vi "Parser.vi"() -> ()   [LabVIEW 2010]
panel:
  out "array of clusters 2":cluster{string[]}[](array[cluster])
  in  "Ring":u16(ring) items=["cp", "ct", "dd", "ep", "io", "ip", "pd", "pp", "ss", "st", "tp", "up", "vp"]
  out "Группы":string[](array[string])
  out "Параметры 2":T1(array[cluster])=[{"Имя"="cp1", "Группа"="cp", "Наименование"="Пропорциональный коэффициент контура тока", "Ед. изм"=0, "Список"="", "Адрес"=0, "Описание"="Параметр настройки ПИ-регулятора контура тока", "Мин"=0, "Макс"=100, "Сервис"=TRUE, "Только чтение"=FALSE, "Разработка"=FALSE, "К-во бит"=32, "Шаг"=12, "Обработка"=FALSE, "Макрос"=""}, {"Имя"="cp10", "Группа"="cp", "Наименование"="Номинальный ток", "Ед. изм"=5, "Список"="", "Адрес"=2069, "Описание"="", "Мин"=0, "Макс"=850, "Сервис"=TRUE, "Только чтение"=FALSE, "Разработка"=FALSE, "К-во бит"=32, "Шаг"=16, "Обработка"=TRUE, "Макрос"="macros cp10\n  ON_READ\n  READ cp3\n  cp3=cp3*5/2047\n  RETURN cp3\n  ON_WRITE\n  cp3=val*66\n  WRITE cp3\nend"}, {"Имя"="cp11", "Группа"="cp", "Наименование"="Коэффициент ФНЧ входного сигнала", "Ед. изм"=0, "Список"="", "Адрес"=2081, "Описание"="Коэффициент ФНЧ входного сигнала контура тока.", "Мин"=0, "Макс"=1, "Сервис"=TRUE, "Только чтение"=FALSE, "Разработка"=FALSE, "К-во бит"=32, "Шаг"=12, "Обработка"=FALSE, "Макрос"=""}, {"Имя"="cp12", "Группа"="cp", "Наименование"="Коэффициент ФНЧ сигнала ОС", "Ед. изм"=0, "Список"="", "Адрес"=2082, "Описание"="Коэффициент ФНЧ сигнала обратной связи контура тока.", "Мин"=0, "Макс"=1, "Сервис"=TRUE, "Только чтение"=FALSE, "Разработка"=FALSE, "К-во бит"=32, "Шаг"=12, "Обработка"=FALSE, "Макрос"=""}, {"Имя"="cp2", "Группа"="cp", "Наименование"="Интегральный коэффициент контура тока", "Ед. изм"=0, "Список"="", "Адрес"=2, "Описание"="Параметр настройки ПИ-регулятора контура тока", "Мин"=0, "Макс"=200, "Сервис"=TRUE, "Только чтение"=FALSE, "Разработка"=FALSE, "К-во бит"=32, "Шаг"=12, "Обработка"=FALSE, "Макрос"=""}, {"Имя"="cp3", "Группа"="cp", "Наименование"="Максимальный ток", "Ед. изм"=1, "Список"="", "Адрес"=4, "Описание"="Определять предельную величину тока допустимую для двигателя.", "Мин"=0, "Макс"=1500, "Сервис"=FALSE, "Только чтение"=FALSE, "Разработка"=FALSE, "К-во бит"=16, "Шаг"=0, "Обработка"=TRUE, "Макрос"="macros cp3\n  ON_READ\n  READ cp3\n  cp3=cp3*5/2047\n  RETURN cp3\n  ON_WRITE\n  cp3=val*2047/5\n  WRITE cp3\nend"}, {"Имя"="cp4", "Группа"="cp", "Наименование"="Максимальная скваженность ШИМ", "Ед. изм"=1, "Список"="", "Адрес"=5, "Описание"="3070 дискрет соответствует 100% заполнения", "Мин"=0, "Макс"=6150, "Сервис"=FALSE, "Только чтение"=FALSE, "Разработка"=FALSE, "К-во бит"=16, "Шаг"=0, "Обработка"=TRUE, "Макрос"="macros cp4\n  ON_READ\n  READ cp4\n  cp4=cp4*5/2500\n  RETURN cp4\n  ON_WRITE\n  cp4=val*2500/5\n  WRITE cp4\nend"}, {"Имя"="cp5", "Группа"="cp", "Наименование"="Состояние контура тока", "Ед. изм"=0, "Список"="0:Разомкнут\n2:Замкнут\n4:Прямое управление токами в обмотках\n5:Адаптивное упрваление\n6:Прямое раздельное управление токами в обмотках\n\r\n", "Адрес"=16, "Описание"="Обеспечивает замкнутое или разомкнутое регулирование контура тока. В стандартном режиме использования контур должен быть замкнут.", "Мин"=0, "Макс"=6, "Сервис"=FALSE, "Только чтение"=FALSE, "Разработка"=FALSE, "К-во бит"=16, "Шаг"=0, "Обработка"=FALSE, "Макрос"=""}, {"Имя"="cp6", "Группа"="cp", "Наименование"="Вырабатываемый момент", "Ед. изм"=0, "Список"="100:100%\n75:75%\n50:50%\n25:25%\n\r\n", "Адрес"=72, "Описание"="Параметр позволяет ограничить развиваемый момент", "Мин"=25, "Макс"=100, "Сервис"=FALSE, "Только чтение"=FALSE, "Разработка"=TRUE, "К-во бит"=16, "Шаг"=0, "Обработка"=FALSE, "Макрос"=""}, {"Имя"="cp7", "Группа"="cp", "Наименование"="Модуляция ШИМ сигнала", "Ед. изм"=0, "Список"="0:Выключена\n1:Включена\n\r\n", "Адрес"=83, "Описание"="Разрешает/запрещает подачу силового напряжения на обмотки двигателя", "Мин"=0, "Макс"=1, "Сервис"=FALSE, "Только чтение"=FALSE, "Разработка"=FALSE, "К-во бит"=16, "Шаг"=0, "Обработка"=FALSE, "Макрос"=""}, {"Имя"="cp8", "Группа"="cp", "Наименование"="Частота ШИМ сигнала", "Ед. изм"=12, "Список"="2500:40кГц\n5000:20кГц\n6250:16кГц\n12500:8кГц\n25000:4кГц\n\r\n", "Адрес"=96, "Описание"="Определяет частоту ШИМ сигнала и частоту работы контура тока. Влияет на КПД силовой части привода, а также качество работы контура тока. Для приводов серии СПШ частота всегда 40кГц. Влияет на параметр cp4.", "Мин"=-65535, "Макс"=65535, "Сервис"=FALSE, "Только чтение"=FALSE, "Разработка"=FALSE, "К-во бит"=16, "Шаг"=0, "Обработка"=FALSE, "Макрос"=""}, {"Имя"="cp9", "Группа"="cp", "Наименование"="Допустимая перегрузка", "Ед. изм"=13, "Список"="", "Адрес"=2068, "Описание"="Ограничение выделяемой мощности обмотками двигателя. Предотвращает повреждения обмоток. Реализует защитную функцию I2t", "Мин"=0, "Макс"=350, "Сервис"=TRUE, "Только чтение"=FALSE, "Разработка"=FALSE, "К-во бит"=32, "Шаг"=16, "Обработка"=FALSE, "Макрос"=""}, {"Имя"="ct1", "Группа"="ct", "Наименование"="Задание тока", "Ед. изм"=5, "Список"="", "Адрес"=512, "Описание"="Сигнал управления при разомкнутом контуре скорости и положения", "Мин"=-3500, "Макс"=3500, "Сервис"=FALSE, "Только чтение"=FALSE, "Разработка"=FALSE, "К-во бит"=16, "Шаг"=0, "Обработка"=TRUE, "Макрос"="macros ct1\n  ON_READ\n  READ ct1\n  ct1=ct1*5/2500\n  RETURN ct1\n  ON_WRITE\n  ct1=val*2500/5\n  WRITE ct1\nend"}, {"Имя"="ct2", "Группа"="ct", "Наименование"="Задание скорости", "Ед. изм"=4, "Список"="", "Адрес"=514, "Описание"="Сигнал управления при разомкнутом контуре положения", "Мин"=-12000, "Макс"=12000, "Сервис"=TRUE, "Только чтение"=FALSE, "Разработка"=FALSE, "К-во бит"=32, "Шаг"=12, "Обработка"=FALSE, "Макрос"=""}, {"Имя"="ct3", "Группа"="ct", "Наименование"="Задание положения", "Ед. изм"=6, "Список"="", "Адрес"=516, "Описание"="Сигнал управления при замкнутом контуре положения", "Мин"=-2147483647, "Макс"=2147483647, "Сервис"=FALSE, "Только чтение"=FALSE, "Разработка"=FALSE, "К-во бит"=32, "Шаг"=0, "Обработка"=FALSE, "Макрос"=""}, {"Имя"="dd1", "Группа"="dd", "Наименование"="Ток в обмотке 1", "Ед. изм"=5, "Список"="", "Адрес"=1024, "Описание"="Показывает ток, протекающий в обмотке двигателя", "Мин"=-5, "Макс"=5, "Сервис"=FALSE, "Только чтение"=TRUE, "Разработка"=FALSE, "К-во бит"=16, "Шаг"=0, "Обработка"=TRUE, "Макрос"="macros dd1\n  ON_READ\n  READ dd1\n  dd1=dd1*5/2047\n  RETURN dd1\n  ON_WRITE\n  dd1=val*2047/5\n  WRITE dd1\nend"}, {"Имя"="dd10", "Группа"="dd", "Наименование"="Температура внутри корпуса", "Ед. изм"=7, "Список"="", "Адрес"=1038, "Описание"="", "Мин"=-40, "Макс"=120, "Сервис"=FALSE, "Только чтение"=TRUE, "Разработка"=FALSE, "К-во бит"=16, "Шаг"=0, "Обработка"=TRUE, "Макрос"="macros dd10\n  ON_READ\n  READ dd10\n  dd10=dd10/128\n  RETURN dd10\n  ON_WRITE\n  dd10=val\n  WRITE dd10\nend"}, {"Имя"="dd11", "Группа"="dd", "Наименование"="Статус контроллера", "Ед. изм"=0, "Список"="0:Исправен\n1:Останов по команде\n2:Останов - высокое противодействующее усилие\n3:Останов - короткое замыкание\n4:Выход из температурного диапазона\n5:Повышенное силовое напряжение\n6:Низкое силовое напряжение\n7:Повышенное цифровое напряжение\n8:Низкое цифровое напряжение\n9:Cиловое напряжение превышает напряжение, установл. пользователем\n10:Останов - превышение допустимой перегрузки\n11:Останов - сработала защита IGBT модуля\n12:Останов - Ошибка поиска фазы по UVW трекам\n13:Останов - ошибка в настройках энкодера\n14: Останов - сбой в работе энкодера\n15: Останов - Ошибка фазировки двигателя\n\r\n", "Адрес"=1039, "Описание"="Привод в состоянии отработать задание только, если его статус \"Исправен\".", "Мин"=0, "Макс"=15, "Сервис"=FALSE, "Только чтение"=FALSE, "Разработка"=FALSE, "К-во бит"=16, "Шаг"=0, "Обработка"=FALSE, "Макрос"=""}, {"Имя"="dd12", "Группа"="dd", "Наименование"="Текущее напряжение питания", "Ед. изм"=8, "Список"="", "Адрес"=1040, "Описание"="", "Мин"=0, "Макс"=120, "Сервис"=FALSE, "Только чтение"=TRUE, "Разработка"=FALSE, "К-во бит"=16, "Шаг"=0, "Обработка"=TRUE, "Макрос"="macros dd12\n  ON_READ\n  READ dd12\n  dd12=dd12/21\n  RETURN dd12\n  ON_WRITE\n  dd12=val\n  WRITE dd12\nend"}, {"Имя"="dd13", "Группа"="dd", "Наименование"="Тестовый параметр 1", "Ед. изм"=0, "Список"="", "Адрес"=1041, "Описание"="Пока используется для индикации перехода на меандр вместо синуса. Параметр для разработчика", "Мин"=-65535, "Макс"=65535, "Сервис"=FALSE, "Только чтение"=TRUE, "Разработка"=TRUE, "К-во бит"=16, "Шаг"=0, "Обработка"=FALSE, "Макрос"=""}, {"Имя"="dd14", "Группа"="dd", "Наименование"="Тестовый параметр 2", "Ед. изм"=0, "Список"="", "Адрес"=1042, "Описание"="Пока используется для индикации сдвига фазы", "Мин"=-65535, "Макс"=65535, "Сервис"=FALSE, "Только чтение"=TRUE, "Разработка"=TRUE, "К-во бит"=16, "Шаг"=0, "Обработка"=FALSE, "Макрос"=""}, {"Имя"="dd15", "Группа"="dd", "Наименование"="Время выполнения команды интерпретатором", "Ед. изм"=11, "Список"="", "Адрес"=1043, "Описание"="Определяет максимальное время, которое интерпретатор затрачивает на выполнение команды в текущей программе.", "Мин"=0, "Макс"=2147483647, "Сервис"=FALSE, "Только чтение"=TRUE, "Разработка"=FALSE, "К-во бит"=32, "Шаг"=1, "Обработка"=TRUE, "Макрос"="macros dd15\n  ON_READ\n  READ dd15\n  dd15=dd15*25/1000\n  RETURN dd15\n  ON_WRITE\n  dd15=val\n  WRITE dd15\nend"}, {"Имя"="dd16", "Группа"="dd", "Наименование"="Время выполнения программы интерпретатором", "Ед. изм"=11, "Список"="", "Адрес"=1044, "Описание"="Определяет максимальное время, которое интерпретатор затрачивает на выполнение всей программы.", "Мин"=0, "Макс"=2147483647, "Сервис"=FALSE, "Только чтение"=TRUE, "Разработка"=FALSE, "К-во бит"=32, "Шаг"=1, "Обработка"=TRUE, "Макрос"="macros dd16\n  ON_READ\n  READ dd16\n  dd16=dd16*25/1000\n  RETURN dd16\n  ON_WRITE\n  dd16=val\n  WRITE dd16\nend"}, {"Имя"="dd17", "Группа"="dd", "Наименование"="Аналоговый вход 0", "Ед. изм"=1, "Список"="", "Адрес"=1045, "Описание"="", "Мин"=-65535, "Макс"=65535, "Сервис"=FALSE, "Только чтение"=TRUE, "Разработка"=FALSE, "К-во бит"=16, "Шаг"=0, "Обработка"=FALSE, "Макрос"=""}, {"Имя"="dd18", "Группа"="dd", "Наименование"="Аналоговый вход 1", "Ед. изм"=1, "Список"="", "Адрес"=1046, "Описание"="", "Мин"=-65535, "Макс"=65535, "Сервис"=FALSE, "Только чтение"=TRUE, "Разработка"=FALSE, "К-во бит"=16, "Шаг"=0, "Обработка"=FALSE, "Макрос"=""}, {"Имя"="dd19", "Группа"="dd", "Наименование"="Текущее цифровое напряжение", "Ед. изм"=8, "Список"="", "Адрес"=1047, "Описание"="", "Мин"=0, "Макс"=23, "Сервис"=FALSE, "Только чтение"=TRUE, "Разработка"=FALSE, "К-во бит"=16, "Шаг"=0, "Обработка"=TRUE, "Макрос"="macros dd19\n  ON_READ\n  READ dd19\n  dd19=dd19/178\n  RETURN dd19\n  ON_WRITE\n  dd19=val\n  WRITE dd19\nend"}, {"Имя"="dd2", "Группа"="dd", "Наименование"="Заданный ток в роторной системе координат", "Ед. изм"=5, "Список"="", "Адрес"=1026, "Описание"="Индицирует ток, который задан контуром скорости", "Мин"=-5, "Макс"=5, "Сервис"=FALSE, "Только чтение"=TRUE, "Разработка"=FALSE, "К-во бит"=16, "Шаг"=0, "Обработка"=TRUE, "Макрос"="macros dd2\n  ON_READ\n  READ dd2\n  dd2=dd2*5/2047\n  RETURN dd2\n  ON_WRITE\n  dd2=val*2047/5\n  WRITE dd2\nend"}, {"Имя"="dd20", "Группа"="dd", "Наименование"="Ошибка контура позиции", "Ед. изм"=6, "Список"="", "Адрес"=1048, "Описание"="", "Мин"=-2147483647, "Макс"=2147483647, "Сервис"=TRUE, "Только чтение"=TRUE, "Разработка"=FALSE, "К-во бит"=32, "Шаг"=10, "Обработка"=FALSE, "Макрос"=""}, {"Имя"="dd21", "Группа"="dd", "Наименование"="Ошибка контура скорости", "Ед. изм"=4, "Список"="", "Адрес"=1049, "Описание"="", "Мин"=-65535, "Макс"=65535, "Сервис"=FALSE, "Только чтение"=TRUE, "Разработка"=FALSE, "К-во бит"=16, "Шаг"=1, "Обработка"=FALSE, "Макрос"=""}, {"Имя"="dd22", "Группа"="dd", "Наименование"="Максимальное отклонение от траектории", "Ед. изм"=1, "Список"="", "Адрес"=1056, "Описание"="Определяет максимальную ошибку контура позиции зафиксированную при прохождении траектории.", "Мин"=0, "Макс"=65535, "Сервис"=FALSE, "Только чтение"=FALSE, "Разработка"=FALSE, "К-во бит"=16, "Шаг"=0, "Обработка"=FALSE, "Макрос"=""}, {"Имя"="dd23", "Группа"="dd", "Наименование"="Статус G декодера", "Ед. изм"=0, "Список"="0:Останов\n1:Начало\n2:Отработка\n3:Ожидание подтверждений\n4:Ошибка\n5:Выход в нуль\r\n", "Адрес"=1057, "Описание"="", "Мин"=0, "Макс"=5, "Сервис"=FALSE, "Только чтение"=TRUE, "Разработка"=TRUE, "К-во бит"=16, "Шаг"=0, "Обработка"=FALSE, "Макрос"=""}, {"Имя"="dd24", "Группа"="dd", "Наименование"="Текущий кадр G декодера", "Ед. изм"=0, "Список"="", "Адрес"=1058, "Описание"="", "Мин"=0, "Макс"=65535, "Сервис"=FALSE, "Только чтение"=TRUE, "Разработка"=TRUE, "К-во бит"=16, "Шаг"=0, "Обработка"=FALSE, "Макрос"=""}, {"Имя"="dd25", "Группа"="dd", "Наименование"="UVW треки", "Ед. изм"=0, "Список"="", "Адрес"=1059, "Описание"="Сигнал, считанный с UVW треков энкодера", "Мин"=0, "Макс"=16, "Сервис"=FALSE, "Только чтение"=TRUE, "Разработка"=FALSE, "К-во бит"=16, "Шаг"=0, "Обработка"=FALSE, "Макрос"=""}, {"Имя"="dd26", "Группа"="dd", "Наименование"="Текущая перегрузка", "Ед. изм"=13, "Список"="", "Адрес"=1060, "Описание"="Накомпленнае мощность, превышающая номинальные характеристики двигателя", "Мин"=0, "Макс"=100, "Сервис"=TRUE, "Только чтение"=TRUE, "Разработка"=FALSE, "К-во бит"=32, "Шаг"=16, "Обработка"=FALSE, "Макрос"=""}, {"Имя"="dd27", "Группа"="dd", "Наименование"="Ток в обмотке 3", "Ед. изм"=5, "Список"="", "Адрес"=1061, "Описание"="Показывает ток, протекающий в обмотке двигателя. Параметр действителен только для СПС.", "Мин"=-5, "Макс"=5, "Сервис"=FALSE, "Только чтение"=TRUE, "Разработка"=FALSE, "К-во бит"=16, "Шаг"=0, "Обработка"=TRUE, "Макрос"="macros dd27\n  ON_READ\n  READ dd1\n  dd1=dd1*5/2047\n  RETURN dd1\n  ON_WRITE\n  dd1=val*2047/5\n  WRITE dd1\nend"}, {"Имя"="dd28", "Группа"="dd", "Наименование"="Заданный ток в обмотке 3", "Ед. изм"=5, "Список"="", "Адрес"=1062, "Описание"="Заданный ток в обмотке 3. Действителен только для приводов серии СПС.", "Мин"=-2047, "Макс"=2047, "Сервис"=FALSE, "Только чтение"=FALSE, "Разработка"=FALSE, "К-во бит"=16, "Шаг"=0, "Обработка"=TRUE, "Макрос"="macros dd28\n  ON_READ\n  READ dd6\n  dd6=dd6/74\n  RETURN dd6\n  ON_WRITE\n  dd6=val*74\n  WRITE dd6\nend"}, {"Имя"="dd29", "Группа"="dd", "Наименование"="Ток потребления двигателя", "Ед. изм"=5, "Список"="", "Адрес"=1063, "Описание"="Параметр действителен только для СПС.", "Мин"=-5, "Макс"=5, "Сервис"=FALSE, "Только чтение"=TRUE, "Разработка"=FALSE, "К-во бит"=16, "Шаг"=0, "Обработка"=TRUE, "Макрос"="macros dd29\n  ON_READ\n  READ dd1\n  dd1=dd1/74\n  RETURN dd1\n  ON_WRITE\n  dd1=val*74\n  WRITE dd1\nend"}, {"Имя"="dd3", "Группа"="dd", "Наименование"="Ток в обмотке 2", "Ед. изм"=5, "Список"="", "Адрес"=1029, "Описание"="Индицирует ток, протекающий в обмотке двигателя", "Мин"=-5, "Макс"=5, "Сервис"=FALSE, "Только чтение"=TRUE, "Разработка"=FALSE, "К-во бит"=16, "Шаг"=0, "Обработка"=TRUE, "Макрос"="macros dd3\n  ON_READ\n  READ dd3\n  dd3=dd3*5/2047\n  RETURN dd3\n  ON_WRITE\n  dd3=val*2047/5\n  WRITE dd3\nend"}, {"Имя"="dd30", "Группа"="dd", "Наименование"="Разница между внешним и внутренним энкодерами", "Ед. изм"=1, "Список"="", "Адрес"=1064, "Описание"="Разница между внешним и внутренним энкодерами с приведением к разрешению внутреннего", "Мин"=-524286, "Макс"=524286, "Сервис"=TRUE, "Только чтение"=TRUE, "Разработка"=FALSE, "К-во бит"=32, "Шаг"=12, "Обработка"=FALSE, "Макрос"=""}, {"Имя"="dd31", "Группа"="dd", "Наименование"="Смещение фазы ослабления поля", "Ед. изм"=0, "Список"="", "Адрес"=1065, "Описание"="", "Мин"=0, "Макс"=0, "Сервис"=FALSE, "Только чтение"=TRUE, "Разработка"=FALSE, "К-во бит"=16, "Шаг"=0, "Обработка"=FALSE, "Макрос"=""}, {"Имя"="dd32", "Группа"="dd", "Наименование"="Задержка синхронизации", "Ед. изм"=14, "Список"="", "Адрес"=1066, "Описание"="Время между приемом команды упарвления и команды синхронизации. Параметр действителен только для приоводов с интерфейсом упарвления EtherCAT и при активизации управления от СЧПУ.", "Мин"=0, "Макс"=0, "Сервис"=FALSE, "Только чтение"=TRUE, "Разработка"=FALSE, "К-во бит"=32, "Шаг"=0, "Обработка"=FALSE, "Макрос"=""}, {"Имя"="dd33", "Группа"="dd", "Наименование"="Кол-во импульсов на сектор UVW сигнала", "Ед. изм"=6, "Список"="", "Адрес"=1067, "Описание"="Кол-во импульсов датчика позиции, приходящееся на текущий сектор UVW сигнала.", "Мин"=-2147483647, "Макс"=2147483647, "Сервис"=FALSE, "Только чтение"=TRUE, "Разработка"=FALSE, "К-во бит"=32, "Шаг"=0, "Обработка"=FALSE, "Макрос"=""}, {"Имя"="dd34", "Группа"="dd", "Наименование"="Ток в роторной системе координат", "Ед. изм"=1, "Список"="", "Адрес"=1068, "Описание"="Ток, пересчитанный в роторную систему координат. Данный сигнал является обратной связью на задание ddd2", "Мин"=-2147483647, "Макс"=2147483647, "Сервис"=TRUE, "Только чтение"=TRUE, "Разработка"=FALSE, "К-во бит"=32, "Шаг"=12, "Обработка"=FALSE, "Макрос"=""}, {"Имя"="dd4", "Группа"="dd", "Наименование"="Текущая скорость вращения", "Ед. изм"=4, "Список"="", "Адрес"=1032, "Описание"="", "Мин"=-5000, "Макс"=5000, "Сервис"=FALSE, "Только чтение"=TRUE, "Разработка"=FALSE, "К-во бит"=8, "Шаг"=12, "Обработка"=FALSE, "Макрос"=""}, {"Имя"="dd5", "Группа"="dd", "Наименование"="Заданная скорость вращения", "Ед. изм"=4, "Список"="", "Адрес"=1033, "Описание"="", "Мин"=-5000, "Макс"=5000, "Сервис"=FALSE, "Только чтение"=TRUE, "Разработка"=FALSE, "К-во бит"=16, "Шаг"=12, "Обработка"=FALSE, "Макрос"=""}, {"Имя"="dd6", "Группа"="dd", "Наименование"="Заданный ток в обмотке 1", "Ед. изм"=5, "Список"="", "Адрес"=1034, "Описание"="", "Мин"=-2047, "Макс"=2047, "Сервис"=FALSE, "Только чтение"=FALSE, "Разработка"=FALSE, "К-во бит"=16, "Шаг"=0, "Обработка"=TRUE, "Макрос"="macros dd6\n  ON_READ\n  READ dd6\n  dd6=dd6*5/2047\n  RETURN dd6\n  ON_WRITE\n  dd6=val*2047/5\n  WRITE dd6\nend"}, {"Имя"="dd7", "Группа"="dd", "Наименование"="Заданная позиция", "Ед. изм"=6, "Список"="", "Адрес"=1035, "Описание"="", "Мин"=-2147483647, "Макс"=2147483647, "Сервис"=FALSE, "Только чтение"=TRUE, "Разработка"=FALSE, "К-во бит"=32, "Шаг"=0, "Обработка"=FALSE, "Макрос"=""}, {"Имя"="dd8", "Группа"="dd", "Наименование"="Текущая позиция", "Ед. изм"=6, "Список"="", "Адрес"=1036, "Описание"="", "Мин"=-2147483647, "Макс"=2147483647, "Сервис"=FALSE, "Только чтение"=TRUE, "Разработка"=FALSE, "К-во бит"=32, "Шаг"=0, "Обработка"=FALSE, "Макрос"=""}, {"Имя"="dd9", "Группа"="dd", "Наименование"="Заданный ток в обмотке 2", "Ед. изм"=5, "Список"="", "Адрес"=1037, "Описание"="", "Мин"=-2047, "Макс"=2047, "Сервис"=FALSE, "Только чтение"=FALSE, "Разработка"=FALSE, "К-во бит"=16, "Шаг"=0, "Обработка"=TRUE, "Макрос"="macros dd9\n  ON_READ\n  READ dd9\n  dd9=dd9*5/2047\n  RETURN dd9\n  ON_WRITE\n  dd9=val*2047/5\n  WRITE dd9\nend"}, {"Имя"="ep1", "Группа"="ep", "Наименование"="Режим торможения", "Ед. изм"=0, "Список"="0:Торможение без контроля напряжения\n2:Торможение с контролем напряжения\n\r\n", "Адрес"=67, "Описание"="При торможении без контроля напряжения привод перейдет в аварийное состояние в момент превышения напряжением допустимого значения, установленным в параметре ep2.", "Мин"=0, "Макс"=2, "Сервис"=FALSE, "Только чтение"=FALSE, "Разработка"=FALSE, "К-во бит"=16, "Шаг"=0, "Обработка"=FALSE, "Макрос"=""}, {"Имя"="ep2", "Группа"="ep", "Наименование"="Максимальное напряжение", "Ед. изм"=8, "Список"="", "Адрес"=68, "Описание"="Максимальное допустимое напряжение, при котором привод должен переходить в состояние отключения.", "Мин"=0, "Макс"=280, "Сервис"=FALSE, "Только чтение"=FALSE, "Разработка"=FALSE, "К-во бит"=16, "Шаг"=0, "Обработка"=TRUE, "Макрос"="macros ep2\n  ON_READ\n  READ ep2\n  ep2=ep2/21\n  RETURN ep2\n  ON_WRITE\n  ep2=val*21\n  WRITE ep2\nend"}, {"Имя"="ep3", "Группа"="ep", "Наименование"="Ток поиска фазы", "Ед. изм"=1, "Список"="", "Адрес"=81, "Описание"="Определяет уровень тока, который устанавливается при поиске фазы. Ток задается в дискретах.", "Мин"=0, "Макс"=32000, "Сервис"=FALSE, "Только чтение"=FALSE, "Разработка"=FALSE, "К-во бит"=16, "Шаг"=1, "Обработка"=FALSE, "Макрос"=""}, {"Имя"="ep4", "Группа"="ep", "Наименование"="Время поиска фазы", "Ед. изм"=1, "Список"="", "Адрес"=82, "Описание"="Определяет время, в течение которого будет удерживаться ток ep3 при поиске фазы.", "Мин"=0, "Макс"=32000, "Сервис"=FALSE, "Только чтение"=FALSE, "Разработка"=FALSE, "К-во бит"=16, "Шаг"=1, "Обработка"=FALSE, "Макрос"=""}, {"Имя"="ep5", "Группа"="ep", "Наименование"="Максимальная температура", "Ед. изм"=7, "Список"="", "Адрес"=84, "Описание"="Указывает максимальную допустимую температуру внутри корпуса", "Мин"=25, "Макс"=85, "Сервис"=FALSE, "Только чтение"=FALSE, "Разработка"=FALSE, "К-во бит"=16, "Шаг"=1, "Обработка"=FALSE, "Макрос"=""}, {"Имя"="ep6", "Группа"="ep", "Наименование"="Период поиска фазы", "Ед. изм"=0, "Список"="0:Однопериодный\n1:1\n2:2\n3:3\n\r\n", "Адрес"=86, "Описание"="Один из трех периодов, во время которого привод может выполнять поиск фазы. В результате удается избежать перегрузки источника питания и выполнить корректный поиск фазы в приводах, между которыми имеется жесткая механическая связь.", "Мин"=0, "Макс"=3, "Сервис"=FALSE, "Только чтение"=FALSE, "Разработка"=FALSE, "К-во бит"=16, "Шаг"=1, "Обработка"=FALSE, "Макрос"=""}, {"Имя"="ep7", "Группа"="ep", "Наименование"="Функция контроля зазора", "Ед. изм"=0, "Список"="0:ВЫКЛ\n90:ВКЛ\n\r\n", "Адрес"=2075, "Описание"="Включение данной автоматически запускает внутреннюю программу контроля расстояния между инструментом и обрабатываемым листом.", "Мин"=0, "Макс"=90, "Сервис"=FALSE, "Только чтение"=FALSE, "Разработка"=FALSE, "К-во бит"=16, "Шаг"=1, "Обработка"=FALSE, "Макрос"=""}, {"Имя"="io0", "Группа"="io", "Наименование"="Порт ввода 0", "Ед. изм"=0, "Список"="", "Адрес"=2053, "Описание"="Значение порта ввода 0", "Мин"=0, "Макс"=1, "Сервис"=FALSE, "Только чтение"=FALSE, "Разработка"=FALSE, "К-во бит"=16, "Шаг"=0, "Обработка"=FALSE, "Макрос"=""}, {"Имя"="io1", "Группа"="io", "Наименование"="Порт ввода 1", "Ед. изм"=0, "Список"="", "Адрес"=2054, "Описание"="Значение порта ввода 1", "Мин"=0, "Макс"=1, "Сервис"=FALSE, "Только чтение"=FALSE, "Разработка"=FALSE, "К-во бит"=16, "Шаг"=0, "Обработка"=FALSE, "Макрос"=""}, {"Имя"="io10", "Группа"="io", "Наименование"="Режим порта ввода 2", "Ед. изм"=0, "Список"="0:Порт ввода общего назначения\n1:Порт ввода в режиме квадратурного счетчика\n2:Порт ввода в режиме счетчика Step/dir\n\r\n", "Адрес"=2063, "Описание"="Определяет режим работы порта ввода.", "Мин"=0, "Макс"=3, "Сервис"=FALSE, "Только чтение"=FALSE, "Разработка"=FALSE, "К-во бит"=16, "Шаг"=1, "Обработка"=FALSE, "Макрос"=""}, {"Имя"="io11", "Группа"="io", "Наименование"="Режим порта ввода 3", "Ед. изм"=0, "Список"="0:Порт ввода общего назначения\n1:Порт ввода в режиме квадратурного счетчика\n2:Порт ввода в режиме счетчика Step/dir\n\r\n", "Адрес"=2064, "Описание"="Определяет режим работы порта ввода.", "Мин"=0, "Макс"=3, "Сервис"=FALSE, "Только чтение"=FALSE, "Разработка"=FALSE, "К-во бит"=16, "Шаг"=1, "Обработка"=FALSE, "Макрос"=""}, {"Имя"="io12", "Группа"="io", "Наименование"="Режим порта вывода 0", "Ед. изм"=0, "Список"="0:Порт вывода общего назначения\n1:Порт вывода в режиме ШИМ\n\r\n", "Адрес"=2065, "Описание"="Определяет режим работы порта вывода.", "Мин"=0, "Макс"=3, "Сервис"=FALSE, "Только чтение"=FALSE, "Разработка"=FALSE, "К-во бит"=16, "Шаг"=1, "Обработка"=FALSE, "Макрос"=""}, {"Имя"="io13", "Группа"="io", "Наименование"="Режим порта вывода 1", "Ед. изм"=0, "Список"="0:Порт вывода общего назначения\n1:Порт вывода в режиме ШИМ\n\r\n", "Адрес"=2066, "Описание"="Определяет режим работы порта вывода.", "Мин"=0, "Макс"=3, "Сервис"=FALSE, "Только чтение"=FALSE, "Разработка"=FALSE, "К-во бит"=16, "Шаг"=1, "Обработка"=FALSE, "Макрос"=""}, {"Имя"="io14", "Группа"="io", "Наименование"="Счетчик импульсов", "Ед. изм"=0, "Список"="", "Адрес"=1807, "Описание"="Аппаратный счетчик импульсов,  которые приходят на входы In0 и In1. При этом порты должны быть настроены на соответствующий интерфейс (см. параметры io8 и io9).", "Мин"=-2147483647, "Макс"=2147483647, "Сервис"=FALSE, "Только чтение"=TRUE, "Разработка"=FALSE, "К-во бит"=32, "Шаг"=1, "Обработка"=FALSE, "Макрос"=""}, {"Имя"="io2", "Группа"="io", "Наименование"="Порт ввода 2", "Ед. изм"=0, "Список"="", "Адрес"=2055, "Описание"="Значение порта ввода 2", "Мин"=0, "Макс"=1, "Сервис"=FALSE, "Только чтение"=FALSE, "Разработка"=FALSE, "К-во бит"=16, "Шаг"=0, "Обработка"=FALSE, "Макрос"=""}, {"Имя"="io3", "Группа"="io", "Наименование"="Порт ввода 3", "Ед. изм"=0, "Список"="", "Адрес"=2056, "Описание"="Значение порта ввода 3", "Мин"=0, "Макс"=1, "Сервис"=FALSE, "Только чтение"=FALSE, "Разработка"=FALSE, "К-во бит"=16, "Шаг"=0, "Обработка"=FALSE, "Макрос"=""}, {"Имя"="io4", "Группа"="io", "Наименование"="Порт вывода 0", "Ед. изм"=0, "Список"="", "Адрес"=2057, "Описание"="Значение порта вывода 0", "Мин"=0, "Макс"=1, "Сервис"=FALSE, "Только чтение"=FALSE, "Разработка"=FALSE, "К-во бит"=16, "Шаг"=0, "Обработка"=FALSE, "Макрос"=""}, {"Имя"="io5", "Группа"="io", "Наименование"="Порт вывода 1", "Ед. изм"=0, "Список"="", "Адрес"=2058, "Описание"="Значение порта вывода 1", "Мин"=0, "Макс"=1, "Сервис"=FALSE, "Только чтение"=FALSE, "Разработка"=FALSE, "К-во бит"=16, "Шаг"=0, "Обработка"=FALSE, "Макрос"=""}, {"Имя"="io6", "Группа"="io", "Наименование"="PWM0", "Ед. изм"=0, "Список"="", "Адрес"=2059, "Описание"="Скваженность ШИМ сигнала, выводимого на порт вывода 0. Порт необходимо соответствующим образом настроить с помощью параметра: Режим работы порта вывода.", "Мин"=0, "Макс"=160, "Сервис"=FALSE, "Только чтение"=FALSE, "Разработка"=FALSE, "К-во бит"=16, "Шаг"=1, "Обработка"=FALSE, "Макрос"=""}, {"Имя"="io7", "Группа"="io", "Наименование"="PWM1", "Ед. изм"=0, "Список"="", "Адрес"=2060, "Описание"="Скваженность ШИМ сигнала, выводимого на порт вывода 1. Порт необходимо соответствующим образом настроить с помощью параметра: Режим работы порта вывода.", "Мин"=0, "Макс"=160, "Сервис"=FALSE, "Только чтение"=FALSE, "Разработка"=FALSE, "К-во бит"=16, "Шаг"=1, "Обработка"=FALSE, "Макрос"=""}, {"Имя"="io8", "Группа"="io", "Наименование"="Режим порта ввода 0", "Ед. изм"=0, "Список"="0:Порт ввода общего назначения\n1:Порт ввода в режиме квадратурного счетчика\n2:Порт ввода в режиме счетчика Step/dir\n\r\n", "Адрес"=2061, "Описание"="Определяет режим работы порта ввода.", "Мин"=0, "Макс"=3, "Сервис"=FALSE, "Только чтение"=FALSE, "Разработка"=FALSE, "К-во бит"=16, "Шаг"=1, "Обработка"=FALSE, "Макрос"=""}, {"Имя"="io9", "Группа"="io", "Наименование"="Режим порта ввода 1", "Ед. изм"=0, "Список"="0:Порт ввода общего назначения\n1:Порт ввода в режиме квадратурного счетчика\n2:Порт ввода в режиме счетчика Step/dir\n\r\n", "Адрес"=2062, "Описание"="Определяет режим работы порта ввода.", "Мин"=0, "Макс"=3, "Сервис"=FALSE, "Только чтение"=FALSE, "Разработка"=FALSE, "К-во бит"=16, "Шаг"=1, "Обработка"=FALSE, "Макрос"=""}, {"Имя"="ip0", "Группа"="ip", "Наименование"="Источник опорного сигнала", "Ед. изм"=0, "Список"="0:Интерфейс USB\n2:Интерфейс StepDir\n4:Аналоговый интерфейс\n5:Интерфейс CAN\n6:Квадратурный интерфейс\r\n", "Адрес"=23, "Описание"="Определяет интерфейс, по которому осуществляется ввод задания для привода.", "Мин"=0, "Макс"=6, "Сервис"=FALSE, "Только чтение"=FALSE, "Разработка"=FALSE, "К-во бит"=16, "Шаг"=0, "Обработка"=FALSE, "Макрос"=""}, {"Имя"="ip1", "Группа"="ip", "Наименование"="Коэффициент веса одной дискреты", "Ед. изм"=0, "Список"="", "Адрес"=24, "Описание"="Определяет количество импульсов датчика, на которые необходимо повернуть вал двигателя, при получении одной дискреты по интерфейсу Step/Dir, т.е. масштаб одного импульса", "Мин"=-4000, "Макс"=4000, "Сервис"=TRUE, "Только чтение"=FALSE, "Разработка"=FALSE, "К-во бит"=32, "Шаг"=10, "Обработка"=FALSE, "Макрос"=""}, {"Имя"="ip10", "Группа"="ip", "Наименование"="Статус шины CAN", "Ед. изм"=0, "Список"="0:Норма\n1:Неисправности на линии\n2:Ошибка передачи синхронизации слейву\n3:Ошибка - подтверждение не получено.\r\n", "Адрес"=56, "Описание"="Статус 2 - устанавливается, если мастер не может передать сообщение слейву в течение ip7", "Мин"=0, "Макс"=3, "Сервис"=FALSE, "Только чтение"=TRUE, "Разработка"=FALSE, "К-во бит"=16, "Шаг"=0, "Обработка"=FALSE, "Макрос"=""}, {"Имя"="ip11", "Группа"="ip", "Наименование"="Статус интерпретатора", "Ед. изм"=0, "Список"="0:Норма\n1:Смена банка программ\n2:Неизвестный параметр\n3:Неизвестная команда\n4:Останов\n5:STATUS_UNKNOWN_AL_OP\n6:STATUS_UNKNOWN_CMP_OP\n7:Загрузка программы\n8:STATUS_DEBUG_BREAK\n9:STATUS_DEBUG_WAIT_END_OF_CMD\n10:Неизвестная динамическая функция\n11:Старая версия программы\n12:Слишком много циклов\n77:Неправильное условие\n13:Не удалось найти Z метку\n78:Переполнение стека\n79:Попытка чтения пустого стека\n\r\n", "Адрес"=66, "Описание"="", "Мин"=0, "Макс"=12, "Сервис"=FALSE, "Только чтение"=TRUE, "Разработка"=FALSE, "К-во бит"=16, "Шаг"=1, "Обработка"=FALSE, "Макрос"=""}, {"Имя"="ip12", "Группа"="ip", "Наименование"="Мертвая зона аналоговых входов", "Ед. изм"=1, "Список"="", "Адрес"=69, "Описание"="Определяет зону нечувствительности аналоговых входов привода. При ручном управлении, например, с помощью джойстика, данный параметр позволяет исключить вращение вала при задании нулевой скорости.", "Мин"=0, "Макс"=250, "Сервис"=FALSE, "Только чтение"=FALSE, "Разработка"=FALSE, "К-во бит"=16, "Шаг"=0, "Обработка"=FALSE, "Макрос"=""}, {"Имя"="ip13", "Группа"="ip", "Наименование"="Ограничитель левый", "Ед. изм"=6, "Список"="", "Адрес"=87, "Описание"="Программный ограничитель позиции,  при достижении которой привод останавливается и воспринимает команду управления только в противоположную сторону.", "Мин"=-2147483647, "Макс"=2147483647, "Сервис"=FALSE, "Только чтение"=FALSE, "Разработка"=FALSE, "К-во бит"=32, "Шаг"=0, "Обработка"=FALSE, "Макрос"=""}, {"Имя"="ip14", "Группа"="ip", "Наименование"="Ограничитель правый", "Ед. изм"=6, "Список"="", "Адрес"=88, "Описание"="Программный ограничитель позиции,  при достижении которой привод останавливается и воспринимает команду управления только в противоположную сторону.", "Мин"=-2147483647, "Макс"=2147483647, "Сервис"=FALSE, "Только чтение"=FALSE, "Разработка"=FALSE, "К-во бит"=32, "Шаг"=0, "Обработка"=FALSE, "Макрос"=""}, {"Имя"="ip15", "Группа"="ip", "Наименование"="Скорость обмена по шине CAN", "Ед. изм"=0, "Список"="500:500 кБит/сек\n1000:1000 кБит/сек\n\r\n", "Адрес"=89, "Описание"="Определяет скорость обмена по шине CAN. При этом допустимая скорость определяется дальностью линии связи. На скорость 1000кБит максимальная дальность 60м, 500кБит - 120м", "Мин"=50, "Макс"=1000, "Сервис"=FALSE, "Только чтение"=FALSE, "Разработка"=FALSE, "К-во бит"=16, "Шаг"=0, "Обработка"=FALSE, "Макрос"=""}, {"Имя"="ip16", "Группа"="ip", "Наименование"="USB2CAN конвертор", "Ед. изм"=0, "Список"="0:Выкл\n2:Вкл\n\r\n", "Адрес"=97, "Описание"="Данная функция предназначена для облегчения подключения к группе приводов СПШ/СПС, которые объединены в рамках системы в одну сеть CAN. Чтобы работать со всеми приводами сети достаточно подключиться только к одному приводу по USB.", "Мин"=0, "Макс"=2, "Сервис"=FALSE, "Только чтение"=FALSE, "Разработка"=FALSE, "К-во бит"=16, "Шаг"=0, "Обработка"=FALSE, "Макрос"=""}, {"Имя"="ip17", "Группа"="ip", "Наименование"="Таймаут передачи синхронизации слейву", "Ед. изм"=9, "Список"="", "Адрес"=2048, "Описание"="Временной интервал, в течение которого мастер обязан передать синхронизацию слейву. По истечении этого времени параметр ip10 будет установлен в значение 1 или 2.", "Мин"=0, "Макс"=10000, "Сервис"=FALSE, "Только чтение"=FALSE, "Разработка"=FALSE, "К-во бит"=16, "Шаг"=25, "Обработка"=FALSE, "Макрос"=""}, {"Имя"="ip18", "Группа"="ip", "Наименование"="Таймаут передачи подтверждения мастеру от слейва", "Ед. изм"=9, "Список"="", "Адрес"=2049, "Описание"="Временной интервал, в течение которого слейв обязан передать подтверждение на команду синхронизации мастеру. По истечении этого времени параметр ip10 будет установлен в значение 3.", "Мин"=0, "Макс"=10000, "Сервис"=FALSE, "Только чтение"=FALSE, "Разработка"=FALSE, "К-во бит"=16, "Шаг"=25, "Обработка"=FALSE, "Макрос"=""}, {"Имя"="ip19", "Группа"="ip", "Наименование"="Данные CAN собщения 0", "Ед. изм"=0, "Список"="", "Адрес"=2077, "Описание"="4 младших байта последнего полученного CAN собщения", "Мин"=-2147483637, "Макс"=2147483646, "Сервис"=FALSE, "Только чтение"=FALSE, "Разработка"=FALSE, "К-во бит"=32, "Шаг"=0, "Обработка"=FALSE, "Макрос"=""}, {"Имя"="ip2", "Группа"="ip", "Наименование"="Текущий банк программы интерпретатора", "Ед. изм"=10, "Список"="0:0\n1:1\n2:2\n3:3\n4:4\n5:5\n6:6\n7:7\n255:Программа не выбрана\n\r\n", "Адрес"=26, "Описание"="Банк, из которой загружена программа на выполнение.", "Мин"=0, "Макс"=255, "Сервис"=FALSE, "Только чтение"=FALSE, "Разработка"=FALSE, "К-во бит"=16, "Шаг"=1, "Обработка"=FALSE, "Макрос"=""}, {"Имя"="ip20", "Группа"="ip", "Наименование"="Данные CAN собщения 1", "Ед. изм"=0, "Список"="", "Адрес"=2078, "Описание"="4 старших байта последнего полученного CAN собщения", "Мин"=-2147483637, "Макс"=2147483646, "Сервис"=FALSE, "Только чтение"=FALSE, "Разработка"=FALSE, "К-во бит"=32, "Шаг"=0, "Обработка"=FALSE, "Макрос"=""}, {"Имя"="ip3", "Группа"="ip", "Наименование"="Текущий банк чт/записи программ интерпретатора", "Ед. изм"=10, "Список"="0:0\n1:1\n2:2\n3:3\n4:4\n5:5\n6:6\n7:7\n255:Программа не выбрана\n\r\n", "Адрес"=27, "Описание"="", "Мин"=0, "Макс"=255, "Сервис"=FALSE, "Только чтение"=TRUE, "Разработка"=TRUE, "К-во бит"=16, "Шаг"=1, "Обработка"=FALSE, "Макрос"=""}, {"Имя"="ip4", "Группа"="ip", "Наименование"="Режим работы интерпретатора", "Ед. изм"=0, "Список"="0:Режим выполнения программы\n1:Режим отладки\n\r\n", "Адрес"=28, "Описание"="Режим работы интерпретатора", "Мин"=0, "Макс"=1, "Сервис"=FALSE, "Только чтение"=FALSE, "Разработка"=FALSE, "К-во бит"=16, "Шаг"=1, "Обработка"=FALSE, "Макрос"=""}, {"Имя"="ip5", "Группа"="ip", "Наименование"="Порт ввода вывода", "Ед. изм"=0, "Список"="", "Адрес"=29, "Описание"="Старший байт содержит содержимое порта вывода, младший - состояние линий ввода.", "Мин"=0, "Макс"=65535, "Сервис"=FALSE, "Только чтение"=FALSE, "Разработка"=FALSE, "К-во бит"=16, "Шаг"=0, "Обработка"=FALSE, "Макрос"=""}, {"Имя"="ip6", "Группа"="ip", "Наименование"="Смещение диапазона сигнала управления", "Ед. изм"=0, "Список"="", "Адрес"=48, "Описание"="Используется для корректировки диапазона регулирования входного сигнала (аналогового или Step\\Dir). Значение 2048 соответствует нулевой скорости при подаче на вход нулевого напряжения.", "Мин"=0, "Макс"=4096, "Сервис"=FALSE, "Только чтение"=FALSE, "Разработка"=FALSE, "К-во бит"=16, "Шаг"=0, "Обработка"=FALSE, "Макрос"=""}, {"Имя"="ip7", "Группа"="ip", "Наименование"="CAN адрес устройства", "Ед. изм"=0, "Список"="", "Адрес"=53, "Описание"="Адрес данного устройства в сети CAN", "Мин"=0, "Макс"=127, "Сервис"=FALSE, "Только чтение"=FALSE, "Разработка"=FALSE, "К-во бит"=16, "Шаг"=0, "Обработка"=FALSE, "Макрос"=""}, {"Имя"="ip8", "Группа"="ip", "Наименование"="CAN адрес удаленного узла", "Ед. изм"=0, "Список"="", "Адрес"=54, "Описание"="Адрес удаленного устройства в сети CAN, которое выступает в качестве мастера для данного устройства", "Мин"=0, "Макс"=127, "Сервис"=FALSE, "Только чтение"=FALSE, "Разработка"=FALSE, "К-во бит"=16, "Шаг"=0, "Обработка"=FALSE, "Макрос"=""}, {"Имя"="ip9", "Группа"="ip", "Наименование"="Режим синхронизации по CAN", "Ед. изм"=0, "Список"="0:Режим не выбран\n1:Режим мастер\n2:Режим слейв\n3:Режим контурного управления\n4:Синхронизация по команде SYNC\n\r\n", "Адрес"=55, "Описание"="В режиме мастер привод передает текущую позицию в CAN на адрес удаленного узла.", "Мин"=0, "Макс"=4, "Сервис"=FALSE, "Только чтение"=FALSE, "Разработка"=FALSE, "К-во бит"=16, "Шаг"=0, "Обработка"=FALSE, "Макрос"=""}, {"Имя"="pd1", "Группа"="pd", "Наименование"="Зона нечувствительности", "Ед. изм"=0, "Список"="", "Адрес"=2561, "Описание"="Параметр настройки ПИД-регулятора", "Мин"=0, "Макс"=10000, "Сервис"=TRUE, "Только чтение"=FALSE, "Разработка"=FALSE, "К-во бит"=32, "Шаг"=12, "Обработка"=FALSE, "Макрос"=""}, {"Имя"="pd10", "Группа"="pd", "Наименование"="Коэффициент форсирующей составляющей 0го порядка", "Ед. изм"=0, "Список"="", "Адрес"=2570, "Описание"="Параметр настройки ПИД-регулятора", "Мин"=0, "Макс"=10000, "Сервис"=TRUE, "Только чтение"=FALSE, "Разработка"=FALSE, "К-во бит"=32, "Шаг"=12, "Обработка"=FALSE, "Макрос"=""}, {"Имя"="pd11", "Группа"="pd", "Наименование"="Коэффициент форсирующей составляющей 1го порядка", "Ед. изм"=0, "Список"="", "Адрес"=2571, "Описание"="Параметр настройки ПИД-регулятора", "Мин"=0, "Макс"=10000, "Сервис"=TRUE, "Только чтение"=FALSE, "Разработка"=FALSE, "К-во бит"=32, "Шаг"=12, "Обработка"=FALSE, "Макрос"=""}, {"Имя"="pd12", "Группа"="pd", "Наименование"="Коэффициент форсирующей составляющей 2го порядка", "Ед. изм"=0, "Список"="", "Адрес"=2572, "Описание"="Параметр настройки ПИД-регулятора", "Мин"=0, "Макс"=10000, "Сервис"=TRUE, "Только чтение"=FALSE, "Разработка"=FALSE, "К-во бит"=32, "Шаг"=12, "Обработка"=FALSE, "Макрос"=""}, {"Имя"="pd13", "Группа"="pd", "Наименование"="Смещение сигнала управления", "Ед. изм"=0, "Список"="", "Адрес"=2573, "Описание"="Параметр настройки ПИД-регулятора", "Мин"=-524286, "Макс"=524287, "Сервис"=TRUE, "Только чтение"=FALSE, "Разработка"=FALSE, "К-во бит"=32, "Шаг"=12, "Обработка"=FALSE, "Макрос"=""}, {"Имя"="pd14", "Группа"="pd", "Наименование"="Ограничение выходного сигнала", "Ед. изм"=0, "Список"="", "Адрес"=2574, "Описание"="Параметр настройки ПИД-регулятора", "Мин"=0, "Макс"=524287, "Сервис"=TRUE, "Только чтение"=FALSE, "Разработка"=FALSE, "К-во бит"=32, "Шаг"=12, "Обработка"=FALSE, "Макрос"=""}, {"Имя"="pd15", "Группа"="pd", "Наименование"="Задание регулятора", "Ед. изм"=0, "Список"="", "Адрес"=2575, "Описание"="Параметр настройки ПИД-регулятора", "Мин"=-524286, "Макс"=524287, "Сервис"=TRUE, "Только чтение"=FALSE, "Разработка"=FALSE, "К-во бит"=32, "Шаг"=12, "Обработка"=FALSE, "Макрос"=""}, {"Имя"="pd16", "Группа"="pd", "Наименование"="Обратная связь", "Ед. изм"=0, "Список"="", "Адрес"=2576, "Описание"="Параметр настройки ПИД-регулятора", "Мин"=-524286, "Макс"=524287, "Сервис"=TRUE, "Только чтение"=TRUE, "Разработка"=FALSE, "К-во бит"=32, "Шаг"=12, "Обработка"=FALSE, "Макрос"=""}, {"Имя"="pd17", "Группа"="pd", "Наименование"="Ошибка", "Ед. изм"=0, "Список"="", "Адрес"=2577, "Описание"="Параметр настройки ПИД-регулятора", "Мин"=-524286, "Макс"=524287, "Сервис"=TRUE, "Только чтение"=TRUE, "Разработка"=FALSE, "К-во бит"=32, "Шаг"=12, "Обработка"=FALSE, "Макрос"=""}, {"Имя"="pd18", "Группа"="pd", "Наименование"="Коэффициент ФНЧ входного сигнала", "Ед. изм"=0, "Список"="", "Адрес"=2589, "Описание"="Параметр настройки ПИД-регулятора", "Мин"=0, "Макс"=1, "Сервис"=TRUE, "Только чтение"=FALSE, "Разработка"=FALSE, "К-во бит"=32, "Шаг"=12, "Обработка"=FALSE, "Макрос"=""}, {"Имя"="pd19", "Группа"="pd", "Наименование"="Коэффициент ФНЧ сигнала обратной связи", "Ед. изм"=0, "Список"="", "Адрес"=2590, "Описание"="Параметр настройки ПИД-регулятора", "Мин"=0, "Макс"=1, "Сервис"=TRUE, "Только чтение"=FALSE, "Разработка"=FALSE, "К-во бит"=32, "Шаг"=12, "Обработка"=FALSE, "Макрос"=""}, {"Имя"="pd2", "Группа"="pd", "Наименование"="Максимальная ошибка", "Ед. изм"=0, "Список"="", "Адрес"=2562, "Описание"="Параметр настройки ПИД-регулятора", "Мин"=0, "Макс"=524287, "Сервис"=TRUE, "Только чтение"=FALSE, "Разработка"=FALSE, "К-во бит"=32, "Шаг"=12, "Обработка"=FALSE, "Макрос"=""}, {"Имя"="pd3", "Группа"="pd", "Наименование"="Пропорциональный коэффициент", "Ед. изм"=0, "Список"="", "Адрес"=2563, "Описание"="Параметр настройки ПИД-регулятора", "Мин"=0, "Макс"=10000, "Сервис"=TRUE, "Только чтение"=FALSE, "Разработка"=FALSE, "К-во бит"=32, "Шаг"=12, "Обработка"=FALSE, "Макрос"=""}, {"Имя"="pd4", "Группа"="pd", "Наименование"="Интегральный коэффициент", "Ед. изм"=0, "Список"="", "Адрес"=2564, "Описание"="Параметр настройки ПИД-регулятора", "Мин"=0, "Макс"=10000, "Сервис"=TRUE, "Только чтение"=FALSE, "Разработка"=FALSE, "К-во бит"=32, "Шаг"=12, "Обработка"=FALSE, "Макрос"=""}, {"Имя"="pd5", "Группа"="pd", "Наименование"="Дифференциальный коэффициент", "Ед. изм"=0, "Список"="", "Адрес"=2565, "Описание"="Параметр настройки ПИД-регулятора", "Мин"=0, "Макс"=10000, "Сервис"=TRUE, "Только чтение"=FALSE, "Разработка"=FALSE, "К-во бит"=32, "Шаг"=12, "Обработка"=FALSE, "Макрос"=""}, {"Имя"="pd6", "Группа"="pd", "Наименование"="Ограничение интегральной составляющей", "Ед. изм"=0, "Список"="", "Адрес"=2566, "Описание"="Параметр настройки ПИД-регулятора", "Мин"=0, "Макс"=100000, "Сервис"=TRUE, "Только чтение"=FALSE, "Разработка"=FALSE, "К-во бит"=32, "Шаг"=12, "Обработка"=FALSE, "Макрос"=""}, {"Имя"="pd7", "Группа"="pd", "Наименование"="Ограничение дифференциальной составляющей", "Ед. изм"=0, "Список"="", "Адрес"=2567, "Описание"="Параметр настройки ПИД-регулятора", "Мин"=0, "Макс"=100000, "Сервис"=TRUE, "Только чтение"=FALSE, "Разработка"=FALSE, "К-во бит"=32, "Шаг"=12, "Обработка"=FALSE, "Макрос"=""}, {"Имя"="pd8", "Группа"="pd", "Наименование"="Ограничение форсирующей составляющей 1го порядка", "Ед. изм"=0, "Список"="", "Адрес"=2568, "Описание"="Параметр настройки ПИД-регулятора", "Мин"=0, "Макс"=524287, "Сервис"=TRUE, "Только чтение"=FALSE, "Разработка"=FALSE, "К-во бит"=32, "Шаг"=12, "Обработка"=FALSE, "Макрос"=""}, {"Имя"="pd9", "Группа"="pd", "Наименование"="Ограничение форсирующей составляющей 2го порядка", "Ед. изм"=0, "Список"="", "Адрес"=2569, "Описание"="Параметр настройки ПИД-регулятора", "Мин"=0, "Макс"=524287, "Сервис"=TRUE, "Только чтение"=FALSE, "Разработка"=FALSE, "К-во бит"=32, "Шаг"=12, "Обработка"=FALSE, "Макрос"=""}, {"Имя"="pp1", "Группа"="pp", "Наименование"="Пропорциональный коэффициент контура положения", "Ед. изм"=0, "Список"="", "Адрес"=11, "Описание"="Параметр настройки ПИ-регулятора контура позиционирования", "Мин"=0, "Макс"=10000, "Сервис"=TRUE, "Только чтение"=FALSE, "Разработка"=FALSE, "К-во бит"=32, "Шаг"=4, "Обработка"=FALSE, "Макрос"=""}, {"Имя"="pp10", "Группа"="pp", "Наименование"="Коэффициент форсирующей составляющей 2го порядка", "Ед. изм"=0, "Список"="", "Адрес"=2581, "Описание"="Параметр настройки ПИД-регулятора", "Мин"=0, "Макс"=100000, "Сервис"=TRUE, "Только чтение"=FALSE, "Разработка"=FALSE, "К-во бит"=32, "Шаг"=10, "Обработка"=FALSE, "Макрос"=""}, {"Имя"="pp11", "Группа"="pp", "Наименование"="Коэффициент микроинтерполяции", "Ед. изм"=0, "Список"="1:1\n2:2\n3:3\n4:4\n5:5\n\r\n", "Адрес"=2076, "Описание"="Коэффициент микроинтерполяции определяет кратность соотношения частот квантования СЧПУ и контура позиции привода. Коэффициент может принимать только значения 1, 2, 3, 4, 5. Если коэффициент равен 1, то частоты СЧПУ и привода равны.", "Мин"=1, "Макс"=5, "Сервис"=TRUE, "Только чтение"=FALSE, "Разработка"=FALSE, "К-во бит"=32, "Шаг"=10, "Обработка"=FALSE, "Макрос"=""}, {"Имя"="pp2", "Группа"="pp", "Наименование"="Интегральный коэффициент контура положения", "Ед. изм"=0, "Список"="", "Адрес"=12, "Описание"="Параметр настройки ПИ-регулятора контура позиционирования", "Мин"=0, "Макс"=30000, "Сервис"=TRUE, "Только чтение"=FALSE, "Разработка"=FALSE, "К-во бит"=32, "Шаг"=4, "Обработка"=FALSE, "Макрос"=""}, {"Имя"="pp3", "Группа"="pp", "Наименование"="Частота дискретизации контура положения", "Ед. изм"=0, "Список"="25:25\n50:50\n100:100\n200:200\n500:500\n1000:1000\n2000:2000\n3000:3000\n4000:4000\n5000:5000\n\r\n", "Адрес"=13, "Описание"="Определяет частоту обсчета контура позиции.", "Мин"=25, "Макс"=5000, "Сервис"=FALSE, "Только чтение"=FALSE, "Разработка"=FALSE, "К-во бит"=16, "Шаг"=0, "Обработка"=FALSE, "Макрос"=""}, {"Имя"="pp5", "Группа"="pp", "Наименование"="Состояние контура положения", "Ед. изм"=0, "Список"="0:Разомкнут\n2:Замкнут\n\r\n", "Адрес"=18, "Описание"="Обеспечивает замкнутое или разомкнутое регулирование контура позиции", "Мин"=0, "Макс"=2, "Сервис"=FALSE, "Только чтение"=FALSE, "Разработка"=FALSE, "К-во бит"=16, "Шаг"=0, "Обработка"=FALSE, "Макрос"=""}, {"Имя"="pp6", "Группа"="pp", "Наименование"="Ограничение интегральной составляющей контура позиции", "Ед. изм"=0, "Список"="", "Адрес"=65, "Описание"="Определяет максимальное значение, до которого может увеличиваться интегральная составляющая. По достижению этой величины интегральная составляющая удерживается константой.", "Мин"=0, "Макс"=15000, "Сервис"=TRUE, "Только чтение"=FALSE, "Разработка"=FALSE, "К-во бит"=32, "Шаг"=10, "Обработка"=FALSE, "Макрос"=""}, {"Имя"="pp7", "Группа"="pp", "Наименование"="Ограничение форсирующей составляющей 1го порядка", "Ед. изм"=0, "Список"="", "Адрес"=2578, "Описание"="Параметр настройки ПИД-регулятора", "Мин"=0, "Макс"=524287, "Сервис"=TRUE, "Только чтение"=FALSE, "Разработка"=FALSE, "К-во бит"=32, "Шаг"=10, "Обработка"=FALSE, "Макрос"=""}, {"Имя"="pp8", "Группа"="pp", "Наименование"="Ограничение форсирующей составляющей 2го порядка", "Ед. изм"=0, "Список"="", "Адрес"=2579, "Описание"="Параметр настройки ПИД-регулятора", "Мин"=0, "Макс"=524287, "Сервис"=TRUE, "Только чтение"=FALSE, "Разработка"=FALSE, "К-во бит"=32, "Шаг"=10, "Обработка"=FALSE, "Макрос"=""}, {"Имя"="pp9", "Группа"="pp", "Наименование"="Коэффициент форсирующей составляющей 1го порядка", "Ед. изм"=0, "Список"="", "Адрес"=2580, "Описание"="Параметр настройки ПИД-регулятора", "Мин"=0, "Макс"=100000, "Сервис"=TRUE, "Только чтение"=FALSE, "Разработка"=FALSE, "К-во бит"=32, "Шаг"=10, "Обработка"=FALSE, "Макрос"=""}, {"Имя"="si1", "Группа"="ss", "Наименование"="Смещение датчика тока 1", "Ед. изм"=0, "Список"="", "Адрес"=1536, "Описание"="Формула расчета I=cur1-511-si1", "Мин"=0, "Макс"=4096, "Сервис"=FALSE, "Только чтение"=FALSE, "Разработка"=TRUE, "К-во бит"=16, "Шаг"=0, "Обработка"=FALSE, "Макрос"=""}, {"Имя"="si2", "Группа"="ss", "Наименование"="Смещение датчика тока 2", "Ед. изм"=0, "Список"="", "Адрес"=1537, "Описание"="Формула расчета I=cur2-511-si2", "Мин"=0, "Макс"=4096, "Сервис"=FALSE, "Только чтение"=FALSE, "Разработка"=TRUE, "К-во бит"=16, "Шаг"=0, "Обработка"=FALSE, "Макрос"=""}, {"Имя"="ss1", "Группа"="ss", "Наименование"="Тестовый параметр", "Ед. изм"=0, "Список"="", "Адрес"=19, "Описание"="", "Мин"=-65535, "Макс"=65535, "Сервис"=FALSE, "Только чтение"=FALSE, "Разработка"=TRUE, "К-во бит"=16, "Шаг"=0, "Обработка"=FALSE, "Макрос"=""}, {"Имя"="ss10", "Группа"="ss", "Наименование"="Сообщение 2", "Ед. изм"=0, "Список"="1:Короткое замыкание\n2:Перегрев\n3:Повышенное напряжение\n4:Пониженное напряжение\n5:Перегрузка по току\n6:Произведена перезапись контроллера\n\r\n", "Адрес"=39, "Описание"="Журнал последних 8 сообщений", "Мин"=0, "Макс"=65535, "Сервис"=FALSE, "Только чтение"=FALSE, "Разработка"=FALSE, "К-во бит"=16, "Шаг"=0, "Обработка"=FALSE, "Макрос"=""}, {"Имя"="ss11", "Группа"="ss", "Наименование"="Сообщение 3", "Ед. изм"=0, "Список"="1:Короткое замыкание\n2:Перегрев\n3:Повышенное напряжение\n4:Пониженное напряжение\n5:Перегрузка по току\n6:Произведена перезапись контроллера\n\r\n", "Адрес"=40, "Описание"="Журнал последних 8 сообщений", "Мин"=0, "Макс"=65535, "Сервис"=FALSE, "Только чтение"=FALSE, "Разработка"=FALSE, "К-во бит"=16, "Шаг"=0, "Обработка"=FALSE, "Макрос"=""}, {"Имя"="ss12", "Группа"="ss", "Наименование"="Сообщение 4", "Ед. изм"=0, "Список"="1:Короткое замыкание\n2:Перегрев\n3:Повышенное напряжение\n4:Пониженное напряжение\n5:Перегрузка по току\n6:Произведена перезапись контроллера\n\r\n", "Адрес"=41, "Описание"="Журнал последних 8 сообщений", "Мин"=0, "Макс"=65535, "Сервис"=FALSE, "Только чтение"=FALSE, "Разработка"=FALSE, "К-во бит"=16, "Шаг"=0, "Обработка"=FALSE, "Макрос"=""}, {"Имя"="ss13", "Группа"="ss", "Наименование"="Сообщение 5", "Ед. изм"=0, "Список"="1:Короткое замыкание\n2:Перегрев\n3:Повышенное напряжение\n4:Пониженное напряжение\n5:Перегрузка по току\n6:Произведена перезапись контроллера\n\r\n", "Адрес"=42, "Описание"="Журнал последних 8 сообщений", "Мин"=0, "Макс"=65535, "Сервис"=FALSE, "Только чтение"=FALSE, "Разработка"=FALSE, "К-во бит"=16, "Шаг"=0, "Обработка"=FALSE, "Макрос"=""}, {"Имя"="ss14", "Группа"="ss", "Наименование"="Сообщение 6", "Ед. изм"=0, "Список"="1:Короткое замыкание\n2:Перегрев\n3:Повышенное напряжение\n4:Пониженное напряжение\n5:Перегрузка по току\n6:Произведена перезапись контроллера\n\r\n", "Адрес"=43, "Описание"="Журнал последних 8 сообщений", "Мин"=0, "Макс"=65535, "Сервис"=FALSE, "Только чтение"=FALSE, "Разработка"=FALSE, "К-во бит"=16, "Шаг"=0, "Обработка"=FALSE, "Макрос"=""}, {"Имя"="ss15", "Группа"="ss", "Наименование"="Сообщение 7", "Ед. изм"=0, "Список"="1:Короткое замыкание\n2:Перегрев\n3:Повышенное напряжение\n4:Пониженное напряжение\n5:Перегрузка по току\n6:Произведена перезапись контроллера\n\r\n", "Адрес"=44, "Описание"="Журнал последних 8 сообщений", "Мин"=0, "Макс"=65535, "Сервис"=FALSE, "Только чтение"=FALSE, "Разработка"=FALSE, "К-во бит"=16, "Шаг"=0, "Обработка"=FALSE, "Макрос"=""}, {"Имя"="ss16", "Группа"="ss", "Наименование"="Счетчик потерь синхронизации", "Ед. изм"=0, "Список"="", "Адрес"=2072, "Описание"="Показывает сколько было потеряно команд SYNC=0x02 по шине CAN. Счетчик работает только, если выбран один из возможных режимов синхронизации.", "Мин"=0, "Макс"=65535, "Сервис"=FALSE, "Только чтение"=FALSE, "Разработка"=FALSE, "К-во бит"=16, "Шаг"=0, "Обработка"=FALSE, "Макрос"=""}, {"Имя"="ss17", "Группа"="ss", "Наименование"="Счетчик потерь команд управления", "Ед. изм"=0, "Список"="", "Адрес"=2073, "Описание"="Показывает сколько было потеряно команд CAN_POS_COM=0x08 по шине CAN. Счетчик работает только, если выбран один из возможных режимов синхронизации.", "Мин"=0, "Макс"=65535, "Сервис"=FALSE, "Только чтение"=FALSE, "Разработка"=FALSE, "К-во бит"=16, "Шаг"=0, "Обработка"=FALSE, "Макрос"=""}, {"Имя"="ss18", "Группа"="ss", "Наименование"="Счетчик получения неизвестных команд", "Ед. изм"=0, "Список"="", "Адрес"=2074, "Описание"="Показывает сколько было получено неизвестных команд по шине CAN, которые помешали прохождению команд управления. Счетчик работает только, если выбран один из возможных режимов синхронизации.", "Мин"=0, "Макс"=65535, "Сервис"=FALSE, "Только чтение"=FALSE, "Разработка"=FALSE, "К-во бит"=16, "Шаг"=0, "Обработка"=FALSE, "Макрос"=""}, {"Имя"="ss2", "Группа"="ss", "Наименование"="Количество КЗ", "Ед. изм"=0, "Список"="", "Адрес"=31, "Описание"="Количество зафиксированных коротких замыканий", "Мин"=0, "Макс"=65535, "Сервис"=FALSE, "Только чтение"=FALSE, "Разработка"=FALSE, "К-во бит"=16, "Шаг"=0, "Обработка"=FALSE, "Макрос"=""}, {"Имя"="ss3", "Группа"="ss", "Наименование"="Количество превышений температуры", "Ед. изм"=0, "Список"="", "Адрес"=32, "Описание"="Количество зафиксированных превышений температуры", "Мин"=0, "Макс"=65535, "Сервис"=FALSE, "Только чтение"=FALSE, "Разработка"=FALSE, "К-во бит"=16, "Шаг"=0, "Обработка"=FALSE, "Макрос"=""}, {"Имя"="ss4", "Группа"="ss", "Наименование"="Количество перенапряжений", "Ед. изм"=0, "Список"="", "Адрес"=33, "Описание"="Количество зафиксированных перенапряжений", "Мин"=0, "Макс"=65535, "Сервис"=FALSE, "Только чтение"=FALSE, "Разработка"=FALSE, "К-во бит"=16, "Шаг"=0, "Обработка"=FALSE, "Макрос"=""}, {"Имя"="ss5", "Группа"="ss", "Наименование"="Количество недонапряжений", "Ед. изм"=0, "Список"="", "Адрес"=34, "Описание"="Количество зафиксированных случаев пониженного напряжений", "Мин"=0, "Макс"=65535, "Сервис"=FALSE, "Только чтение"=FALSE, "Разработка"=FALSE, "К-во бит"=16, "Шаг"=0, "Обработка"=FALSE, "Макрос"=""}, {"Имя"="ss6", "Группа"="ss", "Наименование"="Количество перегрузок", "Ед. изм"=0, "Список"="", "Адрес"=35, "Описание"="", "Мин"=0, "Макс"=65535, "Сервис"=FALSE, "Только чтение"=FALSE, "Разработка"=FALSE, "К-во бит"=16, "Шаг"=0, "Обработка"=FALSE, "Макрос"=""}, {"Имя"="ss7", "Группа"="ss", "Наименование"="Количество перепрогарммирований", "Ед. изм"=0, "Список"="", "Адрес"=36, "Описание"="", "Мин"=0, "Макс"=65535, "Сервис"=FALSE, "Только чтение"=FALSE, "Разработка"=FALSE, "К-во бит"=16, "Шаг"=0, "Обработка"=FALSE, "Макрос"=""}, {"Имя"="ss8", "Группа"="ss", "Наименование"="Сообщение 0", "Ед. изм"=0, "Список"="1:Короткое замыкание\n2:Перегрев\n3:Повышенное напряжение\n4:Пониженное напряжение\n5:Перегрузка по току\n6:Произведена перезапись контроллера\n\r\n", "Адрес"=37, "Описание"="Журнал последних 8 сообщений", "Мин"=0, "Макс"=65535, "Сервис"=FALSE, "Только чтение"=FALSE, "Разработка"=FALSE, "К-во бит"=16, "Шаг"=0, "Обработка"=FALSE, "Макрос"=""}, {"Имя"="ss9", "Группа"="ss", "Наименование"="Сообщение 1", "Ед. изм"=0, "Список"="1:Короткое замыкание\n2:Перегрев\n3:Повышенное напряжение\n4:Пониженное напряжение\n5:Перегрузка по току\n6:Произведена перезапись контроллера\n\r\n", "Адрес"=38, "Описание"="Журнал последних 8 сообщений", "Мин"=0, "Макс"=65535, "Сервис"=FALSE, "Только чтение"=FALSE, "Разработка"=FALSE, "К-во бит"=16, "Шаг"=0, "Обработка"=FALSE, "Макрос"=""}, {"Имя"="st1", "Группа"="st", "Наименование"="Разрешение", "Ед. изм"=6, "Список"="", "Адрес"=21, "Описание"="Разрешение датчика положения/скорости", "Мин"=0, "Макс"=2147483647, "Сервис"=FALSE, "Только чтение"=FALSE, "Разработка"=FALSE, "К-во бит"=32, "Шаг"=0, "Обработка"=FALSE, "Макрос"=""}, {"Имя"="st10", "Группа"="st", "Наименование"="Разрешение линейного энкодера", "Ед. изм"=1, "Список"="", "Адрес"=2071, "Описание"="Разрешение линейного энкодера на оборот вала двигателя", "Мин"=-524286, "Макс"=524286, "Сервис"=TRUE, "Только чтение"=FALSE, "Разработка"=FALSE, "К-во бит"=32, "Шаг"=12, "Обработка"=FALSE, "Макрос"=""}, {"Имя"="st11", "Группа"="st", "Наименование"="Разрешение на полюс двигателя", "Ед. изм"=1, "Список"="", "Адрес"=2083, "Описание"="Формуля для расчета:", "Мин"=1000, "Макс"=2098176, "Сервис"=FALSE, "Только чтение"=FALSE, "Разработка"=FALSE, "К-во бит"=32, "Шаг"=0, "Обработка"=FALSE, "Макрос"=""}, {"Имя"="st12", "Группа"="st", "Наименование"="Коэффициент деления энкодера", "Ед. изм"=0, "Список"="", "Адрес"=2084, "Описание"="Уменьшает разрешение датчика позиции (энкодера) в 2 или 4 раза. Если st12=1, то разрешение энкодера не уменьшается и соответствует физическому разрешению, выдаваемому самим датчиком.", "Мин"=1, "Макс"=4, "Сервис"=FALSE, "Только чтение"=FALSE, "Разработка"=FALSE, "К-во бит"=16, "Шаг"=0, "Обработка"=FALSE, "Макрос"=""}, {"Имя"="st13", "Группа"="st", "Наименование"="Инвертированные сигналы UVW", "Ед. изм"=0, "Список"="0:Нет\n21930:Да\n\r\n", "Адрес"=2085, "Описание"="UVW треки должны следовать в следующем порядке: 2, 3, 1, 5, 4, 6. Для таких датчиков st13=Нет. В некоторых датчиках сигналы идут с инверсией, в этом случае последовательность: 2, 6, 4, 5, 1, 3. Для таких датчиков st13=Да.", "Мин"=-2147483647, "Макс"=2147483647, "Сервис"=FALSE, "Только чтение"=FALSE, "Разработка"=FALSE, "К-во бит"=32, "Шаг"=0, "Обработка"=FALSE, "Макрос"=""}, {"Имя"="st14", "Группа"="st", "Наименование"="Автоматический поиск фазы", "Ед. изм"=0, "Список"="0:Фаза не найдена\n170:Запрос поиска фазы\n171:Ожидание завершения поиска фазы\n172:Ожидаем вращения в +\n173:Ожидаем вращения в -\n174:Ошибка поиска\n175:Поиск выполнен успешно\n\r\n", "Адрес"=2086, "Описание"="Параметр используется для отображения текущего состояния поиска фазы в автоматическом режиме. Поиск фазы позволяет настроить сервоусилитель на конкретный экземпляр двигателя.", "Мин"=0, "Макс"=175, "Сервис"=FALSE, "Только чтение"=TRUE, "Разработка"=FALSE, "К-во бит"=16, "Шаг"=0, "Обработка"=FALSE, "Макрос"=""}, {"Имя"="st2", "Группа"="st", "Наименование"="Версия ПО драйвера", "Ед. изм"=0, "Список"="", "Адрес"=22, "Описание"="Текущая версия программного обеспечения привода.", "Мин"=0, "Макс"=2147483647, "Сервис"=TRUE, "Только чтение"=FALSE, "Разработка"=FALSE, "К-во бит"=32, "Шаг"=12, "Обработка"=FALSE, "Макрос"=""}, {"Имя"="st3", "Группа"="st", "Наименование"="Уникальный идентификатор устройства", "Ед. изм"=0, "Список"="", "Адрес"=30, "Описание"="", "Мин"=0, "Макс"=2147483647, "Сервис"=FALSE, "Только чтение"=FALSE, "Разработка"=FALSE, "К-во бит"=32, "Шаг"=0, "Обработка"=FALSE, "Макрос"=""}, {"Имя"="st4", "Группа"="st", "Наименование"="Тип привода", "Ед. изм"=0, "Список"="1:СПШ10-23xx\n2:СПШ20-23xx\\1000Z\n4:СПШ20-23xx\\2000Z\n64:СПШ10-34xx\n128:СПШ20-34xx\\2000Z\n4096:СПШ20-34xx\\1000Z\n8192:СПС25-80007\n8193:СПС25-80016\n8194:СПС25-80025\n8195:СПС25-1100075\n8196:СПС30-хххх\n\r\n", "Адрес"=70, "Описание"="", "Мин"=1, "Макс"=65535, "Сервис"=FALSE, "Только чтение"=FALSE, "Разработка"=FALSE, "К-во бит"=16, "Шаг"=0, "Обработка"=FALSE, "Макрос"=""}, {"Имя"="st5", "Группа"="st", "Наименование"="Z метка", "Ед. изм"=0, "Список"="0:Нет\n1:Да\n\r\n", "Адрес"=71, "Описание"="Наличие или отсутствие у датчика позиции канала нуливой метки", "Мин"=0, "Макс"=1, "Сервис"=FALSE, "Только чтение"=FALSE, "Разработка"=FALSE, "К-во бит"=16, "Шаг"=0, "Обработка"=FALSE, "Макрос"=""}, {"Имя"="st6", "Группа"="st", "Наименование"="Нулевой сектор сигналов UVW", "Ед. изм"=0, "Список"="1:1\n2:2\n3:3\n4:4\n5:5\n6:6\n170:Выполнить инициализацию\n85:Не использовать UVW треки\n\r\n", "Адрес"=2050, "Описание"="Определяет сектор датчика UVW, в котором находится нуль двигателя. Если установить значение \"Выполнить инициализацию\", то при следующем запуске автоматически будет выполнена операция поиска сектора и смещения внутри сектора", "Мин"=0, "Макс"=170, "Сервис"=FALSE, "Только чтение"=FALSE, "Разработка"=FALSE, "К-во бит"=16, "Шаг"=0, "Обработка"=FALSE, "Макрос"=""}, {"Имя"="st7", "Группа"="st", "Наименование"="Сдвиг нуля внутри сектора сигналов UVW", "Ед. изм"=0, "Список"="", "Адрес"=2052, "Описание"="Определяет смещение внутри сектора датчика UVW, в котором находится нуль двигателя. Если установить значение \"Выполнить инициализацию\", то при следующем запуске автоматически будет выполнена операция поиска сектора и смещения внутри сектора", "Мин"=0, "Макс"=80000, "Сервис"=FALSE, "Только чтение"=FALSE, "Разработка"=FALSE, "К-во бит"=16, "Шаг"=0, "Обработка"=FALSE, "Макрос"=""}, {"Имя"="st8", "Группа"="st", "Наименование"="Тип энкодера", "Ед. изм"=0, "Список"="0:Инкрементальный\n1:Абсолютный\n\r\n", "Адрес"=98, "Описание"="", "Мин"=0, "Макс"=1, "Сервис"=FALSE, "Только чтение"=FALSE, "Разработка"=FALSE, "К-во бит"=32, "Шаг"=1, "Обработка"=FALSE, "Макрос"=""}, {"Имя"="st9", "Группа"="st", "Наименование"="Линейный энкодер", "Ед. изм"=0, "Список"="0:Нет\n1:Да\n\r\n", "Адрес"=2070, "Описание"="Если параметр установлен в Да, то будет использоваться внешний по отношению к приводу линейный энкодер для замыкания контура позиции. При этом контуры тока и скорости будут работать, по прежнему, от внутреннего энкодера.", "Мин"=0, "Макс"=1, "Сервис"=FALSE, "Только чтение"=FALSE, "Разработка"=FALSE, "К-во бит"=16, "Шаг"=0, "Обработка"=FALSE, "Макрос"=""}, {"Имя"="tp1", "Группа"="tp", "Наименование"="Режим осциллографа", "Ед. изм"=0, "Список"="0:Непрерывный режим\n1:Ступенька\n2:Синус\n3:Приращение скорости\n4:Синусоидальное изменение скорости\n5:Треугольное изменение позиции\n6:Измерение без задания\n7:Измерение без задания до принудительного останова\n8:Приращение момента\n\r\n", "Адрес"=1280, "Описание"="Режим сканирования динамических параметров (отображение выбранных параметров в процессе работы привода).", "Мин"=0, "Макс"=8, "Сервис"=FALSE, "Только чтение"=FALSE, "Разработка"=FALSE, "К-во бит"=16, "Шаг"=0, "Обработка"=FALSE, "Макрос"=""}, {"Имя"="tp2", "Группа"="tp", "Наименование"="Период опроса параметров", "Ед. изм"=9, "Список"="", "Адрес"=1282, "Описание"="Определяет интервал времени между запоминанием данных в массив в режимах 1-7.", "Мин"=25, "Макс"=25000, "Сервис"=FALSE, "Только чтение"=FALSE, "Разработка"=FALSE, "К-во бит"=16, "Шаг"=25, "Обработка"=FALSE, "Макрос"=""}, {"Имя"="tp3", "Группа"="tp", "Наименование"="Амплитуда задания положения", "Ед. изм"=0, "Список"="", "Адрес"=1284, "Описание"="Определяет величину приращения позиции в режиме осциллографа 1.", "Мин"=-2147483647, "Макс"=2147483647, "Сервис"=FALSE, "Только чтение"=FALSE, "Разработка"=FALSE, "К-во бит"=32, "Шаг"=0, "Обработка"=FALSE, "Макрос"=""}, {"Имя"="tp5", "Группа"="tp", "Наименование"="Период задающего воздействия", "Ед. изм"=9, "Список"="", "Адрес"=1285, "Описание"="Данный параметр определяет задержку введения задающего воздействия от начала сбора информации в режиме осциллографа 1 и 3.", "Мин"=25, "Макс"=800000, "Сервис"=FALSE, "Только чтение"=FALSE, "Разработка"=FALSE, "К-во бит"=16, "Шаг"=25, "Обработка"=TRUE, "Макрос"="macros tp5\n  ON_READ\n  READ tp5\n  tp5=tp5*25\n  RETURN tp5\n  ON_WRITE\n  tp5=val/25\n  WRITE tp5\n  ON_ERROR\n  err=100000000000\n  RETURN err\nend"}, {"Имя"="tp6", "Группа"="tp", "Наименование"="Амплитуда задания скорости", "Ед. изм"=4, "Список"="", "Адрес"=1286, "Описание"="Определяет величину приращения скорости в режиме осциллографа 3.", "Мин"=-14000, "Макс"=14000, "Сервис"=FALSE, "Только чтение"=FALSE, "Разработка"=FALSE, "К-во бит"=16, "Шаг"=0, "Обработка"=FALSE, "Макрос"=""}, {"Имя"="up0", "Группа"="up", "Наименование"="Переменная общего назначения 0", "Ед. изм"=0, "Список"="", "Адрес"=1792, "Описание"="Может использоваться для общих целей. Например, для запоминания длинны оси, приводимой в движение данным приводом и т.д.", "Мин"=-2147483647, "Макс"=2147483647, "Сервис"=FALSE, "Только чтение"=FALSE, "Разработка"=FALSE, "К-во бит"=32, "Шаг"=0, "Обработка"=FALSE, "Макрос"=""}, {"Имя"="up1", "Группа"="up", "Наименование"="Переменная общего назначения 1", "Ед. изм"=0, "Список"="", "Адрес"=1793, "Описание"="Может использоваться для общих целей. Например, для запоминания длинны оси, приводимой в движение данным приводом и т.д.", "Мин"=-2147483647, "Макс"=2147483647, "Сервис"=FALSE, "Только чтение"=FALSE, "Разработка"=FALSE, "К-во бит"=32, "Шаг"=0, "Обработка"=FALSE, "Макрос"=""}, {"Имя"="up10", "Группа"="up", "Наименование"="Z", "Ед. изм"=0, "Список"="", "Адрес"=1802, "Описание"="Переменная, используемая в ПЛК", "Мин"=-2147483647, "Макс"=2147483647, "Сервис"=FALSE, "Только чтение"=FALSE, "Разработка"=FALSE, "К-во бит"=32, "Шаг"=1, "Обработка"=FALSE, "Макрос"=""}, {"Имя"="up11", "Группа"="up", "Наименование"="EEPROM массив", "Ед. изм"=0, "Список"="", "Адрес"=1803, "Описание"="User EEPROM massive", "Мин"=-2147483647, "Макс"=2147483647, "Сервис"=FALSE, "Только чтение"=FALSE, "Разработка"=TRUE, "К-во бит"=32, "Шаг"=1, "Обработка"=FALSE, "Макрос"=""}, {"Имя"="up12", "Группа"="up", "Наименование"="EEPROM массив метаданных", "Ед. изм"=0, "Список"="", "Адрес"=1804, "Описание"="Metadata massive of params of motor", "Мин"=-2147483647, "Макс"=2147483647, "Сервис"=FALSE, "Только чтение"=FALSE, "Разработка"=TRUE, "К-во бит"=32, "Шаг"=1, "Обработка"=FALSE, "Макрос"=""}, {"Имя"="up13", "Группа"="up", "Наименование"="Значение текущего элемента EEPROM массива", "Ед. изм"=0, "Список"="", "Адрес"=1805, "Описание"="Отображает значение текущего элемента массива энергонезависимой памяти данных общего назначения.", "Мин"=-2147483647, "Макс"=2147483647, "Сервис"=FALSE, "Только чтение"=FALSE, "Разработка"=FALSE, "К-во бит"=32, "Шаг"=1, "Обработка"=FALSE, "Макрос"=""}, {"Имя"="up14", "Группа"="up", "Наименование"="Индекс текущего элемента EEPROM массива", "Ед. изм"=0, "Список"="", "Адрес"=1806, "Описание"="Отображает индекс текущего элемента массива энергонезависимой памяти данных общего назначения.", "Мин"=-2147483647, "Макс"=2147483647, "Сервис"=FALSE, "Только чтение"=FALSE, "Разработка"=FALSE, "К-во бит"=32, "Шаг"=1, "Обработка"=FALSE, "Макрос"=""}, {"Имя"="up15", "Группа"="up", "Наименование"="Значение счетчика импульсов", "Ед. изм"=0, "Список"="", "Адрес"=1807, "Описание"="Отображает значение счетчика импульсов, которые приходят на порты IN0, IN1, по протоколу Step\\Dir или по квадратурному протоколу. Счетчик активизирован только при выборе соответствующего протокола.", "Мин"=-2147483647, "Макс"=2147483647, "Сервис"=FALSE, "Только чтение"=FALSE, "Разработка"=FALSE, "К-во бит"=32, "Шаг"=1, "Обработка"=FALSE, "Макрос"=""}, {"Имя"="up16", "Группа"="up", "Наименование"="Среднее значение заданного тока", "Ед. изм"=0, "Список"="", "Адрес"=1808, "Описание"="Величина пропорциональна вырабатываемому приводом моменту, используется в программах для определения развиваемого момента.", "Мин"=-65535, "Макс"=65535, "Сервис"=FALSE, "Только чтение"=TRUE, "Разработка"=FALSE, "К-во бит"=16, "Шаг"=1, "Обработка"=FALSE, "Макрос"=""}, {"Имя"="up17", "Группа"="up", "Наименование"="Переменная общего назначения 8", "Ед. изм"=0, "Список"="", "Адрес"=1809, "Описание"="Может использоваться для общих целей. ВНИМАНИЕ! Данная переменная не записывается в энергонезависимую память.", "Мин"=-2147483647, "Макс"=2147483647, "Сервис"=FALSE, "Только чтение"=FALSE, "Разработка"=FALSE, "К-во бит"=32, "Шаг"=0, "Обработка"=FALSE, "Макрос"=""}, {"Имя"="up18", "Группа"="up", "Наименование"="Переменная общего назначения 9", "Ед. изм"=0, "Список"="", "Адрес"=1810, "Описание"="Может использоваться для общих целей. ВНИМАНИЕ! Данная переменная не записывается в энергонезависимую память.", "Мин"=-2147483647, "Макс"=2147483647, "Сервис"=FALSE, "Только чтение"=FALSE, "Разработка"=FALSE, "К-во бит"=32, "Шаг"=0, "Обработка"=FALSE, "Макрос"=""}, {"Имя"="up19", "Группа"="up", "Наименование"="Переменная общего назначения 10", "Ед. изм"=0, "Список"="", "Адрес"=1811, "Описание"="", "Мин"=-2147483647, "Макс"=2147483647, "Сервис"=FALSE, "Только чтение"=FALSE, "Разработка"=FALSE, "К-во бит"=32, "Шаг"=0, "Обработка"=FALSE, "Макрос"=""}, {"Имя"="up2", "Группа"="up", "Наименование"="Переменная общего назначения 2", "Ед. изм"=0, "Список"="", "Адрес"=1794, "Описание"="Может использоваться для общих целей. Например, для запоминания длинны оси, приводимой в движение данным приводом и т.д.", "Мин"=-2147483647, "Макс"=2147483647, "Сервис"=FALSE, "Только чтение"=FALSE, "Разработка"=FALSE, "К-во бит"=32, "Шаг"=0, "Обработка"=FALSE, "Макрос"=""}, {"Имя"="up20", "Группа"="up", "Наименование"="Переменная общего назначения 11", "Ед. изм"=0, "Список"="", "Адрес"=1812, "Описание"="", "Мин"=-2147483647, "Макс"=2147483647, "Сервис"=FALSE, "Только чтение"=FALSE, "Разработка"=FALSE, "К-во бит"=32, "Шаг"=0, "Обработка"=FALSE, "Макрос"=""}, {"Имя"="up21", "Группа"="up", "Наименование"="Переменная общего назначения 12", "Ед. изм"=0, "Список"="", "Адрес"=1813, "Описание"="Может использоваться для общих целей. ВНИМАНИЕ! Данная переменная не записывается в энергонезависимую память.", "Мин"=-2147483647, "Макс"=2147483647, "Сервис"=FALSE, "Только чтение"=FALSE, "Разработка"=FALSE, "К-во бит"=32, "Шаг"=0, "Обработка"=FALSE, "Макрос"=""}, {"Имя"="up22", "Группа"="up", "Наименование"="Переменная общего назначения 13", "Ед. изм"=0, "Список"="", "Адрес"=1814, "Описание"="Может использоваться для общих целей. ВНИМАНИЕ! Данная переменная не записывается в энергонезависимую память.", "Мин"=-2147483647, "Макс"=2147483647, "Сервис"=FALSE, "Только чтение"=FALSE, "Разработка"=FALSE, "К-во бит"=32, "Шаг"=0, "Обработка"=FALSE, "Макрос"=""}, {"Имя"="up23", "Группа"="up", "Наименование"="Переменная общего назначения  14", "Ед. изм"=0, "Список"="", "Адрес"=1815, "Описание"="Может использоваться для общих целей. ВНИМАНИЕ! Данная переменная не записывается в энергонезависимую память.", "Мин"=-2147483647, "Макс"=2147483647, "Сервис"=FALSE, "Только чтение"=FALSE, "Разработка"=FALSE, "К-во бит"=32, "Шаг"=0, "Обработка"=FALSE, "Макрос"=""}, {"Имя"="up24", "Группа"="up", "Наименование"="Переменная общего назначения 15", "Ед. изм"=0, "Список"="", "Адрес"=1816, "Описание"="Может использоваться для общих целей. ВНИМАНИЕ! Данная переменная не записывается в энергонезависимую память.", "Мин"=-2147483647, "Макс"=2147483647, "Сервис"=FALSE, "Только чтение"=FALSE, "Разработка"=FALSE, "К-во бит"=32, "Шаг"=0, "Обработка"=FALSE, "Макрос"=""}, {"Имя"="up3", "Группа"="up", "Наименование"="Переменная общего назначения 3", "Ед. изм"=0, "Список"="", "Адрес"=1795, "Описание"="Может использоваться для общих целей. Например, для запоминания длинны оси, приводимой в движение данным приводом и т.д.", "Мин"=-2147483647, "Макс"=2147483647, "Сервис"=FALSE, "Только чтение"=FALSE, "Разработка"=FALSE, "К-во бит"=32, "Шаг"=0, "Обработка"=FALSE, "Макрос"=""}, {"Имя"="up4", "Группа"="up", "Наименование"="Переменная общего назначения 4", "Ед. изм"=0, "Список"="", "Адрес"=1796, "Описание"="Может использоваться для общих целей. Например, для запоминания длинны оси, приводимой в движение данным приводом и т.д.", "Мин"=-2147483647, "Макс"=2147483647, "Сервис"=FALSE, "Только чтение"=FALSE, "Разработка"=FALSE, "К-во бит"=32, "Шаг"=0, "Обработка"=FALSE, "Макрос"=""}, {"Имя"="up5", "Группа"="up", "Наименование"="Переменная общего назначения 5", "Ед. изм"=0, "Список"="", "Адрес"=1797, "Описание"="Может использоваться для общих целей. Например, для запоминания длинны оси, приводимой в движение данным приводом и т.д.", "Мин"=-2147483647, "Макс"=2147483647, "Сервис"=FALSE, "Только чтение"=FALSE, "Разработка"=FALSE, "К-во бит"=32, "Шаг"=0, "Обработка"=FALSE, "Макрос"=""}, {"Имя"="up6", "Группа"="up", "Наименование"="Переменная общего назначения 6", "Ед. изм"=0, "Список"="", "Адрес"=1798, "Описание"="Может использоваться для общих целей. Например, для запоминания длинны оси, приводимой в движение данным приводом и т.д.", "Мин"=-2147483647, "Макс"=2147483647, "Сервис"=FALSE, "Только чтение"=FALSE, "Разработка"=FALSE, "К-во бит"=32, "Шаг"=0, "Обработка"=FALSE, "Макрос"=""}, {"Имя"="up7", "Группа"="up", "Наименование"="Переменная общего назначения 7", "Ед. изм"=0, "Список"="", "Адрес"=1799, "Описание"="Может использоваться для общих целей. Например, для запоминания длинны оси, приводимой в движение данным приводом и т.д.", "Мин"=-2147483647, "Макс"=2147483647, "Сервис"=FALSE, "Только чтение"=FALSE, "Разработка"=FALSE, "К-во бит"=32, "Шаг"=0, "Обработка"=FALSE, "Макрос"=""}, {"Имя"="up8", "Группа"="up", "Наименование"="X", "Ед. изм"=0, "Список"="", "Адрес"=1800, "Описание"="Переменная, используемая в ПЛК", "Мин"=-2147483647, "Макс"=2147483647, "Сервис"=FALSE, "Только чтение"=FALSE, "Разработка"=FALSE, "К-во бит"=32, "Шаг"=1, "Обработка"=FALSE, "Макрос"=""}, {"Имя"="up9", "Группа"="up", "Наименование"="Y", "Ед. изм"=0, "Список"="", "Адрес"=1801, "Описание"="Переменная, используемая в ПЛК", "Мин"=-2147483647, "Макс"=2147483647, "Сервис"=FALSE, "Только чтение"=FALSE, "Разработка"=FALSE, "К-во бит"=32, "Шаг"=1, "Обработка"=FALSE, "Макрос"=""}, {"Имя"="vp1", "Группа"="vp", "Наименование"="Пропорциональный коэффициент контура скорости", "Ед. изм"=0, "Список"="", "Адрес"=6, "Описание"="Параметр настройки ПИ-регулятора контура скорости", "Мин"=0, "Макс"=60000, "Сервис"=TRUE, "Только чтение"=FALSE, "Разработка"=FALSE, "К-во бит"=32, "Шаг"=12, "Обработка"=FALSE, "Макрос"=""}, {"Имя"="vp10", "Группа"="vp", "Наименование"="Начало резонансного диапазона 1", "Ед. изм"=4, "Список"="", "Адрес"=49, "Описание"="Если начало и конец диапазона равны, то диапазон не выбран.", "Мин"=0, "Макс"=8000, "Сервис"=FALSE, "Только чтение"=FALSE, "Разработка"=FALSE, "К-во бит"=16, "Шаг"=0, "Обработка"=TRUE, "Макрос"="macros vp10\n  ON_READ\n  READ vp10\n  if st1=0\n  READ st1\n  fi\n  if vp4=0\n  READ vp4\n  fi\n  if vp3=0\n  READ vp3\n  fi\n  vp10=round(60*vp10*vp4/(st1*vp3))\n  RETURN vp10\n  ON_WRITE\n  if st1=0\n  READ st1\n  fi\n  if vp4=0\n  READ vp4\n  fi\n  if vp3=0\n  READ vp3\n  fi\n  vp10=val*st1*vp3/(60*vp4)\n  WRITE vp10\n  ON_ERROR\n  vp10=100000000000000\n  RETURN vp10\nend"}, {"Имя"="vp11", "Группа"="vp", "Наименование"="Конец резонансного диапазона 1", "Ед. изм"=4, "Список"="", "Адрес"=50, "Описание"="Если начало и конец диапазона равны, то диапазон не выбран.", "Мин"=0, "Макс"=8000, "Сервис"=FALSE, "Только чтение"=FALSE, "Разработка"=FALSE, "К-во бит"=16, "Шаг"=0, "Обработка"=TRUE, "Макрос"="macros vp11\n  ON_READ\n  READ vp11\n  if st1=0\n  READ st1\n  fi\n  if vp4=0\n  READ vp4\n  fi\n  if vp3=0\n  READ vp3\n  fi\n  vp11=round(60*vp11*vp4/(st1*vp3))\n  RETURN vp11\n  ON_WRITE\n  if st1=0\n  READ st1\n  fi\n  if vp4=0\n  READ vp4\n  fi\n  if vp3=0\n  READ vp3\n  fi\n  vp11=val*st1*vp3/(60*vp4)\n  WRITE vp11\n  ON_ERROR\n  vp11=100000000000000\n  RETURN vp11\nend"}, {"Имя"="vp12", "Группа"="vp", "Наименование"="Начало резонансного диапазона 2", "Ед. изм"=4, "Список"="", "Адрес"=51, "Описание"="Если начало и конец диапазона равны, то диапазон не выбран.", "Мин"=0, "Макс"=8000, "Сервис"=FALSE, "Только чтение"=FALSE, "Разработка"=FALSE, "К-во бит"=16, "Шаг"=0, "Обработка"=TRUE, "Макрос"="macros vp12\n  ON_READ\n  READ vp12\n  if st1=0\n  READ st1\n  fi\n  if vp4=0\n  READ vp4\n  fi\n  if vp3=0\n  READ vp3\n  fi\n  vp12=round(60*vp12*vp4/(st1*vp3))\n  RETURN vp12\n  ON_WRITE\n  if st1=0\n  READ st1\n  fi\n  if vp4=0\n  READ vp4\n  fi\n  if vp3=0\n  READ vp3\n  fi\n  vp12=val*st1*vp3/(60*vp4)\n  WRITE vp12\n  ON_ERROR\n  vp12=100000000000000\n  RETURN vp12\nend"}, {"Имя"="vp13", "Группа"="vp", "Наименование"="Конец резонансного диапазона 2", "Ед. изм"=4, "Список"="", "Адрес"=52, "Описание"="Если начало и конец диапазона равны, то диапазон не выбран.", "Мин"=0, "Макс"=8000, "Сервис"=FALSE, "Только чтение"=FALSE, "Разработка"=FALSE, "К-во бит"=16, "Шаг"=0, "Обработка"=TRUE, "Макрос"="macros vp13\n  ON_READ\n  READ vp13\n  if st1=0\n  READ st1\n  fi\n  if vp4=0\n  READ vp4\n  fi\n  if vp3=0\n  READ vp3\n  fi\n  vp13=round(60*vp13*vp4/(st1*vp3))\n  RETURN vp13\n  ON_WRITE\n  if st1=0\n  READ st1\n  fi\n  if vp4=0\n  READ vp4\n  fi\n  if vp3=0\n  READ vp3\n  fi\n  vp13=val*st1*vp3/(60*vp4)\n  WRITE vp13\n  ON_ERROR\n  vp13=100000000000000\n  RETURN vp13\nend"}, {"Имя"="vp14", "Группа"="vp", "Наименование"="Номинальная скорость", "Ед. изм"=4, "Список"="", "Адрес"=57, "Описание"="Скорость, начиная с которой выполняется режим ослабления поля.", "Мин"=0, "Макс"=5000, "Сервис"=FALSE, "Только чтение"=FALSE, "Разработка"=FALSE, "К-во бит"=16, "Шаг"=0, "Обработка"=TRUE, "Макрос"="macros vp14\n  ON_READ\n  READ vp14\n  if st1=0\n  READ st1\n  fi\n  if vp4=0\n  READ vp4\n  fi\n  x=round(60*vp14*1000/4000)\n  RETURN x\n  ON_WRITE\n  if st1=0\n  READ st1\n  fi\n  if vp4=0\n  READ vp4\n  fi\n  vp14=val*4000/(60*1000)\n  WRITE vp14\n  ON_STREAM_REQ\n  READ st1\n  READ vp4\n  ON_ERROR\n  dd4=100000000000000\n  RETURN vp14\nend"}, {"Имя"="vp15", "Группа"="vp", "Наименование"="Авто расчет номинальной скорости", "Ед. изм"=0, "Список"="1:Да\n0:Нет\n\r\n", "Адрес"=64, "Описание"="Автоматический расчет номинальной скорости выполняется на основе текущего напряжения питания при включении привода.", "Мин"=0, "Макс"=1, "Сервис"=FALSE, "Только чтение"=FALSE, "Разработка"=FALSE, "К-во бит"=16, "Шаг"=0, "Обработка"=FALSE, "Макрос"=""}, {"Имя"="vp16", "Группа"="vp", "Наименование"="Дифференциальный коэффициент контура скорости", "Ед. изм"=0, "Список"="", "Адрес"=80, "Описание"="Параметр настройки ПИ-регулятора контура скорости", "Мин"=0, "Макс"=60000, "Сервис"=TRUE, "Только чтение"=FALSE, "Разработка"=FALSE, "К-во бит"=32, "Шаг"=12, "Обработка"=FALSE, "Макрос"=""}, {"Имя"="vp17", "Группа"="vp", "Наименование"="Рывок", "Ед. изм"=0, "Список"="", "Адрес"=99, "Описание"="Ограничивает вторую производную скорости. Параметр вступает в силу только при установки vp9 в значение 4", "Мин"=1, "Макс"=21470, "Сервис"=TRUE, "Только чтение"=FALSE, "Разработка"=FALSE, "К-во бит"=32, "Шаг"=10, "Обработка"=FALSE, "Макрос"=""}, {"Имя"="vp18", "Группа"="vp", "Наименование"="Зона нечувствительности входного сигнала", "Ед. изм"=0, "Список"="", "Адрес"=2582, "Описание"="Параметр настройки ПИ-регулятора контура скорости", "Мин"=0, "Макс"=60000, "Сервис"=TRUE, "Только чтение"=FALSE, "Разработка"=FALSE, "К-во бит"=32, "Шаг"=12, "Обработка"=FALSE, "Макрос"=""}, {"Имя"="vp19", "Группа"="vp", "Наименование"="Максимальная ошибка", "Ед. изм"=0, "Список"="", "Адрес"=2583, "Описание"="Параметр настройки ПИ-регулятора контура скорости", "Мин"=0, "Макс"=60000, "Сервис"=TRUE, "Только чтение"=FALSE, "Разработка"=FALSE, "К-во бит"=32, "Шаг"=12, "Обработка"=FALSE, "Макрос"=""}, {"Имя"="vp2", "Группа"="vp", "Наименование"="Интегральный коэффициент контура скорости", "Ед. изм"=0, "Список"="", "Адрес"=7, "Описание"="Параметр настройки ПИ-регулятора контура скорости", "Мин"=0, "Макс"=60000, "Сервис"=TRUE, "Только чтение"=FALSE, "Разработка"=FALSE, "К-во бит"=32, "Шаг"=12, "Обработка"=FALSE, "Макрос"=""}, {"Имя"="vp20", "Группа"="vp", "Наименование"="Ограничение форсирующей связи 1го порядка", "Ед. изм"=0, "Список"="", "Адрес"=2584, "Описание"="Параметр настройки ПИ-регулятора контура скорости", "Мин"=0, "Макс"=524287, "Сервис"=TRUE, "Только чтение"=FALSE, "Разработка"=FALSE, "К-во бит"=32, "Шаг"=12, "Обработка"=FALSE, "Макрос"=""}, {"Имя"="vp21", "Группа"="vp", "Наименование"="Ограничение форсирующей связи 2го порядка", "Ед. изм"=0, "Список"="", "Адрес"=2585, "Описание"="Параметр настройки ПИ-регулятора контура скорости", "Мин"=0, "Макс"=524287, "Сервис"=TRUE, "Только чтение"=FALSE, "Разработка"=FALSE, "К-во бит"=32, "Шаг"=12, "Обработка"=FALSE, "Макрос"=""}, {"Имя"="vp22", "Группа"="vp", "Наименование"="Коэффициент форсирующей связи 0го порядка", "Ед. изм"=0, "Список"="", "Адрес"=2586, "Описание"="Параметр настройки ПИ-регулятора контура скорости", "Мин"=0, "Макс"=60000, "Сервис"=TRUE, "Только чтение"=FALSE, "Разработка"=FALSE, "К-во бит"=32, "Шаг"=12, "Обработка"=FALSE, "Макрос"=""}, {"Имя"="vp23", "Группа"="vp", "Наименование"="Коэффициент форсирующей связи 1го порядка", "Ед. изм"=0, "Список"="", "Адрес"=2587, "Описание"="Параметр настройки ПИ-регулятора контура скорости", "Мин"=0, "Макс"=60000, "Сервис"=TRUE, "Только чтение"=FALSE, "Разработка"=FALSE, "К-во бит"=32, "Шаг"=12, "Обработка"=FALSE, "Макрос"=""}, {"Имя"="vp24", "Группа"="vp", "Наименование"="Коэффициент форсирующей связи 2го порядка", "Ед. изм"=0, "Список"="", "Адрес"=2588, "Описание"="Параметр настройки ПИ-регулятора контура скорости", "Мин"=0, "Макс"=60000, "Сервис"=TRUE, "Только чтение"=FALSE, "Разработка"=FALSE, "К-во бит"=32, "Шаг"=12, "Обработка"=FALSE, "Макрос"=""}, {"Имя"="vp25", "Группа"="vp", "Наименование"="Коэффициент ФНЧ входного сигнала", "Ед. изм"=0, "Список"="", "Адрес"=2079, "Описание"="Коэффициент ФНЧ входного сигнала контура скорости", "Мин"=0, "Макс"=1, "Сервис"=TRUE, "Только чтение"=FALSE, "Разработка"=FALSE, "К-во бит"=32, "Шаг"=12, "Обработка"=FALSE, "Макрос"=""}, {"Имя"="vp26", "Группа"="vp", "Наименование"="Коэффициент ФНЧ сигнала обратной связи", "Ед. изм"=0, "Список"="", "Адрес"=2080, "Описание"="Коэффициент ФНЧ сигнала обратной связи контура скорости", "Мин"=0, "Макс"=1, "Сервис"=TRUE, "Только чтение"=FALSE, "Разработка"=FALSE, "К-во бит"=32, "Шаг"=12, "Обработка"=FALSE, "Макрос"=""}, {"Имя"="vp3", "Группа"="vp", "Наименование"="Коэффициент обратной связи по скорости", "Ед. изм"=0, "Список"="", "Адрес"=8, "Описание"="Определяет масштаб датчика скорости", "Мин"=-1, "Макс"=1, "Сервис"=TRUE, "Только чтение"=FALSE, "Разработка"=FALSE, "К-во бит"=32, "Шаг"=12, "Обработка"=FALSE, "Макрос"=""}, {"Имя"="vp4", "Группа"="vp", "Наименование"="Частота дискретизации контура скорости", "Ед. изм"=0, "Список"="100:100\n 200:200\n 500:500\n 1000:1000\n 2000:2000\n 3000:3000\n 4000:4000\n 5000:5000\n\r\n", "Адрес"=9, "Описание"="Определяет частоту обсчета контура скорости", "Мин"=100, "Макс"=5000, "Сервис"=FALSE, "Только чтение"=FALSE, "Разработка"=FALSE, "К-во бит"=16, "Шаг"=0, "Обработка"=FALSE, "Макрос"=""}, {"Имя"="vp5", "Группа"="vp", "Наименование"="Ускорение", "Ед. изм"=2, "Список"="", "Адрес"=10, "Описание"="Определяет динамику контура скорости", "Мин"=1, "Макс"=2000000, "Сервис"=TRUE, "Только чтение"=FALSE, "Разработка"=FALSE, "К-во бит"=32, "Шаг"=10, "Обработка"=FALSE, "Макрос"=""}, {"Имя"="vp6", "Группа"="vp", "Наименование"="Максимальное время выхода на номинальный режим", "Ед. изм"=3, "Список"="0:Не ограничено\n1:1\n2:2\n3:3\n4:4\n5:5\n6:6\n7:7\n8:8\n9:9\n10:10\n11:11\n12:12\n13:13\n14:14\n15:15\n16:16\n17:17\n18:18\n19:19\n20:20\n21:21\n22:22\n23:23\n24:24\n25:25\n26:26\n27:27\n28:28\n29:29\n30:30\r\n", "Адрес"=14, "Описание"="Время, по истечению которого привод переходит в состояние останова, если не достигнута заданная скорость", "Мин"=0, "Макс"=30, "Сервис"=FALSE, "Только чтение"=FALSE, "Разработка"=FALSE, "К-во бит"=16, "Шаг"=1, "Обработка"=TRUE, "Макрос"="macros vp6\n  ON_READ\n  READ vp6\n  if vp4=0\n  READ vp4\n  fi\n  vp6=vp6/vp4\n  RETURN vp6\n  ON_WRITE\n  if vp4=0\n  READ vp4\n  fi\n  vp6=val*vp4\n  WRITE vp6\n  ON_ERROR\n  vp6=100000000000000\n  RETURN vp6\nend"}, {"Имя"="vp7", "Группа"="vp", "Наименование"="Состояние контура скорости", "Ед. изм"=0, "Список"="0:Разомкнут\n2:Замкнут\n\r\n", "Адрес"=17, "Описание"="Обеспечивает замкнутое или разомкнутое регулирование контура скорости. Контур должен быть замкнут в режиме управления скоростью привода и в режиме управления позицией.", "Мин"=0, "Макс"=2, "Сервис"=FALSE, "Только чтение"=FALSE, "Разработка"=FALSE, "К-во бит"=16, "Шаг"=0, "Обработка"=FALSE, "Макрос"=""}, {"Имя"="vp8", "Группа"="vp", "Наименование"="Максимальная скорость вращения", "Ед. изм"=4, "Список"="", "Адрес"=20, "Описание"="Ограничение максимальной скорости вращения привода.", "Мин"=0, "Макс"=8000, "Сервис"=TRUE, "Только чтение"=FALSE, "Разработка"=FALSE, "К-во бит"=32, "Шаг"=12, "Обработка"=FALSE, "Макрос"=""}, {"Имя"="vp9", "Группа"="vp", "Наименование"="Динамический режим", "Ед. изм"=0, "Список"="0:Режим плавного разгона/торможения\n2:Режим с максимальной динамикой\n3:Режим G декодирования\n4:S кривая\n\r\n", "Адрес"=15, "Описание"="Включает или отключает внутренний интерполятор. В режиме управления приводов от внешнего контроллера, например, от ЧПУ, привод должен находиться в режиме с максимальной динамикой. Режим G декодирования позволяет реализовать контурное управление непосредственно группой приводов без использования внешнего контроллера.", "Мин"=0, "Макс"=4, "Сервис"=FALSE, "Только чтение"=FALSE, "Разработка"=FALSE, "К-во бит"=16, "Шаг"=0, "Обработка"=FALSE, "Макрос"=""}] {"Ед. изм" items=["", "дискрет", "об/(сек^2)", "сек", "об/мин", "А", "имп.", "град.", "В", "мксек", "Банк", "мсек", "кГц", "А2сек", "nсек"]; "Адрес" format="%04x"}
  out "Параметры":T1(array[cluster])=[{"Имя"="cp1", "Группа"="cp", "Наименование"="Пропорциональный коэффициент контура тока", "Ед. изм"=0, "Список"="", "Адрес"=0, "Описание"="Параметр настройки ПИ-регулятора контура тока", "Мин"=0, "Макс"=100, "Сервис"=TRUE, "Только чтение"=FALSE, "Разработка"=FALSE, "К-во бит"=32, "Шаг"=12, "Обработка"=FALSE, "Макрос"=""}, {"Имя"="cp2", "Группа"="cp", "Наименование"="Интегральный коэффициент контура тока", "Ед. изм"=0, "Список"="", "Адрес"=2, "Описание"="Параметр настройки ПИ-регулятора контура тока", "Мин"=0, "Макс"=200, "Сервис"=TRUE, "Только чтение"=FALSE, "Разработка"=FALSE, "К-во бит"=32, "Шаг"=12, "Обработка"=FALSE, "Макрос"=""}, {"Имя"="cp3", "Группа"="cp", "Наименование"="Максимальный ток", "Ед. изм"=1, "Список"="", "Адрес"=4, "Описание"="Определять предельную величину тока допустимую для двигателя.", "Мин"=0, "Макс"=1500, "Сервис"=FALSE, "Только чтение"=FALSE, "Разработка"=FALSE, "К-во бит"=16, "Шаг"=0, "Обработка"=TRUE, "Макрос"="macros cp3\n  ON_READ\n  READ cp3\n  cp3=cp3*5/2047\n  RETURN cp3\n  ON_WRITE\n  cp3=val*2047/5\n  WRITE cp3\nend"}, {"Имя"="cp4", "Группа"="cp", "Наименование"="Максимальная скваженность ШИМ", "Ед. изм"=1, "Список"="", "Адрес"=5, "Описание"="3070 дискрет соответствует 100% заполнения", "Мин"=0, "Макс"=6150, "Сервис"=FALSE, "Только чтение"=FALSE, "Разработка"=FALSE, "К-во бит"=16, "Шаг"=0, "Обработка"=TRUE, "Макрос"="macros cp4\n  ON_READ\n  READ cp4\n  cp4=cp4*5/2500\n  RETURN cp4\n  ON_WRITE\n  cp4=val*2500/5\n  WRITE cp4\nend"}, {"Имя"="vp1", "Группа"="vp", "Наименование"="Пропорциональный коэффициент контура скорости", "Ед. изм"=0, "Список"="", "Адрес"=6, "Описание"="Параметр настройки ПИ-регулятора контура скорости", "Мин"=0, "Макс"=60000, "Сервис"=TRUE, "Только чтение"=FALSE, "Разработка"=FALSE, "К-во бит"=32, "Шаг"=12, "Обработка"=FALSE, "Макрос"=""}, {"Имя"="vp2", "Группа"="vp", "Наименование"="Интегральный коэффициент контура скорости", "Ед. изм"=0, "Список"="", "Адрес"=7, "Описание"="Параметр настройки ПИ-регулятора контура скорости", "Мин"=0, "Макс"=60000, "Сервис"=TRUE, "Только чтение"=FALSE, "Разработка"=FALSE, "К-во бит"=32, "Шаг"=12, "Обработка"=FALSE, "Макрос"=""}, {"Имя"="vp16", "Группа"="vp", "Наименование"="Дифференциальный коэффициент контура скорости", "Ед. изм"=0, "Список"="", "Адрес"=80, "Описание"="Параметр настройки ПИ-регулятора контура скорости", "Мин"=0, "Макс"=60000, "Сервис"=TRUE, "Только чтение"=FALSE, "Разработка"=FALSE, "К-во бит"=32, "Шаг"=12, "Обработка"=FALSE, "Макрос"=""}, {"Имя"="vp3", "Группа"="vp", "Наименование"="Коэффициент обратной связи по скорости", "Ед. изм"=0, "Список"="", "Адрес"=8, "Описание"="Определяет масштаб датчика скорости", "Мин"=-1, "Макс"=1, "Сервис"=TRUE, "Только чтение"=FALSE, "Разработка"=FALSE, "К-во бит"=32, "Шаг"=12, "Обработка"=FALSE, "Макрос"=""}, {"Имя"="vp4", "Группа"="vp", "Наименование"="Частота дискретизации контура скорости", "Ед. изм"=0, "Список"="100:100\n 200:200\n 500:500\n 1000:1000\n 2000:2000\n 3000:3000\n 4000:4000\n 5000:5000\n\r\n", "Адрес"=9, "Описание"="Определяет частоту обсчета контура скорости", "Мин"=100, "Макс"=5000, "Сервис"=FALSE, "Только чтение"=FALSE, "Разработка"=FALSE, "К-во бит"=16, "Шаг"=0, "Обработка"=FALSE, "Макрос"=""}, {"Имя"="vp5", "Группа"="vp", "Наименование"="Ускорение", "Ед. изм"=2, "Список"="", "Адрес"=10, "Описание"="Определяет динамику контура скорости", "Мин"=1, "Макс"=2000000, "Сервис"=TRUE, "Только чтение"=FALSE, "Разработка"=FALSE, "К-во бит"=32, "Шаг"=10, "Обработка"=FALSE, "Макрос"=""}, {"Имя"="pp1", "Группа"="pp", "Наименование"="Пропорциональный коэффициент контура положения", "Ед. изм"=0, "Список"="", "Адрес"=11, "Описание"="Параметр настройки ПИ-регулятора контура позиционирования", "Мин"=0, "Макс"=10000, "Сервис"=TRUE, "Только чтение"=FALSE, "Разработка"=FALSE, "К-во бит"=32, "Шаг"=4, "Обработка"=FALSE, "Макрос"=""}, {"Имя"="pp2", "Группа"="pp", "Наименование"="Интегральный коэффициент контура положения", "Ед. изм"=0, "Список"="", "Адрес"=12, "Описание"="Параметр настройки ПИ-регулятора контура позиционирования", "Мин"=0, "Макс"=30000, "Сервис"=TRUE, "Только чтение"=FALSE, "Разработка"=FALSE, "К-во бит"=32, "Шаг"=4, "Обработка"=FALSE, "Макрос"=""}, {"Имя"="pp3", "Группа"="pp", "Наименование"="Частота дискретизации контура положения", "Ед. изм"=0, "Список"="25:25\n50:50\n100:100\n200:200\n500:500\n1000:1000\n2000:2000\n3000:3000\n4000:4000\n5000:5000\n\r\n", "Адрес"=13, "Описание"="Определяет частоту обсчета контура позиции.", "Мин"=25, "Макс"=5000, "Сервис"=FALSE, "Только чтение"=FALSE, "Разработка"=FALSE, "К-во бит"=16, "Шаг"=0, "Обработка"=FALSE, "Макрос"=""}, {"Имя"="vp6", "Группа"="vp", "Наименование"="Максимальное время выхода на номинальный режим", "Ед. изм"=3, "Список"="0:Не ограничено\n1:1\n2:2\n3:3\n4:4\n5:5\n6:6\n7:7\n8:8\n9:9\n10:10\n11:11\n12:12\n13:13\n14:14\n15:15\n16:16\n17:17\n18:18\n19:19\n20:20\n21:21\n22:22\n23:23\n24:24\n25:25\n26:26\n27:27\n28:28\n29:29\n30:30\r\n", "Адрес"=14, "Описание"="Время, по истечению которого привод переходит в состояние останова, если не достигнута заданная скорость", "Мин"=0, "Макс"=30, "Сервис"=FALSE, "Только чтение"=FALSE, "Разработка"=FALSE, "К-во бит"=16, "Шаг"=1, "Обработка"=TRUE, "Макрос"="macros vp6\n  ON_READ\n  READ vp6\n  if vp4=0\n  READ vp4\n  fi\n  vp6=vp6/vp4\n  RETURN vp6\n  ON_WRITE\n  if vp4=0\n  READ vp4\n  fi\n  vp6=val*vp4\n  WRITE vp6\n  ON_ERROR\n  vp6=100000000000000\n  RETURN vp6\nend"}, {"Имя"="cp5", "Группа"="cp", "Наименование"="Состояние контура тока", "Ед. изм"=0, "Список"="0:Разомкнут\n2:Замкнут\n4:Прямое управление токами в обмотках\n5:Адаптивное упрваление\n6:Прямое раздельное управление токами в обмотках\n\r\n", "Адрес"=16, "Описание"="Обеспечивает замкнутое или разомкнутое регулирование контура тока. В стандартном режиме использования контур должен быть замкнут.", "Мин"=0, "Макс"=6, "Сервис"=FALSE, "Только чтение"=FALSE, "Разработка"=FALSE, "К-во бит"=16, "Шаг"=0, "Обработка"=FALSE, "Макрос"=""}, {"Имя"="vp7", "Группа"="vp", "Наименование"="Состояние контура скорости", "Ед. изм"=0, "Список"="0:Разомкнут\n2:Замкнут\n\r\n", "Адрес"=17, "Описание"="Обеспечивает замкнутое или разомкнутое регулирование контура скорости. Контур должен быть замкнут в режиме управления скоростью привода и в режиме управления позицией.", "Мин"=0, "Макс"=2, "Сервис"=FALSE, "Только чтение"=FALSE, "Разработка"=FALSE, "К-во бит"=16, "Шаг"=0, "Обработка"=FALSE, "Макрос"=""}, {"Имя"="pp5", "Группа"="pp", "Наименование"="Состояние контура положения", "Ед. изм"=0, "Список"="0:Разомкнут\n2:Замкнут\n\r\n", "Адрес"=18, "Описание"="Обеспечивает замкнутое или разомкнутое регулирование контура позиции", "Мин"=0, "Макс"=2, "Сервис"=FALSE, "Только чтение"=FALSE, "Разработка"=FALSE, "К-во бит"=16, "Шаг"=0, "Обработка"=FALSE, "Макрос"=""}, {"Имя"="vp8", "Группа"="vp", "Наименование"="Максимальная скорость вращения", "Ед. изм"=4, "Список"="", "Адрес"=20, "Описание"="Ограничение максимальной скорости вращения привода.", "Мин"=0, "Макс"=8000, "Сервис"=TRUE, "Только чтение"=FALSE, "Разработка"=FALSE, "К-во бит"=32, "Шаг"=12, "Обработка"=FALSE, "Макрос"=""}, {"Имя"="vp9", "Группа"="vp", "Наименование"="Динамический режим", "Ед. изм"=0, "Список"="0:Режим плавного разгона/торможения\n2:Режим с максимальной динамикой\n3:Режим G декодирования\n4:S кривая\n\r\n", "Адрес"=15, "Описание"="Включает или отключает внутренний интерполятор. В режиме управления приводов от внешнего контроллера, например, от ЧПУ, привод должен находиться в режиме с максимальной динамикой. Режим G декодирования позволяет реализовать контурное управление непосредственно группой приводов без использования внешнего контроллера.", "Мин"=0, "Макс"=4, "Сервис"=FALSE, "Только чтение"=FALSE, "Разработка"=FALSE, "К-во бит"=16, "Шаг"=0, "Обработка"=FALSE, "Макрос"=""}, {"Имя"="ss1", "Группа"="ss", "Наименование"="Тестовый параметр", "Ед. изм"=0, "Список"="", "Адрес"=19, "Описание"="", "Мин"=-65535, "Макс"=65535, "Сервис"=FALSE, "Только чтение"=FALSE, "Разработка"=TRUE, "К-во бит"=16, "Шаг"=0, "Обработка"=FALSE, "Макрос"=""}, {"Имя"="ct1", "Группа"="ct", "Наименование"="Задание тока", "Ед. изм"=5, "Список"="", "Адрес"=512, "Описание"="Сигнал управления при разомкнутом контуре скорости и положения", "Мин"=-3500, "Макс"=3500, "Сервис"=FALSE, "Только чтение"=FALSE, "Разработка"=FALSE, "К-во бит"=16, "Шаг"=0, "Обработка"=TRUE, "Макрос"="macros ct1\n  ON_READ\n  READ ct1\n  ct1=ct1*5/2500\n  RETURN ct1\n  ON_WRITE\n  ct1=val*2500/5\n  WRITE ct1\nend"}, {"Имя"="ct2", "Группа"="ct", "Наименование"="Задание скорости", "Ед. изм"=4, "Список"="", "Адрес"=514, "Описание"="Сигнал управления при разомкнутом контуре положения", "Мин"=-12000, "Макс"=12000, "Сервис"=TRUE, "Только чтение"=FALSE, "Разработка"=FALSE, "К-во бит"=32, "Шаг"=12, "Обработка"=FALSE, "Макрос"=""}, {"Имя"="ct3", "Группа"="ct", "Наименование"="Задание положения", "Ед. изм"=6, "Список"="", "Адрес"=516, "Описание"="Сигнал управления при замкнутом контуре положения", "Мин"=-2147483647, "Макс"=2147483647, "Сервис"=FALSE, "Только чтение"=FALSE, "Разработка"=FALSE, "К-во бит"=32, "Шаг"=0, "Обработка"=FALSE, "Макрос"=""}, {"Имя"="dd1", "Группа"="dd", "Наименование"="Ток в обмотке 1", "Ед. изм"=5, "Список"="", "Адрес"=1024, "Описание"="Показывает ток, протекающий в обмотке двигателя", "Мин"=-5, "Макс"=5, "Сервис"=FALSE, "Только чтение"=TRUE, "Разработка"=FALSE, "К-во бит"=16, "Шаг"=0, "Обработка"=TRUE, "Макрос"="macros dd1\n  ON_READ\n  READ dd1\n  dd1=dd1*5/2047\n  RETURN dd1\n  ON_WRITE\n  dd1=val*2047/5\n  WRITE dd1\nend"}, {"Имя"="dd6", "Группа"="dd", "Наименование"="Заданный ток в обмотке 1", "Ед. изм"=5, "Список"="", "Адрес"=1034, "Описание"="", "Мин"=-2047, "Макс"=2047, "Сервис"=FALSE, "Только чтение"=FALSE, "Разработка"=FALSE, "К-во бит"=16, "Шаг"=0, "Обработка"=TRUE, "Макрос"="macros dd6\n  ON_READ\n  READ dd6\n  dd6=dd6*5/2047\n  RETURN dd6\n  ON_WRITE\n  dd6=val*2047/5\n  WRITE dd6\nend"}, {"Имя"="dd3", "Группа"="dd", "Наименование"="Ток в обмотке 2", "Ед. изм"=5, "Список"="", "Адрес"=1029, "Описание"="Индицирует ток, протекающий в обмотке двигателя", "Мин"=-5, "Макс"=5, "Сервис"=FALSE, "Только чтение"=TRUE, "Разработка"=FALSE, "К-во бит"=16, "Шаг"=0, "Обработка"=TRUE, "Макрос"="macros dd3\n  ON_READ\n  READ dd3\n  dd3=dd3*5/2047\n  RETURN dd3\n  ON_WRITE\n  dd3=val*2047/5\n  WRITE dd3\nend"}, {"Имя"="dd9", "Группа"="dd", "Наименование"="Заданный ток в обмотке 2", "Ед. изм"=5, "Список"="", "Адрес"=1037, "Описание"="", "Мин"=-2047, "Макс"=2047, "Сервис"=FALSE, "Только чтение"=FALSE, "Разработка"=FALSE, "К-во бит"=16, "Шаг"=0, "Обработка"=TRUE, "Макрос"="macros dd9\n  ON_READ\n  READ dd9\n  dd9=dd9*5/2047\n  RETURN dd9\n  ON_WRITE\n  dd9=val*2047/5\n  WRITE dd9\nend"}, {"Имя"="dd2", "Группа"="dd", "Наименование"="Заданный ток в роторной системе координат", "Ед. изм"=5, "Список"="", "Адрес"=1026, "Описание"="Индицирует ток, который задан контуром скорости", "Мин"=-5, "Макс"=5, "Сервис"=FALSE, "Только чтение"=TRUE, "Разработка"=FALSE, "К-во бит"=16, "Шаг"=0, "Обработка"=TRUE, "Макрос"="macros dd2\n  ON_READ\n  READ dd2\n  dd2=dd2*5/2047\n  RETURN dd2\n  ON_WRITE\n  dd2=val*2047/5\n  WRITE dd2\nend"}, {"Имя"="dd4", "Группа"="dd", "Наименование"="Текущая скорость вращения", "Ед. изм"=4, "Список"="", "Адрес"=1032, "Описание"="", "Мин"=-5000, "Макс"=5000, "Сервис"=FALSE, "Только чтение"=TRUE, "Разработка"=FALSE, "К-во бит"=8, "Шаг"=12, "Обработка"=FALSE, "Макрос"=""}, {"Имя"="dd5", "Группа"="dd", "Наименование"="Заданная скорость вращения", "Ед. изм"=4, "Список"="", "Адрес"=1033, "Описание"="", "Мин"=-5000, "Макс"=5000, "Сервис"=FALSE, "Только чтение"=TRUE, "Разработка"=FALSE, "К-во бит"=16, "Шаг"=12, "Обработка"=FALSE, "Макрос"=""}, {"Имя"="dd21", "Группа"="dd", "Наименование"="Ошибка контура скорости", "Ед. изм"=4, "Список"="", "Адрес"=1049, "Описание"="", "Мин"=-65535, "Макс"=65535, "Сервис"=FALSE, "Только чтение"=TRUE, "Разработка"=FALSE, "К-во бит"=16, "Шаг"=1, "Обработка"=FALSE, "Макрос"=""}, {"Имя"="dd7", "Группа"="dd", "Наименование"="Заданная позиция", "Ед. изм"=6, "Список"="", "Адрес"=1035, "Описание"="", "Мин"=-2147483647, "Макс"=2147483647, "Сервис"=FALSE, "Только чтение"=TRUE, "Разработка"=FALSE, "К-во бит"=32, "Шаг"=0, "Обработка"=FALSE, "Макрос"=""}, {"Имя"="dd8", "Группа"="dd", "Наименование"="Текущая позиция", "Ед. изм"=6, "Список"="", "Адрес"=1036, "Описание"="", "Мин"=-2147483647, "Макс"=2147483647, "Сервис"=FALSE, "Только чтение"=TRUE, "Разработка"=FALSE, "К-во бит"=32, "Шаг"=0, "Обработка"=FALSE, "Макрос"=""}, {"Имя"="dd20", "Группа"="dd", "Наименование"="Ошибка контура позиции", "Ед. изм"=6, "Список"="", "Адрес"=1048, "Описание"="", "Мин"=-2147483647, "Макс"=2147483647, "Сервис"=TRUE, "Только чтение"=TRUE, "Разработка"=FALSE, "К-во бит"=32, "Шаг"=10, "Обработка"=FALSE, "Макрос"=""}, {"Имя"="dd10", "Группа"="dd", "Наименование"="Температура внутри корпуса", "Ед. изм"=7, "Список"="", "Адрес"=1038, "Описание"="", "Мин"=-40, "Макс"=120, "Сервис"=FALSE, "Только чтение"=TRUE, "Разработка"=FALSE, "К-во бит"=16, "Шаг"=0, "Обработка"=TRUE, "Макрос"="macros dd10\n  ON_READ\n  READ dd10\n  dd10=dd10/128\n  RETURN dd10\n  ON_WRITE\n  dd10=val\n  WRITE dd10\nend"}, {"Имя"="dd19", "Группа"="dd", "Наименование"="Текущее цифровое напряжение", "Ед. изм"=8, "Список"="", "Адрес"=1047, "Описание"="", "Мин"=0, "Макс"=23, "Сервис"=FALSE, "Только чтение"=TRUE, "Разработка"=FALSE, "К-во бит"=16, "Шаг"=0, "Обработка"=TRUE, "Макрос"="macros dd19\n  ON_READ\n  READ dd19\n  dd19=dd19/178\n  RETURN dd19\n  ON_WRITE\n  dd19=val\n  WRITE dd19\nend"}, {"Имя"="dd12", "Группа"="dd", "Наименование"="Текущее напряжение питания", "Ед. изм"=8, "Список"="", "Адрес"=1040, "Описание"="", "Мин"=0, "Макс"=120, "Сервис"=FALSE, "Только чтение"=TRUE, "Разработка"=FALSE, "К-во бит"=16, "Шаг"=0, "Обработка"=TRUE, "Макрос"="macros dd12\n  ON_READ\n  READ dd12\n  dd12=dd12/21\n  RETURN dd12\n  ON_WRITE\n  dd12=val\n  WRITE dd12\nend"}, {"Имя"="dd11", "Группа"="dd", "Наименование"="Статус контроллера", "Ед. изм"=0, "Список"="0:Исправен\n1:Останов по команде\n2:Останов - высокое противодействующее усилие\n3:Останов - короткое замыкание\n4:Выход из температурного диапазона\n5:Повышенное силовое напряжение\n6:Низкое силовое напряжение\n7:Повышенное цифровое напряжение\n8:Низкое цифровое напряжение\n9:Cиловое напряжение превышает напряжение, установл. пользователем\n10:Останов - превышение допустимой перегрузки\n11:Останов - сработала защита IGBT модуля\n12:Останов - Ошибка поиска фазы по UVW трекам\n13:Останов - ошибка в настройках энкодера\n14: Останов - сбой в работе энкодера\n15: Останов - Ошибка фазировки двигателя\n\r\n", "Адрес"=1039, "Описание"="Привод в состоянии отработать задание только, если его статус \"Исправен\".", "Мин"=0, "Макс"=15, "Сервис"=FALSE, "Только чтение"=FALSE, "Разработка"=FALSE, "К-во бит"=16, "Шаг"=0, "Обработка"=FALSE, "Макрос"=""}, {"Имя"="st1", "Группа"="st", "Наименование"="Разрешение", "Ед. изм"=6, "Список"="", "Адрес"=21, "Описание"="Разрешение датчика положения/скорости", "Мин"=0, "Макс"=2147483647, "Сервис"=FALSE, "Только чтение"=FALSE, "Разработка"=FALSE, "К-во бит"=32, "Шаг"=0, "Обработка"=FALSE, "Макрос"=""}, {"Имя"="tp1", "Группа"="tp", "Наименование"="Режим осциллографа", "Ед. изм"=0, "Список"="0:Непрерывный режим\n1:Ступенька\n2:Синус\n3:Приращение скорости\n4:Синусоидальное изменение скорости\n5:Треугольное изменение позиции\n6:Измерение без задания\n7:Измерение без задания до принудительного останова\n8:Приращение момента\n\r\n", "Адрес"=1280, "Описание"="Режим сканирования динамических параметров (отображение выбранных параметров в процессе работы привода).", "Мин"=0, "Макс"=8, "Сервис"=FALSE, "Только чтение"=FALSE, "Разработка"=FALSE, "К-во бит"=16, "Шаг"=0, "Обработка"=FALSE, "Макрос"=""}, {"Имя"="tp3", "Группа"="tp", "Наименование"="Амплитуда задания положения", "Ед. изм"=0, "Список"="", "Адрес"=1284, "Описание"="Определяет величину приращения позиции в режиме осциллографа 1.", "Мин"=-2147483647, "Макс"=2147483647, "Сервис"=FALSE, "Только чтение"=FALSE, "Разработка"=FALSE, "К-во бит"=32, "Шаг"=0, "Обработка"=FALSE, "Макрос"=""}, {"Имя"="ip0", "Группа"="ip", "Наименование"="Источник опорного сигнала", "Ед. изм"=0, "Список"="0:Интерфейс USB\n2:Интерфейс StepDir\n4:Аналоговый интерфейс\n5:Интерфейс CAN\n6:Квадратурный интерфейс\r\n", "Адрес"=23, "Описание"="Определяет интерфейс, по которому осуществляется ввод задания для привода.", "Мин"=0, "Макс"=6, "Сервис"=FALSE, "Только чтение"=FALSE, "Разработка"=FALSE, "К-во бит"=16, "Шаг"=0, "Обработка"=FALSE, "Макрос"=""}, {"Имя"="st2", "Группа"="st", "Наименование"="Версия ПО драйвера", "Ед. изм"=0, "Список"="", "Адрес"=22, "Описание"="Текущая версия программного обеспечения привода.", "Мин"=0, "Макс"=2147483647, "Сервис"=TRUE, "Только чтение"=FALSE, "Разработка"=FALSE, "К-во бит"=32, "Шаг"=12, "Обработка"=FALSE, "Макрос"=""}, {"Имя"="ip1", "Группа"="ip", "Наименование"="Коэффициент веса одной дискреты", "Ед. изм"=0, "Список"="", "Адрес"=24, "Описание"="Определяет количество импульсов датчика, на которые необходимо повернуть вал двигателя, при получении одной дискреты по интерфейсу Step/Dir, т.е. масштаб одного импульса", "Мин"=-4000, "Макс"=4000, "Сервис"=TRUE, "Только чтение"=FALSE, "Разработка"=FALSE, "К-во бит"=32, "Шаг"=10, "Обработка"=FALSE, "Макрос"=""}, {"Имя"="tp2", "Группа"="tp", "Наименование"="Период опроса параметров", "Ед. изм"=9, "Список"="", "Адрес"=1282, "Описание"="Определяет интервал времени между запоминанием данных в массив в режимах 1-7.", "Мин"=25, "Макс"=25000, "Сервис"=FALSE, "Только чтение"=FALSE, "Разработка"=FALSE, "К-во бит"=16, "Шаг"=25, "Обработка"=FALSE, "Макрос"=""}, {"Имя"="tp5", "Группа"="tp", "Наименование"="Период задающего воздействия", "Ед. изм"=9, "Список"="", "Адрес"=1285, "Описание"="Данный параметр определяет задержку введения задающего воздействия от начала сбора информации в режиме осциллографа 1 и 3.", "Мин"=25, "Макс"=800000, "Сервис"=FALSE, "Только чтение"=FALSE, "Разработка"=FALSE, "К-во бит"=16, "Шаг"=25, "Обработка"=TRUE, "Макрос"="macros tp5\n  ON_READ\n  READ tp5\n  tp5=tp5*25\n  RETURN tp5\n  ON_WRITE\n  tp5=val/25\n  WRITE tp5\n  ON_ERROR\n  err=100000000000\n  RETURN err\nend"}, {"Имя"="tp6", "Группа"="tp", "Наименование"="Амплитуда задания скорости", "Ед. изм"=4, "Список"="", "Адрес"=1286, "Описание"="Определяет величину приращения скорости в режиме осциллографа 3.", "Мин"=-14000, "Макс"=14000, "Сервис"=FALSE, "Только чтение"=FALSE, "Разработка"=FALSE, "К-во бит"=16, "Шаг"=0, "Обработка"=FALSE, "Макрос"=""}, {"Имя"="ip2", "Группа"="ip", "Наименование"="Текущий банк программы интерпретатора", "Ед. изм"=10, "Список"="0:0\n1:1\n2:2\n3:3\n4:4\n5:5\n6:6\n7:7\n255:Программа не выбрана\n\r\n", "Адрес"=26, "Описание"="Банк, из которой загружена программа на выполнение.", "Мин"=0, "Макс"=255, "Сервис"=FALSE, "Только чтение"=FALSE, "Разработка"=FALSE, "К-во бит"=16, "Шаг"=1, "Обработка"=FALSE, "Макрос"=""}, {"Имя"="ip3", "Группа"="ip", "Наименование"="Текущий банк чт/записи программ интерпретатора", "Ед. изм"=10, "Список"="0:0\n1:1\n2:2\n3:3\n4:4\n5:5\n6:6\n7:7\n255:Программа не выбрана\n\r\n", "Адрес"=27, "Описание"="", "Мин"=0, "Макс"=255, "Сервис"=FALSE, "Только чтение"=TRUE, "Разработка"=TRUE, "К-во бит"=16, "Шаг"=1, "Обработка"=FALSE, "Макрос"=""}, {"Имя"="ip4", "Группа"="ip", "Наименование"="Режим работы интерпретатора", "Ед. изм"=0, "Список"="0:Режим выполнения программы\n1:Режим отладки\n\r\n", "Адрес"=28, "Описание"="Режим работы интерпретатора", "Мин"=0, "Макс"=1, "Сервис"=FALSE, "Только чтение"=FALSE, "Разработка"=FALSE, "К-во бит"=16, "Шаг"=1, "Обработка"=FALSE, "Макрос"=""}, {"Имя"="st3", "Группа"="st", "Наименование"="Уникальный идентификатор устройства", "Ед. изм"=0, "Список"="", "Адрес"=30, "Описание"="", "Мин"=0, "Макс"=2147483647, "Сервис"=FALSE, "Только чтение"=FALSE, "Разработка"=FALSE, "К-во бит"=32, "Шаг"=0, "Обработка"=FALSE, "Макрос"=""}, {"Имя"="ip5", "Группа"="ip", "Наименование"="Порт ввода вывода", "Ед. изм"=0, "Список"="", "Адрес"=29, "Описание"="Старший байт содержит содержимое порта вывода, младший - состояние линий ввода.", "Мин"=0, "Макс"=65535, "Сервис"=FALSE, "Только чтение"=FALSE, "Разработка"=FALSE, "К-во бит"=16, "Шаг"=0, "Обработка"=FALSE, "Макрос"=""}, {"Имя"="ss2", "Группа"="ss", "Наименование"="Количество КЗ", "Ед. изм"=0, "Список"="", "Адрес"=31, "Описание"="Количество зафиксированных коротких замыканий", "Мин"=0, "Макс"=65535, "Сервис"=FALSE, "Только чтение"=FALSE, "Разработка"=FALSE, "К-во бит"=16, "Шаг"=0, "Обработка"=FALSE, "Макрос"=""}, {"Имя"="ss3", "Группа"="ss", "Наименование"="Количество превышений температуры", "Ед. изм"=0, "Список"="", "Адрес"=32, "Описание"="Количество зафиксированных превышений температуры", "Мин"=0, "Макс"=65535, "Сервис"=FALSE, "Только чтение"=FALSE, "Разработка"=FALSE, "К-во бит"=16, "Шаг"=0, "Обработка"=FALSE, "Макрос"=""}, {"Имя"="ss4", "Группа"="ss", "Наименование"="Количество перенапряжений", "Ед. изм"=0, "Список"="", "Адрес"=33, "Описание"="Количество зафиксированных перенапряжений", "Мин"=0, "Макс"=65535, "Сервис"=FALSE, "Только чтение"=FALSE, "Разработка"=FALSE, "К-во бит"=16, "Шаг"=0, "Обработка"=FALSE, "Макрос"=""}, {"Имя"="ss5", "Группа"="ss", "Наименование"="Количество недонапряжений", "Ед. изм"=0, "Список"="", "Адрес"=34, "Описание"="Количество зафиксированных случаев пониженного напряжений", "Мин"=0, "Макс"=65535, "Сервис"=FALSE, "Только чтение"=FALSE, "Разработка"=FALSE, "К-во бит"=16, "Шаг"=0, "Обработка"=FALSE, "Макрос"=""}, {"Имя"="ss6", "Группа"="ss", "Наименование"="Количество перегрузок", "Ед. изм"=0, "Список"="", "Адрес"=35, "Описание"="", "Мин"=0, "Макс"=65535, "Сервис"=FALSE, "Только чтение"=FALSE, "Разработка"=FALSE, "К-во бит"=16, "Шаг"=0, "Обработка"=FALSE, "Макрос"=""}, {"Имя"="ss7", "Группа"="ss", "Наименование"="Количество перепрогарммирований", "Ед. изм"=0, "Список"="", "Адрес"=36, "Описание"="", "Мин"=0, "Макс"=65535, "Сервис"=FALSE, "Только чтение"=FALSE, "Разработка"=FALSE, "К-во бит"=16, "Шаг"=0, "Обработка"=FALSE, "Макрос"=""}, {"Имя"="ss8", "Группа"="ss", "Наименование"="Сообщение 0", "Ед. изм"=0, "Список"="1:Короткое замыкание\n2:Перегрев\n3:Повышенное напряжение\n4:Пониженное напряжение\n5:Перегрузка по току\n6:Произведена перезапись контроллера\n\r\n", "Адрес"=37, "Описание"="Журнал последних 8 сообщений", "Мин"=0, "Макс"=65535, "Сервис"=FALSE, "Только чтение"=FALSE, "Разработка"=FALSE, "К-во бит"=16, "Шаг"=0, "Обработка"=FALSE, "Макрос"=""}, {"Имя"="ss9", "Группа"="ss", "Наименование"="Сообщение 1", "Ед. изм"=0, "Список"="1:Короткое замыкание\n2:Перегрев\n3:Повышенное напряжение\n4:Пониженное напряжение\n5:Перегрузка по току\n6:Произведена перезапись контроллера\n\r\n", "Адрес"=38, "Описание"="Журнал последних 8 сообщений", "Мин"=0, "Макс"=65535, "Сервис"=FALSE, "Только чтение"=FALSE, "Разработка"=FALSE, "К-во бит"=16, "Шаг"=0, "Обработка"=FALSE, "Макрос"=""}, {"Имя"="ss10", "Группа"="ss", "Наименование"="Сообщение 2", "Ед. изм"=0, "Список"="1:Короткое замыкание\n2:Перегрев\n3:Повышенное напряжение\n4:Пониженное напряжение\n5:Перегрузка по току\n6:Произведена перезапись контроллера\n\r\n", "Адрес"=39, "Описание"="Журнал последних 8 сообщений", "Мин"=0, "Макс"=65535, "Сервис"=FALSE, "Только чтение"=FALSE, "Разработка"=FALSE, "К-во бит"=16, "Шаг"=0, "Обработка"=FALSE, "Макрос"=""}, {"Имя"="ss11", "Группа"="ss", "Наименование"="Сообщение 3", "Ед. изм"=0, "Список"="1:Короткое замыкание\n2:Перегрев\n3:Повышенное напряжение\n4:Пониженное напряжение\n5:Перегрузка по току\n6:Произведена перезапись контроллера\n\r\n", "Адрес"=40, "Описание"="Журнал последних 8 сообщений", "Мин"=0, "Макс"=65535, "Сервис"=FALSE, "Только чтение"=FALSE, "Разработка"=FALSE, "К-во бит"=16, "Шаг"=0, "Обработка"=FALSE, "Макрос"=""}, {"Имя"="ss12", "Группа"="ss", "Наименование"="Сообщение 4", "Ед. изм"=0, "Список"="1:Короткое замыкание\n2:Перегрев\n3:Повышенное напряжение\n4:Пониженное напряжение\n5:Перегрузка по току\n6:Произведена перезапись контроллера\n\r\n", "Адрес"=41, "Описание"="Журнал последних 8 сообщений", "Мин"=0, "Макс"=65535, "Сервис"=FALSE, "Только чтение"=FALSE, "Разработка"=FALSE, "К-во бит"=16, "Шаг"=0, "Обработка"=FALSE, "Макрос"=""}, {"Имя"="ss13", "Группа"="ss", "Наименование"="Сообщение 5", "Ед. изм"=0, "Список"="1:Короткое замыкание\n2:Перегрев\n3:Повышенное напряжение\n4:Пониженное напряжение\n5:Перегрузка по току\n6:Произведена перезапись контроллера\n\r\n", "Адрес"=42, "Описание"="Журнал последних 8 сообщений", "Мин"=0, "Макс"=65535, "Сервис"=FALSE, "Только чтение"=FALSE, "Разработка"=FALSE, "К-во бит"=16, "Шаг"=0, "Обработка"=FALSE, "Макрос"=""}, {"Имя"="ss14", "Группа"="ss", "Наименование"="Сообщение 6", "Ед. изм"=0, "Список"="1:Короткое замыкание\n2:Перегрев\n3:Повышенное напряжение\n4:Пониженное напряжение\n5:Перегрузка по току\n6:Произведена перезапись контроллера\n\r\n", "Адрес"=43, "Описание"="Журнал последних 8 сообщений", "Мин"=0, "Макс"=65535, "Сервис"=FALSE, "Только чтение"=FALSE, "Разработка"=FALSE, "К-во бит"=16, "Шаг"=0, "Обработка"=FALSE, "Макрос"=""}, {"Имя"="ss15", "Группа"="ss", "Наименование"="Сообщение 7", "Ед. изм"=0, "Список"="1:Короткое замыкание\n2:Перегрев\n3:Повышенное напряжение\n4:Пониженное напряжение\n5:Перегрузка по току\n6:Произведена перезапись контроллера\n\r\n", "Адрес"=44, "Описание"="Журнал последних 8 сообщений", "Мин"=0, "Макс"=65535, "Сервис"=FALSE, "Только чтение"=FALSE, "Разработка"=FALSE, "К-во бит"=16, "Шаг"=0, "Обработка"=FALSE, "Макрос"=""}, {"Имя"="ip6", "Группа"="ip", "Наименование"="Смещение диапазона сигнала управления", "Ед. изм"=0, "Список"="", "Адрес"=48, "Описание"="Используется для корректировки диапазона регулирования входного сигнала (аналогового или Step\\Dir). Значение 2048 соответствует нулевой скорости при подаче на вход нулевого напряжения.", "Мин"=0, "Макс"=4096, "Сервис"=FALSE, "Только чтение"=FALSE, "Разработка"=FALSE, "К-во бит"=16, "Шаг"=0, "Обработка"=FALSE, "Макрос"=""}, {"Имя"="dd13", "Группа"="dd", "Наименование"="Тестовый параметр 1", "Ед. изм"=0, "Список"="", "Адрес"=1041, "Описание"="Пока используется для индикации перехода на меандр вместо синуса. Параметр для разработчика", "Мин"=-65535, "Макс"=65535, "Сервис"=FALSE, "Только чтение"=TRUE, "Разработка"=TRUE, "К-во бит"=16, "Шаг"=0, "Обработка"=FALSE, "Макрос"=""}, {"Имя"="dd14", "Группа"="dd", "Наименование"="Тестовый параметр 2", "Ед. изм"=0, "Список"="", "Адрес"=1042, "Описание"="Пока используется для индикации сдвига фазы", "Мин"=-65535, "Макс"=65535, "Сервис"=FALSE, "Только чтение"=TRUE, "Разработка"=TRUE, "К-во бит"=16, "Шаг"=0, "Обработка"=FALSE, "Макрос"=""}, {"Имя"="vp10", "Группа"="vp", "Наименование"="Начало резонансного диапазона 1", "Ед. изм"=4, "Список"="", "Адрес"=49, "Описание"="Если начало и конец диапазона равны, то диапазон не выбран.", "Мин"=0, "Макс"=8000, "Сервис"=FALSE, "Только чтение"=FALSE, "Разработка"=FALSE, "К-во бит"=16, "Шаг"=0, "Обработка"=TRUE, "Макрос"="macros vp10\n  ON_READ\n  READ vp10\n  if st1=0\n  READ st1\n  fi\n  if vp4=0\n  READ vp4\n  fi\n  if vp3=0\n  READ vp3\n  fi\n  vp10=round(60*vp10*vp4/(st1*vp3))\n  RETURN vp10\n  ON_WRITE\n  if st1=0\n  READ st1\n  fi\n  if vp4=0\n  READ vp4\n  fi\n  if vp3=0\n  READ vp3\n  fi\n  vp10=val*st1*vp3/(60*vp4)\n  WRITE vp10\n  ON_ERROR\n  vp10=100000000000000\n  RETURN vp10\nend"}, {"Имя"="vp11", "Группа"="vp", "Наименование"="Конец резонансного диапазона 1", "Ед. изм"=4, "Список"="", "Адрес"=50, "Описание"="Если начало и конец диапазона равны, то диапазон не выбран.", "Мин"=0, "Макс"=8000, "Сервис"=FALSE, "Только чтение"=FALSE, "Разработка"=FALSE, "К-во бит"=16, "Шаг"=0, "Обработка"=TRUE, "Макрос"="macros vp11\n  ON_READ\n  READ vp11\n  if st1=0\n  READ st1\n  fi\n  if vp4=0\n  READ vp4\n  fi\n  if vp3=0\n  READ vp3\n  fi\n  vp11=round(60*vp11*vp4/(st1*vp3))\n  RETURN vp11\n  ON_WRITE\n  if st1=0\n  READ st1\n  fi\n  if vp4=0\n  READ vp4\n  fi\n  if vp3=0\n  READ vp3\n  fi\n  vp11=val*st1*vp3/(60*vp4)\n  WRITE vp11\n  ON_ERROR\n  vp11=100000000000000\n  RETURN vp11\nend"}, {"Имя"="vp12", "Группа"="vp", "Наименование"="Начало резонансного диапазона 2", "Ед. изм"=4, "Список"="", "Адрес"=51, "Описание"="Если начало и конец диапазона равны, то диапазон не выбран.", "Мин"=0, "Макс"=8000, "Сервис"=FALSE, "Только чтение"=FALSE, "Разработка"=FALSE, "К-во бит"=16, "Шаг"=0, "Обработка"=TRUE, "Макрос"="macros vp12\n  ON_READ\n  READ vp12\n  if st1=0\n  READ st1\n  fi\n  if vp4=0\n  READ vp4\n  fi\n  if vp3=0\n  READ vp3\n  fi\n  vp12=round(60*vp12*vp4/(st1*vp3))\n  RETURN vp12\n  ON_WRITE\n  if st1=0\n  READ st1\n  fi\n  if vp4=0\n  READ vp4\n  fi\n  if vp3=0\n  READ vp3\n  fi\n  vp12=val*st1*vp3/(60*vp4)\n  WRITE vp12\n  ON_ERROR\n  vp12=100000000000000\n  RETURN vp12\nend"}, {"Имя"="vp13", "Группа"="vp", "Наименование"="Конец резонансного диапазона 2", "Ед. изм"=4, "Список"="", "Адрес"=52, "Описание"="Если начало и конец диапазона равны, то диапазон не выбран.", "Мин"=0, "Макс"=8000, "Сервис"=FALSE, "Только чтение"=FALSE, "Разработка"=FALSE, "К-во бит"=16, "Шаг"=0, "Обработка"=TRUE, "Макрос"="macros vp13\n  ON_READ\n  READ vp13\n  if st1=0\n  READ st1\n  fi\n  if vp4=0\n  READ vp4\n  fi\n  if vp3=0\n  READ vp3\n  fi\n  vp13=round(60*vp13*vp4/(st1*vp3))\n  RETURN vp13\n  ON_WRITE\n  if st1=0\n  READ st1\n  fi\n  if vp4=0\n  READ vp4\n  fi\n  if vp3=0\n  READ vp3\n  fi\n  vp13=val*st1*vp3/(60*vp4)\n  WRITE vp13\n  ON_ERROR\n  vp13=100000000000000\n  RETURN vp13\nend"}, {"Имя"="ip7", "Группа"="ip", "Наименование"="CAN адрес устройства", "Ед. изм"=0, "Список"="", "Адрес"=53, "Описание"="Адрес данного устройства в сети CAN", "Мин"=0, "Макс"=127, "Сервис"=FALSE, "Только чтение"=FALSE, "Разработка"=FALSE, "К-во бит"=16, "Шаг"=0, "Обработка"=FALSE, "Макрос"=""}, {"Имя"="ip8", "Группа"="ip", "Наименование"="CAN адрес удаленного узла", "Ед. изм"=0, "Список"="", "Адрес"=54, "Описание"="Адрес удаленного устройства в сети CAN, которое выступает в качестве мастера для данного устройства", "Мин"=0, "Макс"=127, "Сервис"=FALSE, "Только чтение"=FALSE, "Разработка"=FALSE, "К-во бит"=16, "Шаг"=0, "Обработка"=FALSE, "Макрос"=""}, {"Имя"="ip9", "Группа"="ip", "Наименование"="Режим синхронизации по CAN", "Ед. изм"=0, "Список"="0:Режим не выбран\n1:Режим мастер\n2:Режим слейв\n3:Режим контурного управления\n4:Синхронизация по команде SYNC\n\r\n", "Адрес"=55, "Описание"="В режиме мастер привод передает текущую позицию в CAN на адрес удаленного узла.", "Мин"=0, "Макс"=4, "Сервис"=FALSE, "Только чтение"=FALSE, "Разработка"=FALSE, "К-во бит"=16, "Шаг"=0, "Обработка"=FALSE, "Макрос"=""}, {"Имя"="ip10", "Группа"="ip", "Наименование"="Статус шины CAN", "Ед. изм"=0, "Список"="0:Норма\n1:Неисправности на линии\n2:Ошибка передачи синхронизации слейву\n3:Ошибка - подтверждение не получено.\r\n", "Адрес"=56, "Описание"="Статус 2 - устанавливается, если мастер не может передать сообщение слейву в течение ip7", "Мин"=0, "Макс"=3, "Сервис"=FALSE, "Только чтение"=TRUE, "Разработка"=FALSE, "К-во бит"=16, "Шаг"=0, "Обработка"=FALSE, "Макрос"=""}, {"Имя"="vp14", "Группа"="vp", "Наименование"="Номинальная скорость", "Ед. изм"=4, "Список"="", "Адрес"=57, "Описание"="Скорость, начиная с которой выполняется режим ослабления поля.", "Мин"=0, "Макс"=5000, "Сервис"=FALSE, "Только чтение"=FALSE, "Разработка"=FALSE, "К-во бит"=16, "Шаг"=0, "Обработка"=TRUE, "Макрос"="macros vp14\n  ON_READ\n  READ vp14\n  if st1=0\n  READ st1\n  fi\n  if vp4=0\n  READ vp4\n  fi\n  x=round(60*vp14*1000/4000)\n  RETURN x\n  ON_WRITE\n  if st1=0\n  READ st1\n  fi\n  if vp4=0\n  READ vp4\n  fi\n  vp14=val*4000/(60*1000)\n  WRITE vp14\n  ON_STREAM_REQ\n  READ st1\n  READ vp4\n  ON_ERROR\n  dd4=100000000000000\n  RETURN vp14\nend"}, {"Имя"="vp15", "Группа"="vp", "Наименование"="Авто расчет номинальной скорости", "Ед. изм"=0, "Список"="1:Да\n0:Нет\n\r\n", "Адрес"=64, "Описание"="Автоматический расчет номинальной скорости выполняется на основе текущего напряжения питания при включении привода.", "Мин"=0, "Макс"=1, "Сервис"=FALSE, "Только чтение"=FALSE, "Разработка"=FALSE, "К-во бит"=16, "Шаг"=0, "Обработка"=FALSE, "Макрос"=""}, {"Имя"="si1", "Группа"="ss", "Наименование"="Смещение датчика тока 1", "Ед. изм"=0, "Список"="", "Адрес"=1536, "Описание"="Формула расчета I=cur1-511-si1", "Мин"=0, "Макс"=4096, "Сервис"=FALSE, "Только чтение"=FALSE, "Разработка"=TRUE, "К-во бит"=16, "Шаг"=0, "Обработка"=FALSE, "Макрос"=""}, {"Имя"="si2", "Группа"="ss", "Наименование"="Смещение датчика тока 2", "Ед. изм"=0, "Список"="", "Адрес"=1537, "Описание"="Формула расчета I=cur2-511-si2", "Мин"=0, "Макс"=4096, "Сервис"=FALSE, "Только чтение"=FALSE, "Разработка"=TRUE, "К-во бит"=16, "Шаг"=0, "Обработка"=FALSE, "Макрос"=""}, {"Имя"="pp6", "Группа"="pp", "Наименование"="Ограничение интегральной составляющей контура позиции", "Ед. изм"=0, "Список"="", "Адрес"=65, "Описание"="Определяет максимальное значение, до которого может увеличиваться интегральная составляющая. По достижению этой величины интегральная составляющая удерживается константой.", "Мин"=0, "Макс"=15000, "Сервис"=TRUE, "Только чтение"=FALSE, "Разработка"=FALSE, "К-во бит"=32, "Шаг"=10, "Обработка"=FALSE, "Макрос"=""}, {"Имя"="ip11", "Группа"="ip", "Наименование"="Статус интерпретатора", "Ед. изм"=0, "Список"="0:Норма\n1:Смена банка программ\n2:Неизвестный параметр\n3:Неизвестная команда\n4:Останов\n5:STATUS_UNKNOWN_AL_OP\n6:STATUS_UNKNOWN_CMP_OP\n7:Загрузка программы\n8:STATUS_DEBUG_BREAK\n9:STATUS_DEBUG_WAIT_END_OF_CMD\n10:Неизвестная динамическая функция\n11:Старая версия программы\n12:Слишком много циклов\n77:Неправильное условие\n13:Не удалось найти Z метку\n78:Переполнение стека\n79:Попытка чтения пустого стека\n\r\n", "Адрес"=66, "Описание"="", "Мин"=0, "Макс"=12, "Сервис"=FALSE, "Только чтение"=TRUE, "Разработка"=FALSE, "К-во бит"=16, "Шаг"=1, "Обработка"=FALSE, "Макрос"=""}, {"Имя"="ep1", "Группа"="ep", "Наименование"="Режим торможения", "Ед. изм"=0, "Список"="0:Торможение без контроля напряжения\n2:Торможение с контролем напряжения\n\r\n", "Адрес"=67, "Описание"="При торможении без контроля напряжения привод перейдет в аварийное состояние в момент превышения напряжением допустимого значения, установленным в параметре ep2.", "Мин"=0, "Макс"=2, "Сервис"=FALSE, "Только чтение"=FALSE, "Разработка"=FALSE, "К-во бит"=16, "Шаг"=0, "Обработка"=FALSE, "Макрос"=""}, {"Имя"="ep2", "Группа"="ep", "Наименование"="Максимальное напряжение", "Ед. изм"=8, "Список"="", "Адрес"=68, "Описание"="Максимальное допустимое напряжение, при котором привод должен переходить в состояние отключения.", "Мин"=0, "Макс"=280, "Сервис"=FALSE, "Только чтение"=FALSE, "Разработка"=FALSE, "К-во бит"=16, "Шаг"=0, "Обработка"=TRUE, "Макрос"="macros ep2\n  ON_READ\n  READ ep2\n  ep2=ep2/21\n  RETURN ep2\n  ON_WRITE\n  ep2=val*21\n  WRITE ep2\nend"}, {"Имя"="dd15", "Группа"="dd", "Наименование"="Время выполнения команды интерпретатором", "Ед. изм"=11, "Список"="", "Адрес"=1043, "Описание"="Определяет максимальное время, которое интерпретатор затрачивает на выполнение команды в текущей программе.", "Мин"=0, "Макс"=2147483647, "Сервис"=FALSE, "Только чтение"=TRUE, "Разработка"=FALSE, "К-во бит"=32, "Шаг"=1, "Обработка"=TRUE, "Макрос"="macros dd15\n  ON_READ\n  READ dd15\n  dd15=dd15*25/1000\n  RETURN dd15\n  ON_WRITE\n  dd15=val\n  WRITE dd15\nend"}, {"Имя"="dd16", "Группа"="dd", "Наименование"="Время выполнения программы интерпретатором", "Ед. изм"=11, "Список"="", "Адрес"=1044, "Описание"="Определяет максимальное время, которое интерпретатор затрачивает на выполнение всей программы.", "Мин"=0, "Макс"=2147483647, "Сервис"=FALSE, "Только чтение"=TRUE, "Разработка"=FALSE, "К-во бит"=32, "Шаг"=1, "Обработка"=TRUE, "Макрос"="macros dd16\n  ON_READ\n  READ dd16\n  dd16=dd16*25/1000\n  RETURN dd16\n  ON_WRITE\n  dd16=val\n  WRITE dd16\nend"}, {"Имя"="ip12", "Группа"="ip", "Наименование"="Мертвая зона аналоговых входов", "Ед. изм"=1, "Список"="", "Адрес"=69, "Описание"="Определяет зону нечувствительности аналоговых входов привода. При ручном управлении, например, с помощью джойстика, данный параметр позволяет исключить вращение вала при задании нулевой скорости.", "Мин"=0, "Макс"=250, "Сервис"=FALSE, "Только чтение"=FALSE, "Разработка"=FALSE, "К-во бит"=16, "Шаг"=0, "Обработка"=FALSE, "Макрос"=""}, {"Имя"="dd17", "Группа"="dd", "Наименование"="Аналоговый вход 0", "Ед. изм"=1, "Список"="", "Адрес"=1045, "Описание"="", "Мин"=-65535, "Макс"=65535, "Сервис"=FALSE, "Только чтение"=TRUE, "Разработка"=FALSE, "К-во бит"=16, "Шаг"=0, "Обработка"=FALSE, "Макрос"=""}, {"Имя"="dd18", "Группа"="dd", "Наименование"="Аналоговый вход 1", "Ед. изм"=1, "Список"="", "Адрес"=1046, "Описание"="", "Мин"=-65535, "Макс"=65535, "Сервис"=FALSE, "Только чтение"=TRUE, "Разработка"=FALSE, "К-во бит"=16, "Шаг"=0, "Обработка"=FALSE, "Макрос"=""}, {"Имя"="up0", "Группа"="up", "Наименование"="Переменная общего назначения 0", "Ед. изм"=0, "Список"="", "Адрес"=1792, "Описание"="Может использоваться для общих целей. Например, для запоминания длинны оси, приводимой в движение данным приводом и т.д.", "Мин"=-2147483647, "Макс"=2147483647, "Сервис"=FALSE, "Только чтение"=FALSE, "Разработка"=FALSE, "К-во бит"=32, "Шаг"=0, "Обработка"=FALSE, "Макрос"=""}, {"Имя"="up1", "Группа"="up", "Наименование"="Переменная общего назначения 1", "Ед. изм"=0, "Список"="", "Адрес"=1793, "Описание"="Может использоваться для общих целей. Например, для запоминания длинны оси, приводимой в движение данным приводом и т.д.", "Мин"=-2147483647, "Макс"=2147483647, "Сервис"=FALSE, "Только чтение"=FALSE, "Разработка"=FALSE, "К-во бит"=32, "Шаг"=0, "Обработка"=FALSE, "Макрос"=""}, {"Имя"="up2", "Группа"="up", "Наименование"="Переменная общего назначения 2", "Ед. изм"=0, "Список"="", "Адрес"=1794, "Описание"="Может использоваться для общих целей. Например, для запоминания длинны оси, приводимой в движение данным приводом и т.д.", "Мин"=-2147483647, "Макс"=2147483647, "Сервис"=FALSE, "Только чтение"=FALSE, "Разработка"=FALSE, "К-во бит"=32, "Шаг"=0, "Обработка"=FALSE, "Макрос"=""}, {"Имя"="up3", "Группа"="up", "Наименование"="Переменная общего назначения 3", "Ед. изм"=0, "Список"="", "Адрес"=1795, "Описание"="Может использоваться для общих целей. Например, для запоминания длинны оси, приводимой в движение данным приводом и т.д.", "Мин"=-2147483647, "Макс"=2147483647, "Сервис"=FALSE, "Только чтение"=FALSE, "Разработка"=FALSE, "К-во бит"=32, "Шаг"=0, "Обработка"=FALSE, "Макрос"=""}, {"Имя"="up4", "Группа"="up", "Наименование"="Переменная общего назначения 4", "Ед. изм"=0, "Список"="", "Адрес"=1796, "Описание"="Может использоваться для общих целей. Например, для запоминания длинны оси, приводимой в движение данным приводом и т.д.", "Мин"=-2147483647, "Макс"=2147483647, "Сервис"=FALSE, "Только чтение"=FALSE, "Разработка"=FALSE, "К-во бит"=32, "Шаг"=0, "Обработка"=FALSE, "Макрос"=""}, {"Имя"="up5", "Группа"="up", "Наименование"="Переменная общего назначения 5", "Ед. изм"=0, "Список"="", "Адрес"=1797, "Описание"="Может использоваться для общих целей. Например, для запоминания длинны оси, приводимой в движение данным приводом и т.д.", "Мин"=-2147483647, "Макс"=2147483647, "Сервис"=FALSE, "Только чтение"=FALSE, "Разработка"=FALSE, "К-во бит"=32, "Шаг"=0, "Обработка"=FALSE, "Макрос"=""}, {"Имя"="up6", "Группа"="up", "Наименование"="Переменная общего назначения 6", "Ед. изм"=0, "Список"="", "Адрес"=1798, "Описание"="Может использоваться для общих целей. Например, для запоминания длинны оси, приводимой в движение данным приводом и т.д.", "Мин"=-2147483647, "Макс"=2147483647, "Сервис"=FALSE, "Только чтение"=FALSE, "Разработка"=FALSE, "К-во бит"=32, "Шаг"=0, "Обработка"=FALSE, "Макрос"=""}, {"Имя"="up7", "Группа"="up", "Наименование"="Переменная общего назначения 7", "Ед. изм"=0, "Список"="", "Адрес"=1799, "Описание"="Может использоваться для общих целей. Например, для запоминания длинны оси, приводимой в движение данным приводом и т.д.", "Мин"=-2147483647, "Макс"=2147483647, "Сервис"=FALSE, "Только чтение"=FALSE, "Разработка"=FALSE, "К-во бит"=32, "Шаг"=0, "Обработка"=FALSE, "Макрос"=""}, {"Имя"="st4", "Группа"="st", "Наименование"="Тип привода", "Ед. изм"=0, "Список"="1:СПШ10-23xx\n2:СПШ20-23xx\\1000Z\n4:СПШ20-23xx\\2000Z\n64:СПШ10-34xx\n128:СПШ20-34xx\\2000Z\n4096:СПШ20-34xx\\1000Z\n8192:СПС25-80007\n8193:СПС25-80016\n8194:СПС25-80025\n8195:СПС25-1100075\n8196:СПС30-хххх\n\r\n", "Адрес"=70, "Описание"="", "Мин"=1, "Макс"=65535, "Сервис"=FALSE, "Только чтение"=FALSE, "Разработка"=FALSE, "К-во бит"=16, "Шаг"=0, "Обработка"=FALSE, "Макрос"=""}, {"Имя"="st5", "Группа"="st", "Наименование"="Z метка", "Ед. изм"=0, "Список"="0:Нет\n1:Да\n\r\n", "Адрес"=71, "Описание"="Наличие или отсутствие у датчика позиции канала нуливой метки", "Мин"=0, "Макс"=1, "Сервис"=FALSE, "Только чтение"=FALSE, "Разработка"=FALSE, "К-во бит"=16, "Шаг"=0, "Обработка"=FALSE, "Макрос"=""}, {"Имя"="cp6", "Группа"="cp", "Наименование"="Вырабатываемый момент", "Ед. изм"=0, "Список"="100:100%\n75:75%\n50:50%\n25:25%\n\r\n", "Адрес"=72, "Описание"="Параметр позволяет ограничить развиваемый момент", "Мин"=25, "Макс"=100, "Сервис"=FALSE, "Только чтение"=FALSE, "Разработка"=TRUE, "К-во бит"=16, "Шаг"=0, "Обработка"=FALSE, "Макрос"=""}, {"Имя"="ep3", "Группа"="ep", "Наименование"="Ток поиска фазы", "Ед. изм"=1, "Список"="", "Адрес"=81, "Описание"="Определяет уровень тока, который устанавливается при поиске фазы. Ток задается в дискретах.", "Мин"=0, "Макс"=32000, "Сервис"=FALSE, "Только чтение"=FALSE, "Разработка"=FALSE, "К-во бит"=16, "Шаг"=1, "Обработка"=FALSE, "Макрос"=""}, {"Имя"="ep4", "Группа"="ep", "Наименование"="Время поиска фазы", "Ед. изм"=1, "Список"="", "Адрес"=82, "Описание"="Определяет время, в течение которого будет удерживаться ток ep3 при поиске фазы.", "Мин"=0, "Макс"=32000, "Сервис"=FALSE, "Только чтение"=FALSE, "Разработка"=FALSE, "К-во бит"=16, "Шаг"=1, "Обработка"=FALSE, "Макрос"=""}, {"Имя"="ep5", "Группа"="ep", "Наименование"="Максимальная температура", "Ед. изм"=7, "Список"="", "Адрес"=84, "Описание"="Указывает максимальную допустимую температуру внутри корпуса", "Мин"=25, "Макс"=85, "Сервис"=FALSE, "Только чтение"=FALSE, "Разработка"=FALSE, "К-во бит"=16, "Шаг"=1, "Обработка"=FALSE, "Макрос"=""}, {"Имя"="cp7", "Группа"="cp", "Наименование"="Модуляция ШИМ сигнала", "Ед. изм"=0, "Список"="0:Выключена\n1:Включена\n\r\n", "Адрес"=83, "Описание"="Разрешает/запрещает подачу силового напряжения на обмотки двигателя", "Мин"=0, "Макс"=1, "Сервис"=FALSE, "Только чтение"=FALSE, "Разработка"=FALSE, "К-во бит"=16, "Шаг"=0, "Обработка"=FALSE, "Макрос"=""}, {"Имя"="ep6", "Группа"="ep", "Наименование"="Период поиска фазы", "Ед. изм"=0, "Список"="0:Однопериодный\n1:1\n2:2\n3:3\n\r\n", "Адрес"=86, "Описание"="Один из трех периодов, во время которого привод может выполнять поиск фазы. В результате удается избежать перегрузки источника питания и выполнить корректный поиск фазы в приводах, между которыми имеется жесткая механическая связь.", "Мин"=0, "Макс"=3, "Сервис"=FALSE, "Только чтение"=FALSE, "Разработка"=FALSE, "К-во бит"=16, "Шаг"=1, "Обработка"=FALSE, "Макрос"=""}, {"Имя"="up8", "Группа"="up", "Наименование"="X", "Ед. изм"=0, "Список"="", "Адрес"=1800, "Описание"="Переменная, используемая в ПЛК", "Мин"=-2147483647, "Макс"=2147483647, "Сервис"=FALSE, "Только чтение"=FALSE, "Разработка"=FALSE, "К-во бит"=32, "Шаг"=1, "Обработка"=FALSE, "Макрос"=""}, {"Имя"="up9", "Группа"="up", "Наименование"="Y", "Ед. изм"=0, "Список"="", "Адрес"=1801, "Описание"="Переменная, используемая в ПЛК", "Мин"=-2147483647, "Макс"=2147483647, "Сервис"=FALSE, "Только чтение"=FALSE, "Разработка"=FALSE, "К-во бит"=32, "Шаг"=1, "Обработка"=FALSE, "Макрос"=""}, {"Имя"="up10", "Группа"="up", "Наименование"="Z", "Ед. изм"=0, "Список"="", "Адрес"=1802, "Описание"="Переменная, используемая в ПЛК", "Мин"=-2147483647, "Макс"=2147483647, "Сервис"=FALSE, "Только чтение"=FALSE, "Разработка"=FALSE, "К-во бит"=32, "Шаг"=1, "Обработка"=FALSE, "Макрос"=""}, {"Имя"="up11", "Группа"="up", "Наименование"="EEPROM массив", "Ед. изм"=0, "Список"="", "Адрес"=1803, "Описание"="User EEPROM massive", "Мин"=-2147483647, "Макс"=2147483647, "Сервис"=FALSE, "Только чтение"=FALSE, "Разработка"=TRUE, "К-во бит"=32, "Шаг"=1, "Обработка"=FALSE, "Макрос"=""}, {"Имя"="up12", "Группа"="up", "Наименование"="EEPROM массив метаданных", "Ед. изм"=0, "Список"="", "Адрес"=1804, "Описание"="Metadata massive of params of motor", "Мин"=-2147483647, "Макс"=2147483647, "Сервис"=FALSE, "Только чтение"=FALSE, "Разработка"=TRUE, "К-во бит"=32, "Шаг"=1, "Обработка"=FALSE, "Макрос"=""}, {"Имя"="dd22", "Группа"="dd", "Наименование"="Максимальное отклонение от траектории", "Ед. изм"=1, "Список"="", "Адрес"=1056, "Описание"="Определяет максимальную ошибку контура позиции зафиксированную при прохождении траектории.", "Мин"=0, "Макс"=65535, "Сервис"=FALSE, "Только чтение"=FALSE, "Разработка"=FALSE, "К-во бит"=16, "Шаг"=0, "Обработка"=FALSE, "Макрос"=""}, {"Имя"="ip13", "Группа"="ip", "Наименование"="Ограничитель левый", "Ед. изм"=6, "Список"="", "Адрес"=87, "Описание"="Программный ограничитель позиции,  при достижении которой привод останавливается и воспринимает команду управления только в противоположную сторону.", "Мин"=-2147483647, "Макс"=2147483647, "Сервис"=FALSE, "Только чтение"=FALSE, "Разработка"=FALSE, "К-во бит"=32, "Шаг"=0, "Обработка"=FALSE, "Макрос"=""}, {"Имя"="ip14", "Группа"="ip", "Наименование"="Ограничитель правый", "Ед. изм"=6, "Список"="", "Адрес"=88, "Описание"="Программный ограничитель позиции,  при достижении которой привод останавливается и воспринимает команду управления только в противоположную сторону.", "Мин"=-2147483647, "Макс"=2147483647, "Сервис"=FALSE, "Только чтение"=FALSE, "Разработка"=FALSE, "К-во бит"=32, "Шаг"=0, "Обработка"=FALSE, "Макрос"=""}, {"Имя"="dd23", "Группа"="dd", "Наименование"="Статус G декодера", "Ед. изм"=0, "Список"="0:Останов\n1:Начало\n2:Отработка\n3:Ожидание подтверждений\n4:Ошибка\n5:Выход в нуль\r\n", "Адрес"=1057, "Описание"="", "Мин"=0, "Макс"=5, "Сервис"=FALSE, "Только чтение"=TRUE, "Разработка"=TRUE, "К-во бит"=16, "Шаг"=0, "Обработка"=FALSE, "Макрос"=""}, {"Имя"="dd24", "Группа"="dd", "Наименование"="Текущий кадр G декодера", "Ед. изм"=0, "Список"="", "Адрес"=1058, "Описание"="", "Мин"=0, "Макс"=65535, "Сервис"=FALSE, "Только чтение"=TRUE, "Разработка"=TRUE, "К-во бит"=16, "Шаг"=0, "Обработка"=FALSE, "Макрос"=""}, {"Имя"="ip15", "Группа"="ip", "Наименование"="Скорость обмена по шине CAN", "Ед. изм"=0, "Список"="500:500 кБит/сек\n1000:1000 кБит/сек\n\r\n", "Адрес"=89, "Описание"="Определяет скорость обмена по шине CAN. При этом допустимая скорость определяется дальностью линии связи. На скорость 1000кБит максимальная дальность 60м, 500кБит - 120м", "Мин"=50, "Макс"=1000, "Сервис"=FALSE, "Только чтение"=FALSE, "Разработка"=FALSE, "К-во бит"=16, "Шаг"=0, "Обработка"=FALSE, "Макрос"=""}, {"Имя"="cp8", "Группа"="cp", "Наименование"="Частота ШИМ сигнала", "Ед. изм"=12, "Список"="2500:40кГц\n5000:20кГц\n6250:16кГц\n12500:8кГц\n25000:4кГц\n\r\n", "Адрес"=96, "Описание"="Определяет частоту ШИМ сигнала и частоту работы контура тока. Влияет на КПД силовой части привода, а также качество работы контура тока. Для приводов серии СПШ частота всегда 40кГц. Влияет на параметр cp4.", "Мин"=-65535, "Макс"=65535, "Сервис"=FALSE, "Только чтение"=FALSE, "Разработка"=FALSE, "К-во бит"=16, "Шаг"=0, "Обработка"=FALSE, "Макрос"=""}, {"Имя"="ip16", "Группа"="ip", "Наименование"="USB2CAN конвертор", "Ед. изм"=0, "Список"="0:Выкл\n2:Вкл\n\r\n", "Адрес"=97, "Описание"="Данная функция предназначена для облегчения подключения к группе приводов СПШ/СПС, которые объединены в рамках системы в одну сеть CAN. Чтобы работать со всеми приводами сети достаточно подключиться только к одному приводу по USB.", "Мин"=0, "Макс"=2, "Сервис"=FALSE, "Только чтение"=FALSE, "Разработка"=FALSE, "К-во бит"=16, "Шаг"=0, "Обработка"=FALSE, "Макрос"=""}, {"Имя"="up13", "Группа"="up", "Наименование"="Значение текущего элемента EEPROM массива", "Ед. изм"=0, "Список"="", "Адрес"=1805, "Описание"="Отображает значение текущего элемента массива энергонезависимой памяти данных общего назначения.", "Мин"=-2147483647, "Макс"=2147483647, "Сервис"=FALSE, "Только чтение"=FALSE, "Разработка"=FALSE, "К-во бит"=32, "Шаг"=1, "Обработка"=FALSE, "Макрос"=""}, {"Имя"="up14", "Группа"="up", "Наименование"="Индекс текущего элемента EEPROM массива", "Ед. изм"=0, "Список"="", "Адрес"=1806, "Описание"="Отображает индекс текущего элемента массива энергонезависимой памяти данных общего назначения.", "Мин"=-2147483647, "Макс"=2147483647, "Сервис"=FALSE, "Только чтение"=FALSE, "Разработка"=FALSE, "К-во бит"=32, "Шаг"=1, "Обработка"=FALSE, "Макрос"=""}, {"Имя"="up15", "Группа"="up", "Наименование"="Значение счетчика импульсов", "Ед. изм"=0, "Список"="", "Адрес"=1807, "Описание"="Отображает значение счетчика импульсов, которые приходят на порты IN0, IN1, по протоколу Step\\Dir или по квадратурному протоколу. Счетчик активизирован только при выборе соответствующего протокола.", "Мин"=-2147483647, "Макс"=2147483647, "Сервис"=FALSE, "Только чтение"=FALSE, "Разработка"=FALSE, "К-во бит"=32, "Шаг"=1, "Обработка"=FALSE, "Макрос"=""}, {"Имя"="up16", "Группа"="up", "Наименование"="Среднее значение заданного тока", "Ед. изм"=0, "Список"="", "Адрес"=1808, "Описание"="Величина пропорциональна вырабатываемому приводом моменту, используется в программах для определения развиваемого момента.", "Мин"=-65535, "Макс"=65535, "Сервис"=FALSE, "Только чтение"=TRUE, "Разработка"=FALSE, "К-во бит"=16, "Шаг"=1, "Обработка"=FALSE, "Макрос"=""}, {"Имя"="ip17", "Группа"="ip", "Наименование"="Таймаут передачи синхронизации слейву", "Ед. изм"=9, "Список"="", "Адрес"=2048, "Описание"="Временной интервал, в течение которого мастер обязан передать синхронизацию слейву. По истечении этого времени параметр ip10 будет установлен в значение 1 или 2.", "Мин"=0, "Макс"=10000, "Сервис"=FALSE, "Только чтение"=FALSE, "Разработка"=FALSE, "К-во бит"=16, "Шаг"=25, "Обработка"=FALSE, "Макрос"=""}, {"Имя"="ip18", "Группа"="ip", "Наименование"="Таймаут передачи подтверждения мастеру от слейва", "Ед. изм"=9, "Список"="", "Адрес"=2049, "Описание"="Временной интервал, в течение которого слейв обязан передать подтверждение на команду синхронизации мастеру. По истечении этого времени параметр ip10 будет установлен в значение 3.", "Мин"=0, "Макс"=10000, "Сервис"=FALSE, "Только чтение"=FALSE, "Разработка"=FALSE, "К-во бит"=16, "Шаг"=25, "Обработка"=FALSE, "Макрос"=""}, {"Имя"="st6", "Группа"="st", "Наименование"="Нулевой сектор сигналов UVW", "Ед. изм"=0, "Список"="1:1\n2:2\n3:3\n4:4\n5:5\n6:6\n170:Выполнить инициализацию\n85:Не использовать UVW треки\n\r\n", "Адрес"=2050, "Описание"="Определяет сектор датчика UVW, в котором находится нуль двигателя. Если установить значение \"Выполнить инициализацию\", то при следующем запуске автоматически будет выполнена операция поиска сектора и смещения внутри сектора", "Мин"=0, "Макс"=170, "Сервис"=FALSE, "Только чтение"=FALSE, "Разработка"=FALSE, "К-во бит"=16, "Шаг"=0, "Обработка"=FALSE, "Макрос"=""}, {"Имя"="st7", "Группа"="st", "Наименование"="Сдвиг нуля внутри сектора сигналов UVW", "Ед. изм"=0, "Список"="", "Адрес"=2052, "Описание"="Определяет смещение внутри сектора датчика UVW, в котором находится нуль двигателя. Если установить значение \"Выполнить инициализацию\", то при следующем запуске автоматически будет выполнена операция поиска сектора и смещения внутри сектора", "Мин"=0, "Макс"=80000, "Сервис"=FALSE, "Только чтение"=FALSE, "Разработка"=FALSE, "К-во бит"=16, "Шаг"=0, "Обработка"=FALSE, "Макрос"=""}, {"Имя"="io0", "Группа"="io", "Наименование"="Порт ввода 0", "Ед. изм"=0, "Список"="", "Адрес"=2053, "Описание"="Значение порта ввода 0", "Мин"=0, "Макс"=1, "Сервис"=FALSE, "Только чтение"=FALSE, "Разработка"=FALSE, "К-во бит"=16, "Шаг"=0, "Обработка"=FALSE, "Макрос"=""}, {"Имя"="io1", "Группа"="io", "Наименование"="Порт ввода 1", "Ед. изм"=0, "Список"="", "Адрес"=2054, "Описание"="Значение порта ввода 1", "Мин"=0, "Макс"=1, "Сервис"=FALSE, "Только чтение"=FALSE, "Разработка"=FALSE, "К-во бит"=16, "Шаг"=0, "Обработка"=FALSE, "Макрос"=""}, {"Имя"="io2", "Группа"="io", "Наименование"="Порт ввода 2", "Ед. изм"=0, "Список"="", "Адрес"=2055, "Описание"="Значение порта ввода 2", "Мин"=0, "Макс"=1, "Сервис"=FALSE, "Только чтение"=FALSE, "Разработка"=FALSE, "К-во бит"=16, "Шаг"=0, "Обработка"=FALSE, "Макрос"=""}, {"Имя"="io3", "Группа"="io", "Наименование"="Порт ввода 3", "Ед. изм"=0, "Список"="", "Адрес"=2056, "Описание"="Значение порта ввода 3", "Мин"=0, "Макс"=1, "Сервис"=FALSE, "Только чтение"=FALSE, "Разработка"=FALSE, "К-во бит"=16, "Шаг"=0, "Обработка"=FALSE, "Макрос"=""}, {"Имя"="io4", "Группа"="io", "Наименование"="Порт вывода 0", "Ед. изм"=0, "Список"="", "Адрес"=2057, "Описание"="Значение порта вывода 0", "Мин"=0, "Макс"=1, "Сервис"=FALSE, "Только чтение"=FALSE, "Разработка"=FALSE, "К-во бит"=16, "Шаг"=0, "Обработка"=FALSE, "Макрос"=""}, {"Имя"="io5", "Группа"="io", "Наименование"="Порт вывода 1", "Ед. изм"=0, "Список"="", "Адрес"=2058, "Описание"="Значение порта вывода 1", "Мин"=0, "Макс"=1, "Сервис"=FALSE, "Только чтение"=FALSE, "Разработка"=FALSE, "К-во бит"=16, "Шаг"=0, "Обработка"=FALSE, "Макрос"=""}, {"Имя"="io6", "Группа"="io", "Наименование"="PWM0", "Ед. изм"=0, "Список"="", "Адрес"=2059, "Описание"="Скваженность ШИМ сигнала, выводимого на порт вывода 0. Порт необходимо соответствующим образом настроить с помощью параметра: Режим работы порта вывода.", "Мин"=0, "Макс"=160, "Сервис"=FALSE, "Только чтение"=FALSE, "Разработка"=FALSE, "К-во бит"=16, "Шаг"=1, "Обработка"=FALSE, "Макрос"=""}, {"Имя"="io7", "Группа"="io", "Наименование"="PWM1", "Ед. изм"=0, "Список"="", "Адрес"=2060, "Описание"="Скваженность ШИМ сигнала, выводимого на порт вывода 1. Порт необходимо соответствующим образом настроить с помощью параметра: Режим работы порта вывода.", "Мин"=0, "Макс"=160, "Сервис"=FALSE, "Только чтение"=FALSE, "Разработка"=FALSE, "К-во бит"=16, "Шаг"=1, "Обработка"=FALSE, "Макрос"=""}, {"Имя"="io8", "Группа"="io", "Наименование"="Режим порта ввода 0", "Ед. изм"=0, "Список"="0:Порт ввода общего назначения\n1:Порт ввода в режиме квадратурного счетчика\n2:Порт ввода в режиме счетчика Step/dir\n\r\n", "Адрес"=2061, "Описание"="Определяет режим работы порта ввода.", "Мин"=0, "Макс"=3, "Сервис"=FALSE, "Только чтение"=FALSE, "Разработка"=FALSE, "К-во бит"=16, "Шаг"=1, "Обработка"=FALSE, "Макрос"=""}, {"Имя"="io9", "Группа"="io", "Наименование"="Режим порта ввода 1", "Ед. изм"=0, "Список"="0:Порт ввода общего назначения\n1:Порт ввода в режиме квадратурного счетчика\n2:Порт ввода в режиме счетчика Step/dir\n\r\n", "Адрес"=2062, "Описание"="Определяет режим работы порта ввода.", "Мин"=0, "Макс"=3, "Сервис"=FALSE, "Только чтение"=FALSE, "Разработка"=FALSE, "К-во бит"=16, "Шаг"=1, "Обработка"=FALSE, "Макрос"=""}, {"Имя"="io10", "Группа"="io", "Наименование"="Режим порта ввода 2", "Ед. изм"=0, "Список"="0:Порт ввода общего назначения\n1:Порт ввода в режиме квадратурного счетчика\n2:Порт ввода в режиме счетчика Step/dir\n\r\n", "Адрес"=2063, "Описание"="Определяет режим работы порта ввода.", "Мин"=0, "Макс"=3, "Сервис"=FALSE, "Только чтение"=FALSE, "Разработка"=FALSE, "К-во бит"=16, "Шаг"=1, "Обработка"=FALSE, "Макрос"=""}, {"Имя"="io11", "Группа"="io", "Наименование"="Режим порта ввода 3", "Ед. изм"=0, "Список"="0:Порт ввода общего назначения\n1:Порт ввода в режиме квадратурного счетчика\n2:Порт ввода в режиме счетчика Step/dir\n\r\n", "Адрес"=2064, "Описание"="Определяет режим работы порта ввода.", "Мин"=0, "Макс"=3, "Сервис"=FALSE, "Только чтение"=FALSE, "Разработка"=FALSE, "К-во бит"=16, "Шаг"=1, "Обработка"=FALSE, "Макрос"=""}, {"Имя"="io12", "Группа"="io", "Наименование"="Режим порта вывода 0", "Ед. изм"=0, "Список"="0:Порт вывода общего назначения\n1:Порт вывода в режиме ШИМ\n\r\n", "Адрес"=2065, "Описание"="Определяет режим работы порта вывода.", "Мин"=0, "Макс"=3, "Сервис"=FALSE, "Только чтение"=FALSE, "Разработка"=FALSE, "К-во бит"=16, "Шаг"=1, "Обработка"=FALSE, "Макрос"=""}, {"Имя"="io13", "Группа"="io", "Наименование"="Режим порта вывода 1", "Ед. изм"=0, "Список"="0:Порт вывода общего назначения\n1:Порт вывода в режиме ШИМ\n\r\n", "Адрес"=2066, "Описание"="Определяет режим работы порта вывода.", "Мин"=0, "Макс"=3, "Сервис"=FALSE, "Только чтение"=FALSE, "Разработка"=FALSE, "К-во бит"=16, "Шаг"=1, "Обработка"=FALSE, "Макрос"=""}, {"Имя"="io14", "Группа"="io", "Наименование"="Счетчик импульсов", "Ед. изм"=0, "Список"="", "Адрес"=1807, "Описание"="Аппаратный счетчик импульсов,  которые приходят на входы In0 и In1. При этом порты должны быть настроены на соответствующий интерфейс (см. параметры io8 и io9).", "Мин"=-2147483647, "Макс"=2147483647, "Сервис"=FALSE, "Только чтение"=TRUE, "Разработка"=FALSE, "К-во бит"=32, "Шаг"=1, "Обработка"=FALSE, "Макрос"=""}, {"Имя"="dd25", "Группа"="dd", "Наименование"="UVW треки", "Ед. изм"=0, "Список"="", "Адрес"=1059, "Описание"="Сигнал, считанный с UVW треков энкодера", "Мин"=0, "Макс"=16, "Сервис"=FALSE, "Только чтение"=TRUE, "Разработка"=FALSE, "К-во бит"=16, "Шаг"=0, "Обработка"=FALSE, "Макрос"=""}, {"Имя"="st8", "Группа"="st", "Наименование"="Тип энкодера", "Ед. изм"=0, "Список"="0:Инкрементальный\n1:Абсолютный\n\r\n", "Адрес"=98, "Описание"="", "Мин"=0, "Макс"=1, "Сервис"=FALSE, "Только чтение"=FALSE, "Разработка"=FALSE, "К-во бит"=32, "Шаг"=1, "Обработка"=FALSE, "Макрос"=""}, {"Имя"="vp17", "Группа"="vp", "Наименование"="Рывок", "Ед. изм"=0, "Список"="", "Адрес"=99, "Описание"="Ограничивает вторую производную скорости. Параметр вступает в силу только при установки vp9 в значение 4", "Мин"=1, "Макс"=21470, "Сервис"=TRUE, "Только чтение"=FALSE, "Разработка"=FALSE, "К-во бит"=32, "Шаг"=10, "Обработка"=FALSE, "Макрос"=""}, {"Имя"="cp9", "Группа"="cp", "Наименование"="Допустимая перегрузка", "Ед. изм"=13, "Список"="", "Адрес"=2068, "Описание"="Ограничение выделяемой мощности обмотками двигателя. Предотвращает повреждения обмоток. Реализует защитную функцию I2t", "Мин"=0, "Макс"=350, "Сервис"=TRUE, "Только чтение"=FALSE, "Разработка"=FALSE, "К-во бит"=32, "Шаг"=16, "Обработка"=FALSE, "Макрос"=""}, {"Имя"="cp10", "Группа"="cp", "Наименование"="Номинальный ток", "Ед. изм"=5, "Список"="", "Адрес"=2069, "Описание"="", "Мин"=0, "Макс"=850, "Сервис"=TRUE, "Только чтение"=FALSE, "Разработка"=FALSE, "К-во бит"=32, "Шаг"=16, "Обработка"=TRUE, "Макрос"="macros cp10\n  ON_READ\n  READ cp3\n  cp3=cp3*5/2047\n  RETURN cp3\n  ON_WRITE\n  cp3=val*66\n  WRITE cp3\nend"}, {"Имя"="dd26", "Группа"="dd", "Наименование"="Текущая перегрузка", "Ед. изм"=13, "Список"="", "Адрес"=1060, "Описание"="Накомпленнае мощность, превышающая номинальные характеристики двигателя", "Мин"=0, "Макс"=100, "Сервис"=TRUE, "Только чтение"=TRUE, "Разработка"=FALSE, "К-во бит"=32, "Шаг"=16, "Обработка"=FALSE, "Макрос"=""}, {"Имя"="dd27", "Группа"="dd", "Наименование"="Ток в обмотке 3", "Ед. изм"=5, "Список"="", "Адрес"=1061, "Описание"="Показывает ток, протекающий в обмотке двигателя. Параметр действителен только для СПС.", "Мин"=-5, "Макс"=5, "Сервис"=FALSE, "Только чтение"=TRUE, "Разработка"=FALSE, "К-во бит"=16, "Шаг"=0, "Обработка"=TRUE, "Макрос"="macros dd27\n  ON_READ\n  READ dd1\n  dd1=dd1*5/2047\n  RETURN dd1\n  ON_WRITE\n  dd1=val*2047/5\n  WRITE dd1\nend"}, {"Имя"="dd28", "Группа"="dd", "Наименование"="Заданный ток в обмотке 3", "Ед. изм"=5, "Список"="", "Адрес"=1062, "Описание"="Заданный ток в обмотке 3. Действителен только для приводов серии СПС.", "Мин"=-2047, "Макс"=2047, "Сервис"=FALSE, "Только чтение"=FALSE, "Разработка"=FALSE, "К-во бит"=16, "Шаг"=0, "Обработка"=TRUE, "Макрос"="macros dd28\n  ON_READ\n  READ dd6\n  dd6=dd6/74\n  RETURN dd6\n  ON_WRITE\n  dd6=val*74\n  WRITE dd6\nend"}, {"Имя"="dd29", "Группа"="dd", "Наименование"="Ток потребления двигателя", "Ед. изм"=5, "Список"="", "Адрес"=1063, "Описание"="Параметр действителен только для СПС.", "Мин"=-5, "Макс"=5, "Сервис"=FALSE, "Только чтение"=TRUE, "Разработка"=FALSE, "К-во бит"=16, "Шаг"=0, "Обработка"=TRUE, "Макрос"="macros dd29\n  ON_READ\n  READ dd1\n  dd1=dd1/74\n  RETURN dd1\n  ON_WRITE\n  dd1=val*74\n  WRITE dd1\nend"}, {"Имя"="pd1", "Группа"="pd", "Наименование"="Зона нечувствительности", "Ед. изм"=0, "Список"="", "Адрес"=2561, "Описание"="Параметр настройки ПИД-регулятора", "Мин"=0, "Макс"=10000, "Сервис"=TRUE, "Только чтение"=FALSE, "Разработка"=FALSE, "К-во бит"=32, "Шаг"=12, "Обработка"=FALSE, "Макрос"=""}, {"Имя"="pd2", "Группа"="pd", "Наименование"="Максимальная ошибка", "Ед. изм"=0, "Список"="", "Адрес"=2562, "Описание"="Параметр настройки ПИД-регулятора", "Мин"=0, "Макс"=524287, "Сервис"=TRUE, "Только чтение"=FALSE, "Разработка"=FALSE, "К-во бит"=32, "Шаг"=12, "Обработка"=FALSE, "Макрос"=""}, {"Имя"="pd3", "Группа"="pd", "Наименование"="Пропорциональный коэффициент", "Ед. изм"=0, "Список"="", "Адрес"=2563, "Описание"="Параметр настройки ПИД-регулятора", "Мин"=0, "Макс"=10000, "Сервис"=TRUE, "Только чтение"=FALSE, "Разработка"=FALSE, "К-во бит"=32, "Шаг"=12, "Обработка"=FALSE, "Макрос"=""}, {"Имя"="pd4", "Группа"="pd", "Наименование"="Интегральный коэффициент", "Ед. изм"=0, "Список"="", "Адрес"=2564, "Описание"="Параметр настройки ПИД-регулятора", "Мин"=0, "Макс"=10000, "Сервис"=TRUE, "Только чтение"=FALSE, "Разработка"=FALSE, "К-во бит"=32, "Шаг"=12, "Обработка"=FALSE, "Макрос"=""}, {"Имя"="pd5", "Группа"="pd", "Наименование"="Дифференциальный коэффициент", "Ед. изм"=0, "Список"="", "Адрес"=2565, "Описание"="Параметр настройки ПИД-регулятора", "Мин"=0, "Макс"=10000, "Сервис"=TRUE, "Только чтение"=FALSE, "Разработка"=FALSE, "К-во бит"=32, "Шаг"=12, "Обработка"=FALSE, "Макрос"=""}, {"Имя"="pd6", "Группа"="pd", "Наименование"="Ограничение интегральной составляющей", "Ед. изм"=0, "Список"="", "Адрес"=2566, "Описание"="Параметр настройки ПИД-регулятора", "Мин"=0, "Макс"=100000, "Сервис"=TRUE, "Только чтение"=FALSE, "Разработка"=FALSE, "К-во бит"=32, "Шаг"=12, "Обработка"=FALSE, "Макрос"=""}, {"Имя"="pd7", "Группа"="pd", "Наименование"="Ограничение дифференциальной составляющей", "Ед. изм"=0, "Список"="", "Адрес"=2567, "Описание"="Параметр настройки ПИД-регулятора", "Мин"=0, "Макс"=100000, "Сервис"=TRUE, "Только чтение"=FALSE, "Разработка"=FALSE, "К-во бит"=32, "Шаг"=12, "Обработка"=FALSE, "Макрос"=""}, {"Имя"="pd8", "Группа"="pd", "Наименование"="Ограничение форсирующей составляющей 1го порядка", "Ед. изм"=0, "Список"="", "Адрес"=2568, "Описание"="Параметр настройки ПИД-регулятора", "Мин"=0, "Макс"=524287, "Сервис"=TRUE, "Только чтение"=FALSE, "Разработка"=FALSE, "К-во бит"=32, "Шаг"=12, "Обработка"=FALSE, "Макрос"=""}, {"Имя"="pd9", "Группа"="pd", "Наименование"="Ограничение форсирующей составляющей 2го порядка", "Ед. изм"=0, "Список"="", "Адрес"=2569, "Описание"="Параметр настройки ПИД-регулятора", "Мин"=0, "Макс"=524287, "Сервис"=TRUE, "Только чтение"=FALSE, "Разработка"=FALSE, "К-во бит"=32, "Шаг"=12, "Обработка"=FALSE, "Макрос"=""}, {"Имя"="pd10", "Группа"="pd", "Наименование"="Коэффициент форсирующей составляющей 0го порядка", "Ед. изм"=0, "Список"="", "Адрес"=2570, "Описание"="Параметр настройки ПИД-регулятора", "Мин"=0, "Макс"=10000, "Сервис"=TRUE, "Только чтение"=FALSE, "Разработка"=FALSE, "К-во бит"=32, "Шаг"=12, "Обработка"=FALSE, "Макрос"=""}, {"Имя"="pd11", "Группа"="pd", "Наименование"="Коэффициент форсирующей составляющей 1го порядка", "Ед. изм"=0, "Список"="", "Адрес"=2571, "Описание"="Параметр настройки ПИД-регулятора", "Мин"=0, "Макс"=10000, "Сервис"=TRUE, "Только чтение"=FALSE, "Разработка"=FALSE, "К-во бит"=32, "Шаг"=12, "Обработка"=FALSE, "Макрос"=""}, {"Имя"="pd12", "Группа"="pd", "Наименование"="Коэффициент форсирующей составляющей 2го порядка", "Ед. изм"=0, "Список"="", "Адрес"=2572, "Описание"="Параметр настройки ПИД-регулятора", "Мин"=0, "Макс"=10000, "Сервис"=TRUE, "Только чтение"=FALSE, "Разработка"=FALSE, "К-во бит"=32, "Шаг"=12, "Обработка"=FALSE, "Макрос"=""}, {"Имя"="pd13", "Группа"="pd", "Наименование"="Смещение сигнала управления", "Ед. изм"=0, "Список"="", "Адрес"=2573, "Описание"="Параметр настройки ПИД-регулятора", "Мин"=-524286, "Макс"=524287, "Сервис"=TRUE, "Только чтение"=FALSE, "Разработка"=FALSE, "К-во бит"=32, "Шаг"=12, "Обработка"=FALSE, "Макрос"=""}, {"Имя"="pd14", "Группа"="pd", "Наименование"="Ограничение выходного сигнала", "Ед. изм"=0, "Список"="", "Адрес"=2574, "Описание"="Параметр настройки ПИД-регулятора", "Мин"=0, "Макс"=524287, "Сервис"=TRUE, "Только чтение"=FALSE, "Разработка"=FALSE, "К-во бит"=32, "Шаг"=12, "Обработка"=FALSE, "Макрос"=""}, {"Имя"="pd15", "Группа"="pd", "Наименование"="Задание регулятора", "Ед. изм"=0, "Список"="", "Адрес"=2575, "Описание"="Параметр настройки ПИД-регулятора", "Мин"=-524286, "Макс"=524287, "Сервис"=TRUE, "Только чтение"=FALSE, "Разработка"=FALSE, "К-во бит"=32, "Шаг"=12, "Обработка"=FALSE, "Макрос"=""}, {"Имя"="pd16", "Группа"="pd", "Наименование"="Обратная связь", "Ед. изм"=0, "Список"="", "Адрес"=2576, "Описание"="Параметр настройки ПИД-регулятора", "Мин"=-524286, "Макс"=524287, "Сервис"=TRUE, "Только чтение"=TRUE, "Разработка"=FALSE, "К-во бит"=32, "Шаг"=12, "Обработка"=FALSE, "Макрос"=""}, {"Имя"="pd17", "Группа"="pd", "Наименование"="Ошибка", "Ед. изм"=0, "Список"="", "Адрес"=2577, "Описание"="Параметр настройки ПИД-регулятора", "Мин"=-524286, "Макс"=524287, "Сервис"=TRUE, "Только чтение"=TRUE, "Разработка"=FALSE, "К-во бит"=32, "Шаг"=12, "Обработка"=FALSE, "Макрос"=""}, {"Имя"="pp7", "Группа"="pp", "Наименование"="Ограничение форсирующей составляющей 1го порядка", "Ед. изм"=0, "Список"="", "Адрес"=2578, "Описание"="Параметр настройки ПИД-регулятора", "Мин"=0, "Макс"=524287, "Сервис"=TRUE, "Только чтение"=FALSE, "Разработка"=FALSE, "К-во бит"=32, "Шаг"=10, "Обработка"=FALSE, "Макрос"=""}, {"Имя"="pp8", "Группа"="pp", "Наименование"="Ограничение форсирующей составляющей 2го порядка", "Ед. изм"=0, "Список"="", "Адрес"=2579, "Описание"="Параметр настройки ПИД-регулятора", "Мин"=0, "Макс"=524287, "Сервис"=TRUE, "Только чтение"=FALSE, "Разработка"=FALSE, "К-во бит"=32, "Шаг"=10, "Обработка"=FALSE, "Макрос"=""}, {"Имя"="pp9", "Группа"="pp", "Наименование"="Коэффициент форсирующей составляющей 1го порядка", "Ед. изм"=0, "Список"="", "Адрес"=2580, "Описание"="Параметр настройки ПИД-регулятора", "Мин"=0, "Макс"=100000, "Сервис"=TRUE, "Только чтение"=FALSE, "Разработка"=FALSE, "К-во бит"=32, "Шаг"=10, "Обработка"=FALSE, "Макрос"=""}, {"Имя"="pp10", "Группа"="pp", "Наименование"="Коэффициент форсирующей составляющей 2го порядка", "Ед. изм"=0, "Список"="", "Адрес"=2581, "Описание"="Параметр настройки ПИД-регулятора", "Мин"=0, "Макс"=100000, "Сервис"=TRUE, "Только чтение"=FALSE, "Разработка"=FALSE, "К-во бит"=32, "Шаг"=10, "Обработка"=FALSE, "Макрос"=""}, {"Имя"="vp18", "Группа"="vp", "Наименование"="Зона нечувствительности входного сигнала", "Ед. изм"=0, "Список"="", "Адрес"=2582, "Описание"="Параметр настройки ПИ-регулятора контура скорости", "Мин"=0, "Макс"=60000, "Сервис"=TRUE, "Только чтение"=FALSE, "Разработка"=FALSE, "К-во бит"=32, "Шаг"=12, "Обработка"=FALSE, "Макрос"=""}, {"Имя"="vp19", "Группа"="vp", "Наименование"="Максимальная ошибка", "Ед. изм"=0, "Список"="", "Адрес"=2583, "Описание"="Параметр настройки ПИ-регулятора контура скорости", "Мин"=0, "Макс"=60000, "Сервис"=TRUE, "Только чтение"=FALSE, "Разработка"=FALSE, "К-во бит"=32, "Шаг"=12, "Обработка"=FALSE, "Макрос"=""}, {"Имя"="vp20", "Группа"="vp", "Наименование"="Ограничение форсирующей связи 1го порядка", "Ед. изм"=0, "Список"="", "Адрес"=2584, "Описание"="Параметр настройки ПИ-регулятора контура скорости", "Мин"=0, "Макс"=524287, "Сервис"=TRUE, "Только чтение"=FALSE, "Разработка"=FALSE, "К-во бит"=32, "Шаг"=12, "Обработка"=FALSE, "Макрос"=""}, {"Имя"="vp21", "Группа"="vp", "Наименование"="Ограничение форсирующей связи 2го порядка", "Ед. изм"=0, "Список"="", "Адрес"=2585, "Описание"="Параметр настройки ПИ-регулятора контура скорости", "Мин"=0, "Макс"=524287, "Сервис"=TRUE, "Только чтение"=FALSE, "Разработка"=FALSE, "К-во бит"=32, "Шаг"=12, "Обработка"=FALSE, "Макрос"=""}, {"Имя"="vp22", "Группа"="vp", "Наименование"="Коэффициент форсирующей связи 0го порядка", "Ед. изм"=0, "Список"="", "Адрес"=2586, "Описание"="Параметр настройки ПИ-регулятора контура скорости", "Мин"=0, "Макс"=60000, "Сервис"=TRUE, "Только чтение"=FALSE, "Разработка"=FALSE, "К-во бит"=32, "Шаг"=12, "Обработка"=FALSE, "Макрос"=""}, {"Имя"="vp23", "Группа"="vp", "Наименование"="Коэффициент форсирующей связи 1го порядка", "Ед. изм"=0, "Список"="", "Адрес"=2587, "Описание"="Параметр настройки ПИ-регулятора контура скорости", "Мин"=0, "Макс"=60000, "Сервис"=TRUE, "Только чтение"=FALSE, "Разработка"=FALSE, "К-во бит"=32, "Шаг"=12, "Обработка"=FALSE, "Макрос"=""}, {"Имя"="vp24", "Группа"="vp", "Наименование"="Коэффициент форсирующей связи 2го порядка", "Ед. изм"=0, "Список"="", "Адрес"=2588, "Описание"="Параметр настройки ПИ-регулятора контура скорости", "Мин"=0, "Макс"=60000, "Сервис"=TRUE, "Только чтение"=FALSE, "Разработка"=FALSE, "К-во бит"=32, "Шаг"=12, "Обработка"=FALSE, "Макрос"=""}, {"Имя"="st9", "Группа"="st", "Наименование"="Линейный энкодер", "Ед. изм"=0, "Список"="0:Нет\n1:Да\n\r\n", "Адрес"=2070, "Описание"="Если параметр установлен в Да, то будет использоваться внешний по отношению к приводу линейный энкодер для замыкания контура позиции. При этом контуры тока и скорости будут работать, по прежнему, от внутреннего энкодера.", "Мин"=0, "Макс"=1, "Сервис"=FALSE, "Только чтение"=FALSE, "Разработка"=FALSE, "К-во бит"=16, "Шаг"=0, "Обработка"=FALSE, "Макрос"=""}, {"Имя"="st10", "Группа"="st", "Наименование"="Разрешение линейного энкодера", "Ед. изм"=1, "Список"="", "Адрес"=2071, "Описание"="Разрешение линейного энкодера на оборот вала двигателя", "Мин"=-524286, "Макс"=524286, "Сервис"=TRUE, "Только чтение"=FALSE, "Разработка"=FALSE, "К-во бит"=32, "Шаг"=12, "Обработка"=FALSE, "Макрос"=""}, {"Имя"="dd30", "Группа"="dd", "Наименование"="Разница между внешним и внутренним энкодерами", "Ед. изм"=1, "Список"="", "Адрес"=1064, "Описание"="Разница между внешним и внутренним энкодерами с приведением к разрешению внутреннего", "Мин"=-524286, "Макс"=524286, "Сервис"=TRUE, "Только чтение"=TRUE, "Разработка"=FALSE, "К-во бит"=32, "Шаг"=12, "Обработка"=FALSE, "Макрос"=""}, {"Имя"="ss16", "Группа"="ss", "Наименование"="Счетчик потерь синхронизации", "Ед. изм"=0, "Список"="", "Адрес"=2072, "Описание"="Показывает сколько было потеряно команд SYNC=0x02 по шине CAN. Счетчик работает только, если выбран один из возможных режимов синхронизации.", "Мин"=0, "Макс"=65535, "Сервис"=FALSE, "Только чтение"=FALSE, "Разработка"=FALSE, "К-во бит"=16, "Шаг"=0, "Обработка"=FALSE, "Макрос"=""}, {"Имя"="ss17", "Группа"="ss", "Наименование"="Счетчик потерь команд управления", "Ед. изм"=0, "Список"="", "Адрес"=2073, "Описание"="Показывает сколько было потеряно команд CAN_POS_COM=0x08 по шине CAN. Счетчик работает только, если выбран один из возможных режимов синхронизации.", "Мин"=0, "Макс"=65535, "Сервис"=FALSE, "Только чтение"=FALSE, "Разработка"=FALSE, "К-во бит"=16, "Шаг"=0, "Обработка"=FALSE, "Макрос"=""}, {"Имя"="ss18", "Группа"="ss", "Наименование"="Счетчик получения неизвестных команд", "Ед. изм"=0, "Список"="", "Адрес"=2074, "Описание"="Показывает сколько было получено неизвестных команд по шине CAN, которые помешали прохождению команд управления. Счетчик работает только, если выбран один из возможных режимов синхронизации.", "Мин"=0, "Макс"=65535, "Сервис"=FALSE, "Только чтение"=FALSE, "Разработка"=FALSE, "К-во бит"=16, "Шаг"=0, "Обработка"=FALSE, "Макрос"=""}, {"Имя"="pd18", "Группа"="pd", "Наименование"="Коэффициент ФНЧ входного сигнала", "Ед. изм"=0, "Список"="", "Адрес"=2589, "Описание"="Параметр настройки ПИД-регулятора", "Мин"=0, "Макс"=1, "Сервис"=TRUE, "Только чтение"=FALSE, "Разработка"=FALSE, "К-во бит"=32, "Шаг"=12, "Обработка"=FALSE, "Макрос"=""}, {"Имя"="pd19", "Группа"="pd", "Наименование"="Коэффициент ФНЧ сигнала обратной связи", "Ед. изм"=0, "Список"="", "Адрес"=2590, "Описание"="Параметр настройки ПИД-регулятора", "Мин"=0, "Макс"=1, "Сервис"=TRUE, "Только чтение"=FALSE, "Разработка"=FALSE, "К-во бит"=32, "Шаг"=12, "Обработка"=FALSE, "Макрос"=""}, {"Имя"="ep7", "Группа"="ep", "Наименование"="Функция контроля зазора", "Ед. изм"=0, "Список"="0:ВЫКЛ\n90:ВКЛ\n\r\n", "Адрес"=2075, "Описание"="Включение данной автоматически запускает внутреннюю программу контроля расстояния между инструментом и обрабатываемым листом.", "Мин"=0, "Макс"=90, "Сервис"=FALSE, "Только чтение"=FALSE, "Разработка"=FALSE, "К-во бит"=16, "Шаг"=1, "Обработка"=FALSE, "Макрос"=""}, {"Имя"="pp11", "Группа"="pp", "Наименование"="Коэффициент микроинтерполяции", "Ед. изм"=0, "Список"="1:1\n2:2\n3:3\n4:4\n5:5\n\r\n", "Адрес"=2076, "Описание"="Коэффициент микроинтерполяции определяет кратность соотношения частот квантования СЧПУ и контура позиции привода. Коэффициент может принимать только значения 1, 2, 3, 4, 5. Если коэффициент равен 1, то частоты СЧПУ и привода равны.", "Мин"=1, "Макс"=5, "Сервис"=TRUE, "Только чтение"=FALSE, "Разработка"=FALSE, "К-во бит"=32, "Шаг"=10, "Обработка"=FALSE, "Макрос"=""}, {"Имя"="ip19", "Группа"="ip", "Наименование"="Данные CAN собщения 0", "Ед. изм"=0, "Список"="", "Адрес"=2077, "Описание"="4 младших байта последнего полученного CAN собщения", "Мин"=-2147483637, "Макс"=2147483646, "Сервис"=FALSE, "Только чтение"=FALSE, "Разработка"=FALSE, "К-во бит"=32, "Шаг"=0, "Обработка"=FALSE, "Макрос"=""}, {"Имя"="ip20", "Группа"="ip", "Наименование"="Данные CAN собщения 1", "Ед. изм"=0, "Список"="", "Адрес"=2078, "Описание"="4 старших байта последнего полученного CAN собщения", "Мин"=-2147483637, "Макс"=2147483646, "Сервис"=FALSE, "Только чтение"=FALSE, "Разработка"=FALSE, "К-во бит"=32, "Шаг"=0, "Обработка"=FALSE, "Макрос"=""}, {"Имя"="dd31", "Группа"="dd", "Наименование"="Смещение фазы ослабления поля", "Ед. изм"=0, "Список"="", "Адрес"=1065, "Описание"="", "Мин"=0, "Макс"=0, "Сервис"=FALSE, "Только чтение"=TRUE, "Разработка"=FALSE, "К-во бит"=16, "Шаг"=0, "Обработка"=FALSE, "Макрос"=""}, {"Имя"="vp25", "Группа"="vp", "Наименование"="Коэффициент ФНЧ входного сигнала", "Ед. изм"=0, "Список"="", "Адрес"=2079, "Описание"="Коэффициент ФНЧ входного сигнала контура скорости", "Мин"=0, "Макс"=1, "Сервис"=TRUE, "Только чтение"=FALSE, "Разработка"=FALSE, "К-во бит"=32, "Шаг"=12, "Обработка"=FALSE, "Макрос"=""}, {"Имя"="vp26", "Группа"="vp", "Наименование"="Коэффициент ФНЧ сигнала обратной связи", "Ед. изм"=0, "Список"="", "Адрес"=2080, "Описание"="Коэффициент ФНЧ сигнала обратной связи контура скорости", "Мин"=0, "Макс"=1, "Сервис"=TRUE, "Только чтение"=FALSE, "Разработка"=FALSE, "К-во бит"=32, "Шаг"=12, "Обработка"=FALSE, "Макрос"=""}, {"Имя"="up17", "Группа"="up", "Наименование"="Переменная общего назначения 8", "Ед. изм"=0, "Список"="", "Адрес"=1809, "Описание"="Может использоваться для общих целей. ВНИМАНИЕ! Данная переменная не записывается в энергонезависимую память.", "Мин"=-2147483647, "Макс"=2147483647, "Сервис"=FALSE, "Только чтение"=FALSE, "Разработка"=FALSE, "К-во бит"=32, "Шаг"=0, "Обработка"=FALSE, "Макрос"=""}, {"Имя"="up18", "Группа"="up", "Наименование"="Переменная общего назначения 9", "Ед. изм"=0, "Список"="", "Адрес"=1810, "Описание"="Может использоваться для общих целей. ВНИМАНИЕ! Данная переменная не записывается в энергонезависимую память.", "Мин"=-2147483647, "Макс"=2147483647, "Сервис"=FALSE, "Только чтение"=FALSE, "Разработка"=FALSE, "К-во бит"=32, "Шаг"=0, "Обработка"=FALSE, "Макрос"=""}, {"Имя"="up19", "Группа"="up", "Наименование"="Переменная общего назначения 10", "Ед. изм"=0, "Список"="", "Адрес"=1811, "Описание"="", "Мин"=-2147483647, "Макс"=2147483647, "Сервис"=FALSE, "Только чтение"=FALSE, "Разработка"=FALSE, "К-во бит"=32, "Шаг"=0, "Обработка"=FALSE, "Макрос"=""}, {"Имя"="up20", "Группа"="up", "Наименование"="Переменная общего назначения 11", "Ед. изм"=0, "Список"="", "Адрес"=1812, "Описание"="", "Мин"=-2147483647, "Макс"=2147483647, "Сервис"=FALSE, "Только чтение"=FALSE, "Разработка"=FALSE, "К-во бит"=32, "Шаг"=0, "Обработка"=FALSE, "Макрос"=""}, {"Имя"="up21", "Группа"="up", "Наименование"="Переменная общего назначения 12", "Ед. изм"=0, "Список"="", "Адрес"=1813, "Описание"="Может использоваться для общих целей. ВНИМАНИЕ! Данная переменная не записывается в энергонезависимую память.", "Мин"=-2147483647, "Макс"=2147483647, "Сервис"=FALSE, "Только чтение"=FALSE, "Разработка"=FALSE, "К-во бит"=32, "Шаг"=0, "Обработка"=FALSE, "Макрос"=""}, {"Имя"="up22", "Группа"="up", "Наименование"="Переменная общего назначения 13", "Ед. изм"=0, "Список"="", "Адрес"=1814, "Описание"="Может использоваться для общих целей. ВНИМАНИЕ! Данная переменная не записывается в энергонезависимую память.", "Мин"=-2147483647, "Макс"=2147483647, "Сервис"=FALSE, "Только чтение"=FALSE, "Разработка"=FALSE, "К-во бит"=32, "Шаг"=0, "Обработка"=FALSE, "Макрос"=""}, {"Имя"="up23", "Группа"="up", "Наименование"="Переменная общего назначения  14", "Ед. изм"=0, "Список"="", "Адрес"=1815, "Описание"="Может использоваться для общих целей. ВНИМАНИЕ! Данная переменная не записывается в энергонезависимую память.", "Мин"=-2147483647, "Макс"=2147483647, "Сервис"=FALSE, "Только чтение"=FALSE, "Разработка"=FALSE, "К-во бит"=32, "Шаг"=0, "Обработка"=FALSE, "Макрос"=""}, {"Имя"="up24", "Группа"="up", "Наименование"="Переменная общего назначения 15", "Ед. изм"=0, "Список"="", "Адрес"=1816, "Описание"="Может использоваться для общих целей. ВНИМАНИЕ! Данная переменная не записывается в энергонезависимую память.", "Мин"=-2147483647, "Макс"=2147483647, "Сервис"=FALSE, "Только чтение"=FALSE, "Разработка"=FALSE, "К-во бит"=32, "Шаг"=0, "Обработка"=FALSE, "Макрос"=""}, {"Имя"="dd32", "Группа"="dd", "Наименование"="Задержка синхронизации", "Ед. изм"=14, "Список"="", "Адрес"=1066, "Описание"="Время между приемом команды упарвления и команды синхронизации. Параметр действителен только для приоводов с интерфейсом упарвления EtherCAT и при активизации управления от СЧПУ.", "Мин"=0, "Макс"=0, "Сервис"=FALSE, "Только чтение"=TRUE, "Разработка"=FALSE, "К-во бит"=32, "Шаг"=0, "Обработка"=FALSE, "Макрос"=""}, {"Имя"="cp11", "Группа"="cp", "Наименование"="Коэффициент ФНЧ входного сигнала", "Ед. изм"=0, "Список"="", "Адрес"=2081, "Описание"="Коэффициент ФНЧ входного сигнала контура тока.", "Мин"=0, "Макс"=1, "Сервис"=TRUE, "Только чтение"=FALSE, "Разработка"=FALSE, "К-во бит"=32, "Шаг"=12, "Обработка"=FALSE, "Макрос"=""}, {"Имя"="cp12", "Группа"="cp", "Наименование"="Коэффициент ФНЧ сигнала ОС", "Ед. изм"=0, "Список"="", "Адрес"=2082, "Описание"="Коэффициент ФНЧ сигнала обратной связи контура тока.", "Мин"=0, "Макс"=1, "Сервис"=TRUE, "Только чтение"=FALSE, "Разработка"=FALSE, "К-во бит"=32, "Шаг"=12, "Обработка"=FALSE, "Макрос"=""}, {"Имя"="st11", "Группа"="st", "Наименование"="Разрешение на полюс двигателя", "Ед. изм"=1, "Список"="", "Адрес"=2083, "Описание"="Формуля для расчета:", "Мин"=1000, "Макс"=2098176, "Сервис"=FALSE, "Только чтение"=FALSE, "Разработка"=FALSE, "К-во бит"=32, "Шаг"=0, "Обработка"=FALSE, "Макрос"=""}, {"Имя"="st12", "Группа"="st", "Наименование"="Коэффициент деления энкодера", "Ед. изм"=0, "Список"="", "Адрес"=2084, "Описание"="Уменьшает разрешение датчика позиции (энкодера) в 2 или 4 раза. Если st12=1, то разрешение энкодера не уменьшается и соответствует физическому разрешению, выдаваемому самим датчиком.", "Мин"=1, "Макс"=4, "Сервис"=FALSE, "Только чтение"=FALSE, "Разработка"=FALSE, "К-во бит"=16, "Шаг"=0, "Обработка"=FALSE, "Макрос"=""}, {"Имя"="st13", "Группа"="st", "Наименование"="Инвертированные сигналы UVW", "Ед. изм"=0, "Список"="0:Нет\n21930:Да\n\r\n", "Адрес"=2085, "Описание"="UVW треки должны следовать в следующем порядке: 2, 3, 1, 5, 4, 6. Для таких датчиков st13=Нет. В некоторых датчиках сигналы идут с инверсией, в этом случае последовательность: 2, 6, 4, 5, 1, 3. Для таких датчиков st13=Да.", "Мин"=-2147483647, "Макс"=2147483647, "Сервис"=FALSE, "Только чтение"=FALSE, "Разработка"=FALSE, "К-во бит"=32, "Шаг"=0, "Обработка"=FALSE, "Макрос"=""}, {"Имя"="dd33", "Группа"="dd", "Наименование"="Кол-во импульсов на сектор UVW сигнала", "Ед. изм"=6, "Список"="", "Адрес"=1067, "Описание"="Кол-во импульсов датчика позиции, приходящееся на текущий сектор UVW сигнала.", "Мин"=-2147483647, "Макс"=2147483647, "Сервис"=FALSE, "Только чтение"=TRUE, "Разработка"=FALSE, "К-во бит"=32, "Шаг"=0, "Обработка"=FALSE, "Макрос"=""}, {"Имя"="dd34", "Группа"="dd", "Наименование"="Ток в роторной системе координат", "Ед. изм"=1, "Список"="", "Адрес"=1068, "Описание"="Ток, пересчитанный в роторную систему координат. Данный сигнал является обратной связью на задание ddd2", "Мин"=-2147483647, "Макс"=2147483647, "Сервис"=TRUE, "Только чтение"=TRUE, "Разработка"=FALSE, "К-во бит"=32, "Шаг"=12, "Обработка"=FALSE, "Макрос"=""}, {"Имя"="st14", "Группа"="st", "Наименование"="Автоматический поиск фазы", "Ед. изм"=0, "Список"="0:Фаза не найдена\n170:Запрос поиска фазы\n171:Ожидание завершения поиска фазы\n172:Ожидаем вращения в +\n173:Ожидаем вращения в -\n174:Ошибка поиска\n175:Поиск выполнен успешно\n\r\n", "Адрес"=2086, "Описание"="Параметр используется для отображения текущего состояния поиска фазы в автоматическом режиме. Поиск фазы позволяет настроить сервоусилитель на конкретный экземпляр двигателя.", "Мин"=0, "Макс"=175, "Сервис"=FALSE, "Только чтение"=TRUE, "Разработка"=FALSE, "К-во бит"=16, "Шаг"=0, "Обработка"=FALSE, "Макрос"=""}] {"Ед. изм" items=["", "дискрет", "об/(сек^2)", "сек", "об/мин", "А", "имп.", "град.", "В", "мксек", "Банк", "мсек", "кГц", "А2сек", "nсек"]; "Адрес" format="%04x"}
  out "Ед. изм":u16(ring) items=["", "дискрет", "об/(сек^2)", "сек", "об/мин", "А", "имп.", "град.", "В", "мксек", "Банк", "мсек", "кГц", "А2сек", "nсек"]
  in  "text":string="//-------------------------------------------------------------\n// СВОЙСТВА МОДУЛЯ\n//-------------------------------------------------------------\nUnit\n\nUnitName    =Имя конфигурации не указано\nUnitVersion =не указано\n\n//-------------------------------------------------------------\n// ДЕРЕВО ПАРАМЕТРОВ\n//-------------------------------------------------------------\nInterface\n\n0,node: Фиксированные параметры\n1,node: Статические параметры\n2,cp: Контур тока\n2,vp: Контур скорости\n2,pp: Контур положения\n2,st: Общие\n2,ip: Интерфейс\n2,ep: Сервисные параметры\n2,io: Порты ввода-вывода\n2,pd: Технологический ПИД регулятор\n1,ct: Параметры управления\n1,dd: Динамические параметры\n1,ss: Системные параметры\n1,tp: Параметры тестирования\n0,node: Пользовательские параметры\n1,up: Пользовательские переменные\n\n//-------------------------------------------------------------\n// ОПИСАНИЕ ПАРАМЕТРОВ\n//-------------------------------------------------------------\nDescriptions\n\n---\nNAME     =cp1\nGROUP    =cp\nCAPTION  =Пропорциональный коэффициент контура тока\nUNITS    =\nLIST     =\nADDRESS  =0x0000\nDESCRIP  =Параметр настройки ПИ-регулятора контура тока\nMINMAX   =0;100\nSERVICE  =1\nREADONLY =0\nDEVELOP  =0\nBITS     =32\nSTEP     =12\nMACROS   =0\n---\nNAME     =cp2\nGROUP    =cp\nCAPTION  =Интегральный коэффициент контура тока\nUNITS    =\nLIST     =\nADDRESS  =0x0002\nDESCRIP  =Параметр настройки ПИ-регулятора контура тока\nMINMAX   =0;200\nSERVICE  =1\nREADONLY =0\nDEVELOP  =0\nBITS     =32\nSTEP     =12\nMACROS   =0\n---\nNAME     =cp3\nGROUP    =cp\nCAPTION  =Максимальный ток\nUNITS    =дискрет\nLIST     =\nADDRESS  =0x0004\nDESCRIP  =Определять предельную величину тока допустимую для двигателя.\nMINMAX   =0;1500\nSERVICE  =0\nREADONLY =0\nDEVELOP  =0\nBITS     =16\nSTEP     =0.25\nMACROS   =1\n---\nNAME     =cp4\nGROUP    =cp\nCAPTION  =Максимальная скваженность ШИМ\nUNITS    =дискрет\nLIST     =\nADDRESS  =0x0005\nDESCRIP  =3070 дискрет соответствует 100% заполнения\nMINMAX   =0;6150\nSERVICE  =0\nREADONLY =0\nDEVELOP  =0\nBITS     =16\nSTEP     =0.25\nMACROS   =1\n---\nNAME     =vp1\nGROUP    =vp\nCAPTION  =Пропорциональный коэффициент контура скорости\nUNITS    =\nLIST     =\nADDRESS  =0x0006\nDESCRIP  =Параметр настройки ПИ-регулятора контура скорости\nMINMAX   =0;60000\nSERVICE  =1\nREADONLY =0\nDEVELOP  =0\nBITS     =32\nSTEP     =12\nMACROS   =0\n---\nNAME     =vp2\nGROUP    =vp\nCAPTION  =Интегральный коэффициент контура скорости\nUNITS    =\nLIST     =\nADDRESS  =0x0007\nDESCRIP  =Параметр настройки ПИ-регулятора контура скорости\nMINMAX   =0;60000\nSERVICE  =1\nREADONLY =0\nDEVELOP  =0\nBITS     =32\nSTEP     =12\nMACROS   =0\n---\nNAME     =vp16\nGROUP    =vp\nCAPTION  =Дифференциальный коэффициент контура скорости\nUNITS    =\nLIST     =\nADDRESS  =0x0050\nDESCRIP  =Параметр настройки ПИ-регулятора контура скорости\nMINMAX   =0;60000\nSERVICE  =1\nREADONLY =0\nDEVELOP  =0\nBITS     =32\nSTEP     =12\nMACROS   =0\n---\nNAME     =vp3\nGROUP    =vp\nCAPTION  =Коэффициент обратной связи по скорости\nUNITS    =\nLIST     =\nADDRESS  =0x0008\nDESCRIP  =Определяет масштаб датчика скорости\nMINMAX   =-1;1\nSERVICE  =1\nREADONLY =0\nDEVELOP  =0\nBITS     =32\nSTEP     =12\nMACROS   =0\n---\nNAME     =vp4\nGROUP    =vp\nCAPTION  =Частота дискретизации контура скорости\nUNITS    =\nLIST     =100:100; 200:200; 500:500; 1000:1000; 2000:2000; 3000:3000; 4000:4000; 5000:5000;\nADDRESS  =0x0009\nDESCRIP  =Определяет частоту обсчета контура скорости\nMINMAX   =100;5000\nSERVICE  =0\nREADONLY =0\nDEVELOP  =0\nBITS     =16\nSTEP     =\nMACROS   =0\n---\nNAME     =vp5\nGROUP    =vp\nCAPTION  =Ускорение\nUNITS    =об/(сек^2)\nLIST     =\nADDRESS  =0x000A\nDESCRIP  =Определяет динамику контура скорости\nMINMAX   =1;2000000\nSERVICE  =1\nREADONLY =0\nDEVELOP  =0\nBITS     =32\nSTEP     =10\nMACROS   =0\n---\nNAME     =pp1\nGROUP    =pp\nCAPTION  =Пропорциональный коэффициент контура положения\nUNITS    =\nLIST     =\nADDRESS  =0x000B\nDESCRIP  =Параметр настройки ПИ-регулятора контура позиционирования\nMINMAX   =0;10000\nSERVICE  =1\nREADONLY =0\nDEVELOP  =0\nBITS     =32\nSTEP     =4\nMACROS   =0\n---\nNAME     =pp2\nGROUP    =pp\nCAPTION  =Интегральный коэффициент контура положения\nUNITS    =\nLIST     =\nADDRESS  =0x000C\nDESCRIP  =Параметр настройки ПИ-регулятора контура позиционирования\nMINMAX   =0;30000\nSERVICE  =1\nREADONLY =0\nDEVELOP  =0\nBITS     =32\nSTEP     =4\nMACROS   =0\n---\nNAME     =pp3\nGROUP    =pp\nCAPTION  =Частота дискретизации контура положения\nUNITS    =\nLIST     =25:25;50:50;100:100;200:200;500:500;1000:1000;2000:2000;3000:3000;4000:4000;5000:5000;\nADDRESS  =0x000D\nDESCRIP  =Определяет частоту обсчета контура позиции.\nMINMAX   =25;5000\nSERVICE  =0\nREADONLY =0\nDEVELOP  =0\nBITS     =16\nSTEP     =\nMACROS   =0\n---\nNAME     =vp6\nGROUP    =vp\nCAPTION  =Максимальное время выхода на номинальный режим\nUNITS    =сек\nLIST     =0:Не ограничено;1:1;2:2;3:3;4:4;5:5;6:6;7:7;8:8;9:9;10:10;11:11;12:12;13:13;14:14;15:15;16:16;17:17;18:18;19:19;20:20;21:21;22:22;23:23;24:24;25:25;26:26;27:27;28:28;29:29;30:30\nADDRESS  =0x000E\nDESCRIP  =Время, по истечению которого привод переходит в состояние останова, если не достигнута заданная скорость\nMINMAX   =0;30\nSERVICE  =0\nREADONLY =0\nDEVELOP  =0\nBITS     =16\nSTEP     =1\nMACROS   =1\n---\nNAME     =cp5\nGROUP    =cp\nCAPTION  =Состояние контура тока\nUNITS    =\nLIST     =0:Разомкнут;2:Замкнут;4:Прямое управление токами в обмотках;5:Адаптивное упрваление;6:Прямое раздельное управление токами в обмотках;\nADDRESS  =0x0010\nDESCRIP  =Обеспечивает замкнутое или разомкнутое регулирование контура тока. В стандартном режиме использования контур должен быть замкнут.\nMINMAX   =0;6\nSERVICE  =0\nREADONLY =0\nDEVELOP  =0\nBITS     =16\nSTEP     =\nMACROS   =0\n---\nNAME     =vp7\nGROUP    =vp\nCAPTION  =Состояние контура скорости\nUNITS    =\nLIST     =0:Разомкнут;2:Замкнут;\nADDRESS  =0x0011\nDESCRIP  =Обеспечивает замкнутое или разомкнутое регулирование контура скорости. Контур должен быть замкнут в режиме управления скоростью привода и в режиме управления позицией.\nMINMAX   =0;2\nSERVICE  =0\nREADONLY =0\nDEVELOP  =0\nBITS     =16\nSTEP     =\nMACROS   =0\n---\nNAME     =pp5\nGROUP    =pp\nCAPTION  =Состояние контура положения\nUNITS    =\nLIST     =0:Разомкнут;2:Замкнут;\nADDRESS  =0x0012\nDESCRIP  =Обеспечивает замкнутое или разомкнутое регулирование контура позиции\nMINMAX   =0;2\nSERVICE  =0\nREADONLY =0\nDEVELOP  =0\nBITS     =16\nSTEP     =\nMACROS   =0\n---\nNAME     =vp8\nGROUP    =vp\nCAPTION  =Максимальная скорость вращения\nUNITS    =об/мин\nLIST     =\nADDRESS  =0x0014\nDESCRIP  =Ограничение максимальной скорости вращения привода.\nMINMAX   =0;8000\nSERVICE  =1\nREADONLY =0\nDEVELOP  =0\nBITS     =32\nSTEP     =12\nMACROS   =0\n---\nNAME     =vp9\nGROUP    =vp\nCAPTION  =Динамический режим\nUNITS    =\nLIST     =0:Режим плавного разгона/торможения;2:Режим с максимальной динамикой;3:Режим G декодирования;4:S кривая;\nADDRESS  =0x000F\nDESCRIP  =Включает или отключает внутренний интерполятор. В режиме управления приводов от внешнего контроллера, например, от ЧПУ, привод должен находиться в режиме с максимальной динамикой. Режим G декодирования позволяет реализовать контурное управление непосредственно группой приводов без использования внешнего контроллера.\nMINMAX   =0;4\nSERVICE  =0\nREADONLY =0\nDEVELOP  =0\nBITS     =16\nSTEP     =\nMACROS   =0\n---\nNAME     =ss1\nGROUP    =ss\nCAPTION  =Тестовый параметр\nUNITS    =\nLIST     =\nADDRESS  =0x0013\nDESCRIP  =\nMINMAX   =-65535;65535\nSERVICE  =0\nREADONLY =0\nDEVELOP  =1\nBITS     =16\nSTEP     =\nMACROS   =0\n---\nNAME     =ct1\nGROUP    =ct\nCAPTION  =Задание тока\nUNITS    =А\nLIST     =\nADDRESS  =0x0200\nDESCRIP  =Сигнал управления при разомкнутом контуре скорости и положения\nMINMAX   =-3500;3500\nSERVICE  =0\nREADONLY =0\nDEVELOP  =0\nBITS     =16\nSTEP     =0.05\nMACROS   =1\n---\nNAME     =ct2\nGROUP    =ct\nCAPTION  =Задание скорости\nUNITS    =об/мин\nLIST     =\nADDRESS  =0x0202\nDESCRIP  =Сигнал управления при разомкнутом контуре положения\nMINMAX   =-12000;12000\nSERVICE  =1\nREADONLY =0\nDEVELOP  =0\nBITS     =32\nSTEP     =12\nMACROS   =0\n---\nNAME     =ct3\nGROUP    =ct\nCAPTION  =Задание положения\nUNITS    =имп.\nLIST     =\nADDRESS  =0x0204\nDESCRIP  =Сигнал управления при замкнутом контуре положения\nMINMAX   =-2147483647;2147483647\nSERVICE  =0\nREADONLY =0\nDEVELOP  =0\nBITS     =32\nSTEP     =\nMACROS   =0\n---\nNAME     =dd1\nGROUP    =dd\nCAPTION  =Ток в обмотке 1\nUNITS    =А\nLIST     =\nADDRESS  =0x0400\nDESCRIP  =Показывает ток, протекающий в обмотке двигателя\nMINMAX   =-5;5\nSERVICE  =0\nREADONLY =1\nDEVELOP  =0\nBITS     =16\nSTEP     =0.05\nMACROS   =1\n---\nNAME     =dd6\nGROUP    =dd\nCAPTION  =Заданный ток в обмотке 1\nUNITS    =А\nLIST     =\nADDRESS  =0x040A\nDESCRIP  =\nMINMAX   =-2047;2047\nSERVICE  =0\nREADONLY =0\nDEVELOP  =0\nBITS     =16\nSTEP     =\nMACROS   =1\n---\nNAME     =dd3\nGROUP    =dd\nCAPTION  =Ток в обмотке 2\nUNITS    =А\nLIST     =\nADDRESS  =0x0405\nDESCRIP  =Индицирует ток, протекающий в обмотке двигателя\nMINMAX   =-5;5\nSERVICE  =0\nREADONLY =1\nDEVELOP  =0\nBITS     =16\nSTEP     =0.05\nMACROS   =1\n---\nNAME     =dd9\nGROUP    =dd\nCAPTION  =Заданный ток в обмотке 2\nUNITS    =А\nLIST     =\nADDRESS  =0x040D\nDESCRIP  =\nMINMAX   =-2047;2047\nSERVICE  =0\nREADONLY =0\nDEVELOP  =0\nBITS     =16\nSTEP     =\nMACROS   =1\n---\nNAME     =dd2\nGROUP    =dd\nCAPTION  =Заданный ток в роторной системе координат\nUNITS    =А\nLIST     =\nADDRESS  =0x0402\nDESCRIP  =Индицирует ток, который задан контуром скорости\nMINMAX   =-5;5\nSERVICE  =0\nREADONLY =1\nDEVELOP  =0\nBITS     =16\nSTEP     =0.05\nMACROS   =1\n---\nNAME     =dd4\nGROUP    =dd\nCAPTION  =Текущая скорость вращения\nUNITS    =об/мин\nLIST     =\nADDRESS  =0x0408\nDESCRIP  =\nMINMAX   =-5000;5000\nSERVICE  =0\nREADONLY =1\nDEVELOP  =0\nBITS     =8\nSTEP     =12\nMACROS   =0\n---\nNAME     =dd5\nGROUP    =dd\nCAPTION  =Заданная скорость вращения\nUNITS    =об/мин\nLIST     =\nADDRESS  =0x0409\nDESCRIP  =\nMINMAX   =-5000;5000\nSERVICE  =0\nREADONLY =1\nDEVELOP  =0\nBITS     =16\nSTEP     =12\nMACROS   =0\n---\nNAME     =dd21\nGROUP    =dd\nCAPTION  =Ошибка контура скорости\nUNITS    =об/мин\nLIST     =\nADDRESS  =0x0419\nDESCRIP  =\nMINMAX   =-65535;65535\nSERVICE  =0\nREADONLY =1\nDEVELOP  =0\nBITS     =16\nSTEP     =1\nMACROS   =0\n---\nNAME     =dd7\nGROUP    =dd\nCAPTION  =Заданная позиция\nUNITS    =имп.\nLIST     =\nADDRESS  =0x040B\nDESCRIP  =\nMINMAX   =-2147483647;2147483647\nSERVICE  =0\nREADONLY =1\nDEVELOP  =0\nBITS     =32\nSTEP     =\nMACROS   =0\n---\nNAME     =dd8\nGROUP    =dd\nCAPTION  =Текущая позиция\nUNITS    =имп.\nLIST     =\nADDRESS  =0x040C\nDESCRIP  =\nMINMAX   =-2147483647;2147483647\nSERVICE  =0\nREADONLY =1\nDEVELOP  =0\nBITS     =32\nSTEP     =\nMACROS   =0\n---\nNAME     =dd20\nGROUP    =dd\nCAPTION  =Ошибка контура позиции\nUNITS    =имп.\nLIST     =\nADDRESS  =0x0418\nDESCRIP  =\nMINMAX   =-2147483647;2147483647\nSERVICE  =1\nREADONLY =1\nDEVELOP  =0\nBITS     =32\nSTEP     =10\nMACROS   =0\n---\nNAME     =dd10\nGROUP    =dd\nCAPTION  =Температура внутри корпуса\nUNITS    =град.\nLIST     =\nADDRESS  =0x040E\nDESCRIP  =\nMINMAX   =-40;120\nSERVICE  =0\nREADONLY =1\nDEVELOP  =0\nBITS     =16\nSTEP     =\nMACROS   =1\n---\nNAME     =dd19\nGROUP    =dd\nCAPTION  =Текущее цифровое напряжение\nUNITS    =В\nLIST     =\nADDRESS  =0x0417\nDESCRIP  =\nMINMAX   =0;23\nSERVICE  =0\nREADONLY =1\nDEVELOP  =0\nBITS     =16\nSTEP     =\nMACROS   =1\n---\nNAME     =dd12\nGROUP    =dd\nCAPTION  =Текущее напряжение питания\nUNITS    =В\nLIST     =\nADDRESS  =0x0410\nDESCRIP  =\nMINMAX   =0;120\nSERVICE  =0\nREADONLY =1\nDEVELOP  =0\nBITS     =16\nSTEP     =\nMACROS   =1\n---\nNAME     =dd11\nGROUP    =dd\nCAPTION  =Статус контроллера\nUNITS    =\nLIST     =0:Исправен;1:Останов по команде;2:Останов - высокое противодействующее усилие;3:Останов - короткое замыкание;4:Выход из температурного диапазона;5:Повышенное силовое напряжение;6:Низкое силовое напряжение;7:Повышенное цифровое напряжение;8:Низкое цифровое напряжение;9:Cиловое напряжение превышает напряжение, установл. пользователем;10:Останов - превышение допустимой перегрузки;11:Останов - сработала защита IGBT модуля;12:Останов - Ошибка поиска фазы по UVW трекам;13:Останов - ошибка в настройках энкодера;14: Останов - сбой в работе энкодера;15: Останов - Ошибка фазировки двигателя;\nADDRESS  =0x040F\nDESCRIP  =Привод в состоянии отработать задание только, если его статус \"Исправен\".\nMINMAX   =0;15\nSERVICE  =0\nREADONLY =0\nDEVELOP  =0\nBITS     =16\nSTEP     =\nMACROS   =0\n---\nNAME     =st1\nGROUP    =st\nCAPTION  =Разрешение\nUNITS    =имп.\nLIST     =\nADDRESS  =0x0015\nDESCRIP  =Разрешение датчика положения/скорости\nMINMAX   =0;2147483647\nSERVICE  =0\nREADONLY =0\nDEVELOP  =0\nBITS     =32\nSTEP     =\nMACROS   =0\n---\nNAME     =tp1\nGROUP    =tp\nCAPTION  =Режим осциллографа\nUNITS    =\nLIST     =0:Непрерывный режим;1:Ступенька;2:Синус;3:Приращение скорости;4:Синусоидальное изменение скорости;5:Треугольное изменение позиции;6:Измерение без задания;7:Измерение без задания до принудительного останова;8:Приращение момента;\nADDRESS  =0x0500\nDESCRIP  =Режим сканирования динамических параметров (отображение выбранных параметров в процессе работы привода).\nMINMAX   =0;8\nSERVICE  =0\nREADONLY =0\nDEVELOP  =0\nBITS     =16\nSTEP     =\nMACROS   =0\n---\nNAME     =tp3\nGROUP    =tp\nCAPTION  =Амплитуда задания положения\nUNITS    =\nLIST     =\nADDRESS  =0x0504\nDESCRIP  =Определяет величину приращения позиции в режиме осциллографа 1.\nMINMAX   =-2147483647;2147483647\nSERVICE  =0\nREADONLY =0\nDEVELOP  =0\nBITS     =32\nSTEP     =\nMACROS   =0\n---\nNAME     =ip0\nGROUP    =ip\nCAPTION  =Источник опорного сигнала\nUNITS    =\nLIST     =0:Интерфейс USB;2:Интерфейс StepDir;4:Аналоговый интерфейс;5:Интерфейс CAN;6:Квадратурный интерфейс\nADDRESS  =0x0017\nDESCRIP  =Определяет интерфейс, по которому осуществляется ввод задания для привода.\nMINMAX   =0;6\nSERVICE  =0\nREADONLY =0\nDEVELOP  =0\nBITS     =16\nSTEP     =\nMACROS   =0\n---\nNAME     =st2\nGROUP    =st\nCAPTION  =Версия ПО драйвера\nUNITS    =\nLIST     =\nADDRESS  =0x0016\nDESCRIP  =Текущая версия программного обеспечения привода.\nMINMAX   =0;2147483647\nSERVICE  =1\nREADONLY =0\nDEVELOP  =0\nBITS     =32\nSTEP     =12\nMACROS   =0\n---\nNAME     =ip1\nGROUP    =ip\nCAPTION  =Коэффициент веса одной дискреты\nUNITS    =\nLIST     =\nADDRESS  =0x0018\nDESCRIP  =Определяет количество импульсов датчика, на которые необходимо повернуть вал двигателя, при получении одной дискреты по интерфейсу Step/Dir, т.е. масштаб одного импульса\nMINMAX   =-4000;4000\nSERVICE  =1\nREADONLY =0\nDEVELOP  =0\nBITS     =32\nSTEP     =10\nMACROS   =0\n---\nNAME     =tp2\nGROUP    =tp\nCAPTION  =Период опроса параметров\nUNITS    =мксек\nLIST     =\nADDRESS  =0x0502\nDESCRIP  =Определяет интервал времени между запоминанием данных в массив в режимах 1-7.\nMINMAX   =25;25000\nSERVICE  =0\nREADONLY =0\nDEVELOP  =0\nBITS     =16\nSTEP     =25\nMACROS   =0\n---\nNAME     =tp5\nGROUP    =tp\nCAPTION  =Период задающего воздействия\nUNITS    =мксек\nLIST     =\nADDRESS  =0x0505\nDESCRIP  =Данный параметр определяет задержку введения задающего воздействия от начала сбора информации в режиме осциллографа 1 и 3.\nMINMAX   =25;800000\nSERVICE  =0\nREADONLY =0\nDEVELOP  =0\nBITS     =16\nSTEP     =25\nMACROS   =1\n---\nNAME     =tp6\nGROUP    =tp\nCAPTION  =Амплитуда задания скорости\nUNITS    =об/мин\nLIST     =\nADDRESS  =0x0506\nDESCRIP  =Определяет величину приращения скорости в режиме осциллографа 3.\nMINMAX   =-14000;14000\nSERVICE  =0\nREADONLY =0\nDEVELOP  =0\nBITS     =16\nSTEP     =\nMACROS   =0\n---\nNAME     =ip2\nGROUP    =ip\nCAPTION  =Текущий банк программы интерпретатора\nUNITS    =Банк\nLIST     =0:0;1:1;2:2;3:3;4:4;5:5;6:6;7:7;255:Программа не выбрана;\nADDRESS  =0x001A\nDESCRIP  =Банк, из которой загружена программа на выполнение.\nMINMAX   =0;255\nSERVICE  =0\nREADONLY =0\nDEVELOP  =0\nBITS     =16\nSTEP     =1\nMACROS   =0\n---\nNAME     =ip3\nGROUP    =ip\nCAPTION  =Текущий банк чт/записи программ интерпретатора\nUNITS    =Банк\nLIST     =0:0;1:1;2:2;3:3;4:4;5:5;6:6;7:7;255:Программа не выбрана;\nADDRESS  =0x001B\nDESCRIP  =\nMINMAX   =0;255\nSERVICE  =0\nREADONLY =1\nDEVELOP  =1\nBITS     =16\nSTEP     =1\nMACROS   =0\n---\nNAME     =ip4\nGROUP    =ip\nCAPTION  =Режим работы интерпретатора\nUNITS    =\nLIST     =0:Режим выполнения программы;1:Режим отладки;\nADDRESS  =0x001C\nDESCRIP  =Режим работы интерпретатора\nMINMAX   =0;1\nSERVICE  =0\nREADONLY =0\nDEVELOP  =0\nBITS     =16\nSTEP     =1\nMACROS   =0\n---\nNAME     =st3\nGROUP    =st\nCAPTION  =Уникальный идентификатор устройства\nUNITS    =\nLIST     =\nADDRESS  =0x001E\nDESCRIP  =\nMINMAX   =0;2147483647\nSERVICE  =0\nREADONLY =0\nDEVELOP  =0\nBITS     =32\nSTEP     =\nMACROS   =0\n---\nNAME     =ip5\nGROUP    =ip\nCAPTION  =Порт ввода вывода\nUNITS    =\nLIST     =\nADDRESS  =0x0001D\nDESCRIP  =Старший байт содержит содержимое порта вывода, младший - состояние линий ввода.\nMINMAX   =0;65535\nSERVICE  =0\nREADONLY =0\nDEVELOP  =0\nBITS     =16\nSTEP     =\nMACROS   =0\n---\nNAME     =ss2\nGROUP    =ss\nCAPTION  =Количество КЗ\nUNITS    =\nLIST     =\nADDRESS  =0x001F\nDESCRIP  =Количество зафиксированных коротких замыканий\nMINMAX   =0;65535\nSERVICE  =0\nREADONLY =0\nDEVELOP  =0\nBITS     =16\nSTEP     =\nMACROS   =0\n---\nNAME     =ss3\nGROUP    =ss\nCAPTION  =Количество превышений температуры\nUNITS    =\nLIST     =\nADDRESS  =0x0020\nDESCRIP  =Количество зафиксированных превышений температуры\nMINMAX   =0;65535\nSERVICE  =0\nREADONLY =0\nDEVELOP  =0\nBITS     =16\nSTEP     =\nMACROS   =0\n---\nNAME     =ss4\nGROUP    =ss\nCAPTION  =Количество перенапряжений\nUNITS    =\nLIST     =\nADDRESS  =0x0021\nDESCRIP  =Количество зафиксированных перенапряжений\nMINMAX   =0;65535\nSERVICE  =0\nREADONLY =0\nDEVELOP  =0\nBITS     =16\nSTEP     =\nMACROS   =0\n---\nNAME     =ss5\nGROUP    =ss\nCAPTION  =Количество недонапряжений\nUNITS    =\nLIST     =\nADDRESS  =0x0022\nDESCRIP  =Количество зафиксированных случаев пониженного напряжений\nMINMAX   =0;65535\nSERVICE  =0\nREADONLY =0\nDEVELOP  =0\nBITS     =16\nSTEP     =\nMACROS   =0\n---\nNAME     =ss6\nGROUP    =ss\nCAPTION  =Количество перегрузок\nUNITS    =\nLIST     =\nADDRESS  =0x0023\nDESCRIP  =\nMINMAX   =0;65535\nSERVICE  =0\nREADONLY =0\nDEVELOP  =0\nBITS     =16\nSTEP     =\nMACROS   =0\n---\nNAME     =ss7\nGROUP    =ss\nCAPTION  =Количество перепрогарммирований\nUNITS    =\nLIST     =\nADDRESS  =0x0024\nDESCRIP  =\nMINMAX   =0;65535\nSERVICE  =0\nREADONLY =0\nDEVELOP  =0\nBITS     =16\nSTEP     =\nMACROS   =0\n---\nNAME     =ss8\nGROUP    =ss\nCAPTION  =Сообщение 0\nUNITS    =\nLIST     =1:Короткое замыкание;2:Перегрев;3:Повышенное напряжение;4:Пониженное напряжение;5:Перегрузка по току;6:Произведена перезапись контроллера;\nADDRESS  =0x0025\nDESCRIP  =Журнал последних 8 сообщений\nMINMAX   =0;65535\nSERVICE  =0\nREADONLY =0\nDEVELOP  =0\nBITS     =16\nSTEP     =\nMACROS   =0\n---\nNAME     =ss9\nGROUP    =ss\nCAPTION  =Сообщение 1\nUNITS    =\nLIST     =1:Короткое замыкание;2:Перегрев;3:Повышенное напряжение;4:Пониженное напряжение;5:Перегрузка по току;6:Произведена перезапись контроллера;\nADDRESS  =0x0026\nDESCRIP  =Журнал последних 8 сообщений\nMINMAX   =0;65535\nSERVICE  =0\nREADONLY =0\nDEVELOP  =0\nBITS     =16\nSTEP     =\nMACROS   =0\n---\nNAME     =ss10\nGROUP    =ss\nCAPTION  =Сообщение 2\nUNITS    =\nLIST     =1:Короткое замыкание;2:Перегрев;3:Повышенное напряжение;4:Пониженное напряжение;5:Перегрузка по току;6:Произведена перезапись контроллера;\nADDRESS  =0x0027\nDESCRIP  =Журнал последних 8 сообщений\nMINMAX   =0;65535\nSERVICE  =0\nREADONLY =0\nDEVELOP  =0\nBITS     =16\nSTEP     =\nMACROS   =0\n---\nNAME     =ss11\nGROUP    =ss\nCAPTION  =Сообщение 3\nUNITS    =\nLIST     =1:Короткое замыкание;2:Перегрев;3:Повышенное напряжение;4:Пониженное напряжение;5:Перегрузка по току;6:Произведена перезапись контроллера;\nADDRESS  =0x0028\nDESCRIP  =Журнал последних 8 сообщений\nMINMAX   =0;65535\nSERVICE  =0\nREADONLY =0\nDEVELOP  =0\nBITS     =16\nSTEP     =\nMACROS   =0\n---\nNAME     =ss12\nGROUP    =ss\nCAPTION  =Сообщение 4\nUNITS    =\nLIST     =1:Короткое замыкание;2:Перегрев;3:Повышенное напряжение;4:Пониженное напряжение;5:Перегрузка по току;6:Произведена перезапись контроллера;\nADDRESS  =0x0029\nDESCRIP  =Журнал последних 8 сообщений\nMINMAX   =0;65535\nSERVICE  =0\nREADONLY =0\nDEVELOP  =0\nBITS     =16\nSTEP     =\nMACROS   =0\n---\nNAME     =ss13\nGROUP    =ss\nCAPTION  =Сообщение 5\nUNITS    =\nLIST     =1:Короткое замыкание;2:Перегрев;3:Повышенное напряжение;4:Пониженное напряжение;5:Перегрузка по току;6:Произведена перезапись контроллера;\nADDRESS  =0x002A\nDESCRIP  =Журнал последних 8 сообщений\nMINMAX   =0;65535\nSERVICE  =0\nREADONLY =0\nDEVELOP  =0\nBITS     =16\nSTEP     =\nMACROS   =0\n---\nNAME     =ss14\nGROUP    =ss\nCAPTION  =Сообщение 6\nUNITS    =\nLIST     =1:Короткое замыкание;2:Перегрев;3:Повышенное напряжение;4:Пониженное напряжение;5:Перегрузка по току;6:Произведена перезапись контроллера;\nADDRESS  =0x002B\nDESCRIP  =Журнал последних 8 сообщений\nMINMAX   =0;65535\nSERVICE  =0\nREADONLY =0\nDEVELOP  =0\nBITS     =16\nSTEP     =\nMACROS   =0\n---\nNAME     =ss15\nGROUP    =ss\nCAPTION  =Сообщение 7\nUNITS    =\nLIST     =1:Короткое замыкание;2:Перегрев;3:Повышенное напряжение;4:Пониженное напряжение;5:Перегрузка по току;6:Произведена перезапись контроллера;\nADDRESS  =0x002C\nDESCRIP  =Журнал последних 8 сообщений\nMINMAX   =0;65535\nSERVICE  =0\nREADONLY =0\nDEVELOP  =0\nBITS     =16\nSTEP     =\nMACROS   =0\n---\nNAME     =ip6\nGROUP    =ip\nCAPTION  =Смещение диапазона сигнала управления\nUNITS    =\nLIST     =\nADDRESS  =0x0030\nDESCRIP  =Используется для корректировки диапазона регулирования входного сигнала (аналогового или Step\\Dir). Значение 2048 соответствует нулевой скорости при подаче на вход нулевого напряжения.\nMINMAX   =0;4096\nSERVICE  =0\nREADONLY =0\nDEVELOP  =0\nBITS     =16\nSTEP     =\nMACROS   =0\n---\nNAME     =dd13\nGROUP    =dd\nCAPTION  =Тестовый параметр 1\nUNITS    =\nLIST     =\nADDRESS  =0x0411\nDESCRIP  =Пока используется для индикации перехода на меандр вместо синуса. Параметр для разработчика\nMINMAX   =-65535;65535\nSERVICE  =0\nREADONLY =1\nDEVELOP  =1\nBITS     =16\nSTEP     =\nMACROS   =0\n---\nNAME     =dd14\nGROUP    =dd\nCAPTION  =Тестовый параметр 2\nUNITS    =\nLIST     =\nADDRESS  =0x0412\nDESCRIP  =Пока используется для индикации сдвига фазы\nMINMAX   =-65535;65535\nSERVICE  =0\nREADONLY =1\nDEVELOP  =1\nBITS     =16\nSTEP     =\nMACROS   =0\n---\nNAME     =vp10\nGROUP    =vp\nCAPTION  =Начало резонансного диапазона 1\nUNITS    =об/мин\nLIST     =\nADDRESS  =0x0031\nDESCRIP  =Если начало и конец диапазона равны, то диапазон не выбран.\nMINMAX   =0;8000\nSERVICE  =0\nREADONLY =0\nDEVELOP  =0\nBITS     =16\nSTEP     =\nMACROS   =1\n---\nNAME     =vp11\nGROUP    =vp\nCAPTION  =Конец резонансного диапазона 1\nUNITS    =об/мин\nLIST     =\nADDRESS  =0x0032\nDESCRIP  =Если начало и конец диапазона равны, то диапазон не выбран.\nMINMAX   =0;8000\nSERVICE  =0\nREADONLY =0\nDEVELOP  =0\nBITS     =16\nSTEP     =\nMACROS   =1\n---\nNAME     =vp12\nGROUP    =vp\nCAPTION  =Начало резонансного диапазона 2\nUNITS    =об/мин\nLIST     =\nADDRESS  =0x0033\nDESCRIP  =Если начало и конец диапазона равны, то диапазон не выбран.\nMINMAX   =0;8000\nSERVICE  =0\nREADONLY =0\nDEVELOP  =0\nBITS     =16\nSTEP     =\nMACROS   =1\n---\nNAME     =vp13\nGROUP    =vp\nCAPTION  =Конец резонансного диапазона 2\nUNITS    =об/мин\nLIST     =\nADDRESS  =0x0034\nDESCRIP  =Если начало и конец диапазона равны, то диапазон не выбран.\nMINMAX   =0;8000\nSERVICE  =0\nREADONLY =0\nDEVELOP  =0\nBITS     =16\nSTEP     =\nMACROS   =1\n---\nNAME     =ip7\nGROUP    =ip\nCAPTION  =CAN адрес устройства\nUNITS    =\nLIST     =\nADDRESS  =0x0035\nDESCRIP  =Адрес данного устройства в сети CAN\nMINMAX   =0;127\nSERVICE  =0\nREADONLY =0\nDEVELOP  =0\nBITS     =16\nSTEP     =\nMACROS   =0\n---\nNAME     =ip8\nGROUP    =ip\nCAPTION  =CAN адрес удаленного узла\nUNITS    =\nLIST     =\nADDRESS  =0x0036\nDESCRIP  =Адрес удаленного устройства в сети CAN, которое выступает в качестве мастера для данного устройства\nMINMAX   =0;127\nSERVICE  =0\nREADONLY =0\nDEVELOP  =0\nBITS     =16\nSTEP     =\nMACROS   =0\n---\nNAME     =ip9\nGROUP    =ip\nCAPTION  =Режим синхронизации по CAN\nUNITS    =\nLIST     =0:Режим не выбран;1:Режим мастер;2:Режим слейв;3:Режим контурного управления;4:Синхронизация по команде SYNC;\nADDRESS  =0x0037\nDESCRIP  =В режиме мастер привод передает текущую позицию в CAN на адрес удаленного узла.\nMINMAX   =0;4\nSERVICE  =0\nREADONLY =0\nDEVELOP  =0\nBITS     =16\nSTEP     =\nMACROS   =0\n---\nNAME     =ip10\nGROUP    =ip\nCAPTION  =Статус шины CAN\nUNITS    =\nLIST     =0:Норма;1:Неисправности на линии;2:Ошибка передачи синхронизации слейву;3:Ошибка - подтверждение не получено.\nADDRESS  =0x0038\nDESCRIP  =Статус 2 - устанавливается, если мастер не может передать сообщение слейву в течение ip7\nMINMAX   =0;3\nSERVICE  =0\nREADONLY =1\nDEVELOP  =0\nBITS     =16\nSTEP     =\nMACROS   =0\n---\nNAME     =vp14\nGROUP    =vp\nCAPTION  =Номинальная скорость\nUNITS    =об/мин\nLIST     =\nADDRESS  =0x0039\nDESCRIP  =Скорость, начиная с которой выполняется режим ослабления поля.\nMINMAX   =0;5000\nSERVICE  =0\nREADONLY =0\nDEVELOP  =0\nBITS     =16\nSTEP     =\nMACROS   =1\n---\nNAME     =vp15\nGROUP    =vp\nCAPTION  =Авто расчет номинальной скорости\nUNITS    =\nLIST     =1:Да;0:Нет;\nADDRESS  =0x0040\nDESCRIP  =Автоматический расчет номинальной скорости выполняется на основе текущего напряжения питания при включении привода.\nMINMAX   =0;1\nSERVICE  =0\nREADONLY =0\nDEVELOP  =0\nBITS     =16\nSTEP     =\nMACROS   =0\n---\nNAME     =si1\nGROUP    =ss\nCAPTION  =Смещение датчика тока 1\nUNITS    =\nLIST     =\nADDRESS  =0x0600\nDESCRIP  =Формула расчета I=cur1-511-si1\nMINMAX   =0;4096\nSERVICE  =0\nREADONLY =0\nDEVELOP  =1\nBITS     =16\nSTEP     =\nMACROS   =0\n---\nNAME     =si2\nGROUP    =ss\nCAPTION  =Смещение датчика тока 2\nUNITS    =\nLIST     =\nADDRESS  =0x0601\nDESCRIP  =Формула расчета I=cur2-511-si2\nMINMAX   =0;4096\nSERVICE  =0\nREADONLY =0\nDEVELOP  =1\nBITS     =16\nSTEP     =\nMACROS   =0\n---\nNAME     =pp6\nGROUP    =pp\nCAPTION  =Ограничение интегральной составляющей контура позиции\nUNITS    =\nLIST     =\nADDRESS  =0x0041\nDESCRIP  =Определяет максимальное значение, до которого может увеличиваться интегральная составляющая. По достижению этой величины интегральная составляющая удерживается константой.\nMINMAX   =0;15000\nSERVICE  =1\nREADONLY =0\nDEVELOP  =0\nBITS     =32\nSTEP     =10\nMACROS   =0\n---\nNAME     =ip11\nGROUP    =ip\nCAPTION  =Статус интерпретатора\nUNITS    =\nLIST     =0:Норма;1:Смена банка программ;2:Неизвестный параметр;3:Неизвестная команда;4:Останов;5:STATUS_UNKNOWN_AL_OP;6:STATUS_UNKNOWN_CMP_OP;7:Загрузка программы;8:STATUS_DEBUG_BREAK;9:STATUS_DEBUG_WAIT_END_OF_CMD;10:Неизвестная динамическая функция;11:Старая версия программы;12:Слишком много циклов;77:Неправильное условие;13:Не удалось найти Z метку;78:Переполнение стека;79:Попытка чтения пустого стека;\nADDRESS  =0x0042\nDESCRIP  =0:Норма;1:Смена банка программ;2:Неизвестный параметр;3:Неизвестная команда;4:Останов;5:STATUS_UNKNOWN_AL_OP;6:STATUS_UNKNOWN_CMP_OP;7:Загрузка программы;8:STATUS_DEBUG_BREAK;9:STATUS_DEBUG_WAIT_END_OF_CMD;10:Неизвестная динамическая функция;\nMINMAX   =0;12\nSERVICE  =0\nREADONLY =1\nDEVELOP  =0\nBITS     =16\nSTEP     =1\nMACROS   =0\n---\nNAME     =ep1\nGROUP    =ep\nCAPTION  =Режим торможения\nUNITS    =\nLIST     =0:Торможение без контроля напряжения;2:Торможение с контролем напряжения;\nADDRESS  =0x0043\nDESCRIP  =При торможении без контроля напряжения привод перейдет в аварийное состояние в момент превышения напряжением допустимого значения, установленным в параметре ep2.\nMINMAX   =0;2\nSERVICE  =0\nREADONLY =0\nDEVELOP  =0\nBITS     =16\nSTEP     =\nMACROS   =0\n---\nNAME     =ep2\nGROUP    =ep\nCAPTION  =Максимальное напряжение\nUNITS    =В\nLIST     =\nADDRESS  =0x0044\nDESCRIP  =Максимальное допустимое напряжение, при котором привод должен переходить в состояние отключения.\nMINMAX   =0;280\nSERVICE  =0\nREADONLY =0\nDEVELOP  =0\nBITS     =16\nSTEP     =0.5\nMACROS   =1\n---\nNAME     =dd15\nGROUP    =dd\nCAPTION  =Время выполнения команды интерпретатором\nUNITS    =мсек\nLIST     =\nADDRESS  =0x0413\nDESCRIP  =Определяет максимальное время, которое интерпретатор затрачивает на выполнение команды в текущей программе.\nMINMAX   =0;2147483647\nSERVICE  =0\nREADONLY =1\nDEVELOP  =0\nBITS     =32\nSTEP     =1\nMACROS   =1\n---\nNAME     =dd16\nGROUP    =dd\nCAPTION  =Время выполнения программы интерпретатором\nUNITS    =мсек\nLIST     =\nADDRESS  =0x0414\nDESCRIP  =Определяет максимальное время, которое интерпретатор затрачивает на выполнение всей программы.\nMINMAX   =0;2147483647\nSERVICE  =0\nREADONLY =1\nDEVELOP  =0\nBITS     =32\nSTEP     =1\nMACROS   =1\n---\nNAME     =ip12\nGROUP    =ip\nCAPTION  =Мертвая зона аналоговых входов\nUNITS    =дискрет\nLIST     =\nADDRESS  =0x0045\nDESCRIP  =Определяет зону нечувствительности аналоговых входов привода. При ручном управлении, например, с помощью джойстика, данный параметр позволяет исключить вращение вала при задании нулевой скорости.\nMINMAX   =0;250\nSERVICE  =0\nREADONLY =0\nDEVELOP  =0\nBITS     =16\nSTEP     =\nMACROS   =0\n---\nNAME     =dd17\nGROUP    =dd\nCAPTION  =Аналоговый вход 0\nUNITS    =дискрет\nLIST     =\nADDRESS  =0x0415\nDESCRIP  =\nMINMAX   =-65535;65535\nSERVICE  =0\nREADONLY =1\nDEVELOP  =0\nBITS     =16\nSTEP     =\nMACROS   =0\n---\nNAME     =dd18\nGROUP    =dd\nCAPTION  =Аналоговый вход 1\nUNITS    =дискрет\nLIST     =\nADDRESS  =0x0416\nDESCRIP  =\nMINMAX   =-65535;65535\nSERVICE  =0\nREADONLY =1\nDEVELOP  =0\nBITS     =16\nSTEP     =\nMACROS   =0\n---\nNAME     =up0\nGROUP    =up\nCAPTION  =Переменная общего назначения 0\nUNITS    =\nLIST     =\nADDRESS  =0x0700\nDESCRIP  =Может использоваться для общих целей. Например, для запоминания длинны оси, приводимой в движение данным приводом и т.д.\nMINMAX   =-2147483647;2147483647\nSERVICE  =0\nREADONLY =0\nDEVELOP  =0\nBITS     =32\nSTEP     =\nMACROS   =0\n---\nNAME     =up1\nGROUP    =up\nCAPTION  =Переменная общего назначения 1\nUNITS    =\nLIST     =\nADDRESS  =0x0701\nDESCRIP  =Может использоваться для общих целей. Например, для запоминания длинны оси, приводимой в движение данным приводом и т.д.\nMINMAX   =-2147483647;2147483647\nSERVICE  =0\nREADONLY =0\nDEVELOP  =0\nBITS     =32\nSTEP     =\nMACROS   =0\n---\nNAME     =up2\nGROUP    =up\nCAPTION  =Переменная общего назначения 2\nUNITS    =\nLIST     =\nADDRESS  =0x0702\nDESCRIP  =Может использоваться для общих целей. Например, для запоминания длинны оси, приводимой в движение данным приводом и т.д.\nMINMAX   =-2147483647;2147483647\nSERVICE  =0\nREADONLY =0\nDEVELOP  =0\nBITS     =32\nSTEP     =\nMACROS   =0\n---\nNAME     =up3\nGROUP    =up\nCAPTION  =Переменная общего назначения 3\nUNITS    =\nLIST     =\nADDRESS  =0x0703\nDESCRIP  =Может использоваться для общих целей. Например, для запоминания длинны оси, приводимой в движение данным приводом и т.д.\nMINMAX   =-2147483647;2147483647\nSERVICE  =0\nREADONLY =0\nDEVELOP  =0\nBITS     =32\nSTEP     =\nMACROS   =0\n---\nNAME     =up4\nGROUP    =up\nCAPTION  =Переменная общего назначения 4\nUNITS    =\nLIST     =\nADDRESS  =0x0704\nDESCRIP  =Может использоваться для общих целей. Например, для запоминания длинны оси, приводимой в движение данным приводом и т.д.\nMINMAX   =-2147483647;2147483647\nSERVICE  =0\nREADONLY =0\nDEVELOP  =0\nBITS     =32\nSTEP     =\nMACROS   =0\n---\nNAME     =up5\nGROUP    =up\nCAPTION  =Переменная общего назначения 5\nUNITS    =\nLIST     =\nADDRESS  =0x0705\nDESCRIP  =Может использоваться для общих целей. Например, для запоминания длинны оси, приводимой в движение данным приводом и т.д.\nMINMAX   =-2147483647;2147483647\nSERVICE  =0\nREADONLY =0\nDEVELOP  =0\nBITS     =32\nSTEP     =\nMACROS   =0\n---\nNAME     =up6\nGROUP    =up\nCAPTION  =Переменная общего назначения 6\nUNITS    =\nLIST     =\nADDRESS  =0x0706\nDESCRIP  =Может использоваться для общих целей. Например, для запоминания длинны оси, приводимой в движение данным приводом и т.д.\nMINMAX   =-2147483647;2147483647\nSERVICE  =0\nREADONLY =0\nDEVELOP  =0\nBITS     =32\nSTEP     =\nMACROS   =0\n---\nNAME     =up7\nGROUP    =up\nCAPTION  =Переменная общего назначения 7\nUNITS    =\nLIST     =\nADDRESS  =0x0707\nDESCRIP  =Может использоваться для общих целей. Например, для запоминания длинны оси, приводимой в движение данным приводом и т.д.\nMINMAX   =-2147483647;2147483647\nSERVICE  =0\nREADONLY =0\nDEVELOP  =0\nBITS     =32\nSTEP     =\nMACROS   =0\n---\nNAME     =st4\nGROUP    =st\nCAPTION  =Тип привода\nUNITS    =\nLIST     =1:СПШ10-23xx;2:СПШ20-23xx\\1000Z;4:СПШ20-23xx\\2000Z;64:СПШ10-34xx;128:СПШ20-34xx\\2000Z;4096:СПШ20-34xx\\1000Z;8192:СПС25-80007;8193:СПС25-80016;8194:СПС25-80025;8195:СПС25-1100075;8196:СПС30-хххх;\nADDRESS  =0x0046\nDESCRIP  =\nMINMAX   =1;65535\nSERVICE  =0\nREADONLY =0\nDEVELOP  =0\nBITS     =16\nSTEP     =\nMACROS   =0\n---\nNAME     =st5\nGROUP    =st\nCAPTION  =Z метка\nUNITS    =\nLIST     =0:Нет;1:Да;\nADDRESS  =0x0047\nDESCRIP  =Наличие или отсутствие у датчика позиции канала нуливой метки\nMINMAX   =0;1\nSERVICE  =0\nREADONLY =0\nDEVELOP  =0\nBITS     =16\nSTEP     =\nMACROS   =0\n---\nNAME     =cp6\nGROUP    =cp\nCAPTION  =Вырабатываемый момент\nUNITS    =\nLIST     =100:100%;75:75%;50:50%;25:25%;\nADDRESS  =0x0048\nDESCRIP  =Параметр позволяет ограничить развиваемый момент\nMINMAX   =25;100\nSERVICE  =0\nREADONLY =0\nDEVELOP  =1\nBITS     =16\nSTEP     =\nMACROS   =0\n---\nNAME     =ep3\nGROUP    =ep\nCAPTION  =Ток поиска фазы\nUNITS    =дискрет\nLIST     =\nADDRESS  =0x0051\nDESCRIP  =Определяет уровень тока, который устанавливается при поиске фазы. Ток задается в дискретах.\nMINMAX   =0;32000\nSERVICE  =0\nREADONLY =0\nDEVELOP  =0\nBITS     =16\nSTEP     =1\nMACROS   =0\n---\nNAME     =ep4\nGROUP    =ep\nCAPTION  =Время поиска фазы\nUNITS    =дискрет\nLIST     =\nADDRESS  =0x0052\nDESCRIP  =Определяет время, в течение которого будет удерживаться ток ep3 при поиске фазы.\nMINMAX   =0;32000\nSERVICE  =0\nREADONLY =0\nDEVELOP  =0\nBITS     =16\nSTEP     =1\nMACROS   =0\n---\nNAME     =ep5\nGROUP    =ep\nCAPTION  =Максимальная температура\nUNITS    =град.\nLIST     =\nADDRESS  =0x0054\nDESCRIP  =Указывает максимальную допустимую температуру внутри корпуса\nMINMAX   =25;85\nSERVICE  =0\nREADONLY =0\nDEVELOP  =0\nBITS     =16\nSTEP     =1\nMACROS   =0\n---\nNAME     =cp7\nGROUP    =cp\nCAPTION  =Модуляция ШИМ сигнала\nUNITS    =\nLIST     =0:Выключена;1:Включена;\nADDRESS  =0x0053\nDESCRIP  =Разрешает/запрещает подачу силового напряжения на обмотки двигателя\nMINMAX   =0;1\nSERVICE  =0\nREADONLY =0\nDEVELOP  =0\nBITS     =16\nSTEP     =\nMACROS   =0\n---\nNAME     =ep6\nGROUP    =ep\nCAPTION  =Период поиска фазы\nUNITS    =\nLIST     =0:Однопериодный;1:1;2:2;3:3;\nADDRESS  =0x0056\nDESCRIP  =Один из трех периодов, во время которого привод может выполнять поиск фазы. В результате удается избежать перегрузки источника питания и выполнить корректный поиск фазы в приводах, между которыми имеется жесткая механическая связь.\nMINMAX   =0;3\nSERVICE  =0\nREADONLY =0\nDEVELOP  =0\nBITS     =16\nSTEP     =1\nMACROS   =0\n---\nNAME     =up8\nGROUP    =up\nCAPTION  =X\nUNITS    =\nLIST     =\nADDRESS  =0x0708\nDESCRIP  =Переменная, используемая в ПЛК\nMINMAX   =-2147483647;2147483647\nSERVICE  =0\nREADONLY =0\nDEVELOP  =0\nBITS     =32\nSTEP     =1\nMACROS   =0\n---\nNAME     =up9\nGROUP    =up\nCAPTION  =Y\nUNITS    =\nLIST     =\nADDRESS  =0x0709\nDESCRIP  =Переменная, используемая в ПЛК\nMINMAX   =-2147483647;2147483647\nSERVICE  =0\nREADONLY =0\nDEVELOP  =0\nBITS     =32\nSTEP     =1\nMACROS   =0\n---\nNAME     =up10\nGROUP    =up\nCAPTION  =Z\nUNITS    =\nLIST     =\nADDRESS  =0x070A\nDESCRIP  =Переменная, используемая в ПЛК\nMINMAX   =-2147483647;2147483647\nSERVICE  =0\nREADONLY =0\nDEVELOP  =0\nBITS     =32\nSTEP     =1\nMACROS   =0\n---\nNAME     =up11\nGROUP    =up\nCAPTION  =EEPROM массив\nUNITS    =\nLIST     =\nADDRESS  =0x070B\nDESCRIP  =User EEPROM massive\nMINMAX   =-2147483647;2147483647\nSERVICE  =0\nREADONLY =0\nDEVELOP  =1\nBITS     =32\nSTEP     =1\nMACROS   =0\n---\nNAME     =up12\nGROUP    =up\nCAPTION  =EEPROM массив метаданных\nUNITS    =\nLIST     =\nADDRESS  =0x070C\nDESCRIP  =Metadata massive of params of motor\nMINMAX   =-2147483647;2147483647\nSERVICE  =0\nREADONLY =0\nDEVELOP  =1\nBITS     =32\nSTEP     =1\nMACROS   =0\n---\nNAME     =dd22\nGROUP    =dd\nCAPTION  =Максимальное отклонение от траектории\nUNITS    =дискрет\nLIST     =\nADDRESS  =0x0420\nDESCRIP  =Определяет максимальную ошибку контура позиции зафиксированную при прохождении траектории.\nMINMAX   =0;65535\nSERVICE  =0\nREADONLY =0\nDEVELOP  =0\nBITS     =16\nSTEP     =\nMACROS   =0\n---\nNAME     =ip13\nGROUP    =ip\nCAPTION  =Ограничитель левый\nUNITS    =имп.\nLIST     =\nADDRESS  =0x0057\nDESCRIP  =Программный ограничитель позиции,  при достижении которой привод останавливается и воспринимает команду управления только в противоположную сторону.\nMINMAX   =-2147483647;2147483647\nSERVICE  =0\nREADONLY =0\nDEVELOP  =0\nBITS     =32\nSTEP     =\nMACROS   =0\n---\nNAME     =ip14\nGROUP    =ip\nCAPTION  =Ограничитель правый\nUNITS    =имп.\nLIST     =\nADDRESS  =0x0058\nDESCRIP  =Программный ограничитель позиции,  при достижении которой привод останавливается и воспринимает команду управления только в противоположную сторону.\nMINMAX   =-2147483647;2147483647\nSERVICE  =0\nREADONLY =0\nDEVELOP  =0\nBITS     =32\nSTEP     =\nMACROS   =0\n---\nNAME     =dd23\nGROUP    =dd\nCAPTION  =Статус G декодера\nUNITS    =\nLIST     =0:Останов;1:Начало;2:Отработка;3:Ожидание подтверждений;4:Ошибка;5:Выход в нуль\nADDRESS  =0x0421\nDESCRIP  =\nMINMAX   =0;5\nSERVICE  =0\nREADONLY =1\nDEVELOP  =1\nBITS     =16\nSTEP     =\nMACROS   =0\n---\nNAME     =dd24\nGROUP    =dd\nCAPTION  =Текущий кадр G декодера\nUNITS    =\nLIST     =\nADDRESS  =0x0422\nDESCRIP  =\nMINMAX   =0;65535\nSERVICE  =0\nREADONLY =1\nDEVELOP  =1\nBITS     =16\nSTEP     =\nMACROS   =0\n---\nNAME     =ip15\nGROUP    =ip\nCAPTION  =Скорость обмена по шине CAN\nUNITS    =\nLIST     =500:500 кБит/сек;1000:1000 кБит/сек;\nADDRESS  =0x0059\nDESCRIP  =Определяет скорость обмена по шине CAN. При этом допустимая скорость определяется дальностью линии связи. На скорость 1000кБит максимальная дальность 60м, 500кБит - 120м\nMINMAX   =50;1000\nSERVICE  =0\nREADONLY =0\nDEVELOP  =0\nBITS     =16\nSTEP     =\nMACROS   =0\n---\nNAME     =cp8\nGROUP    =cp\nCAPTION  =Частота ШИМ сигнала\nUNITS    =кГц\nLIST     =2500:40кГц;5000:20кГц;6250:16кГц;12500:8кГц;25000:4кГц;\nADDRESS  =0x0060\nDESCRIP  =Определяет частоту ШИМ сигнала и частоту работы контура тока. Влияет на КПД силовой части привода, а также качество работы контура тока. Для приводов серии СПШ частота всегда 40кГц. Влияет на параметр cp4.\nMINMAX   =-65535;65535\nSERVICE  =0\nREADONLY =0\nDEVELOP  =0\nBITS     =16\nSTEP     =\nMACROS   =0\n---\nNAME     =ip16\nGROUP    =ip\nCAPTION  =USB2CAN конвертор\nUNITS    =\nLIST     =0:Выкл;2:Вкл;\nADDRESS  =0x0061\nDESCRIP  =Данная функция предназначена для облегчения подключения к группе приводов СПШ/СПС, которые объединены в рамках системы в одну сеть CAN. Чтобы работать со всеми приводами сети достаточно подключиться только к одному приводу по USB.\nMINMAX   =0;2\nSERVICE  =0\nREADONLY =0\nDEVELOP  =0\nBITS     =16\nSTEP     =\nMACROS   =0\n---\nNAME     =up13\nGROUP    =up\nCAPTION  =Значение текущего элемента EEPROM массива\nUNITS    =\nLIST     =\nADDRESS  =0x070D\nDESCRIP  =Отображает значение текущего элемента массива энергонезависимой памяти данных общего назначения.\nMINMAX   =-2147483647;2147483647\nSERVICE  =0\nREADONLY =0\nDEVELOP  =0\nBITS     =32\nSTEP     =1\nMACROS   =0\n---\nNAME     =up14\nGROUP    =up\nCAPTION  =Индекс текущего элемента EEPROM массива\nUNITS    =\nLIST     =\nADDRESS  =0x070E\nDESCRIP  =Отображает индекс текущего элемента массива энергонезависимой памяти данных общего назначения.\nMINMAX   =-2147483647;2147483647\nSERVICE  =0\nREADONLY =0\nDEVELOP  =0\nBITS     =32\nSTEP     =1\nMACROS   =0\n---\nNAME     =up15\nGROUP    =up\nCAPTION  =Значение счетчика импульсов\nUNITS    =\nLIST     =\nADDRESS  =0x070F\nDESCRIP  =Отображает значение счетчика импульсов, которые приходят на порты IN0, IN1, по протоколу Step\\Dir или по квадратурному протоколу. Счетчик активизирован только при выборе соответствующего протокола.\nMINMAX   =-2147483647;2147483647\nSERVICE  =0\nREADONLY =0\nDEVELOP  =0\nBITS     =32\nSTEP     =1\nMACROS   =0\n---\nNAME     =up16\nGROUP    =up\nCAPTION  =Среднее значение заданного тока\nUNITS    =\nLIST     =\nADDRESS  =0x0710\nDESCRIP  =Величина пропорциональна вырабатываемому приводом моменту, используется в программах для определения развиваемого момента.\nMINMAX   =-65535;65535\nSERVICE  =0\nREADONLY =1\nDEVELOP  =0\nBITS     =16\nSTEP     =1\nMACROS   =0\n---\nNAME     =ip17\nGROUP    =ip\nCAPTION  =Таймаут передачи синхронизации слейву\nUNITS    =мксек\nLIST     =\nADDRESS  =0x0800\nDESCRIP  =Временной интервал, в течение которого мастер обязан передать синхронизацию слейву. По истечении этого времени параметр ip10 будет установлен в значение 1 или 2.\nMINMAX   =0;10000\nSERVICE  =0\nREADONLY =0\nDEVELOP  =0\nBITS     =16\nSTEP     =25\nMACROS   =0\n---\nNAME     =ip18\nGROUP    =ip\nCAPTION  =Таймаут передачи подтверждения мастеру от слейва\nUNITS    =мксек\nLIST     =\nADDRESS  =0x0801\nDESCRIP  =Временной интервал, в течение которого слейв обязан передать подтверждение на команду синхронизации мастеру. По истечении этого времени параметр ip10 будет установлен в значение 3.\nMINMAX   =0;10000\nSERVICE  =0\nREADONLY =0\nDEVELOP  =0\nBITS     =16\nSTEP     =25\nMACROS   =0\n---\nNAME     =st6\nGROUP    =st\nCAPTION  =Нулевой сектор сигналов UVW\nUNITS    =\nLIST     =1:1;2:2;3:3;4:4;5:5;6:6;170:Выполнить инициализацию;85:Не использовать UVW треки;\nADDRESS  =0x0802\nDESCRIP  =Определяет сектор датчика UVW, в котором находится нуль двигателя. Если установить значение \"Выполнить инициализацию\", то при следующем запуске автоматически будет выполнена операция поиска сектора и смещения внутри сектора\nMINMAX   =0;170\nSERVICE  =0\nREADONLY =0\nDEVELOP  =0\nBITS     =16\nSTEP     =\nMACROS   =0\n---\nNAME     =st7\nGROUP    =st\nCAPTION  =Сдвиг нуля внутри сектора сигналов UVW\nUNITS    =\nLIST     =\nADDRESS  =0x0804\nDESCRIP  =Определяет смещение внутри сектора датчика UVW, в котором находится нуль двигателя. Если установить значение \"Выполнить инициализацию\", то при следующем запуске автоматически будет выполнена операция поиска сектора и смещения внутри сектора\nMINMAX   =0;80000\nSERVICE  =0\nREADONLY =0\nDEVELOP  =0\nBITS     =16\nSTEP     =\nMACROS   =0\n---\nNAME     =io0\nGROUP    =io\nCAPTION  =Порт ввода 0\nUNITS    =\nLIST     =\nADDRESS  =0x0805\nDESCRIP  =Значение порта ввода 0\nMINMAX   =0;1\nSERVICE  =0\nREADONLY =0\nDEVELOP  =0\nBITS     =16\nSTEP     =\nMACROS   =0\n---\nNAME     =io1\nGROUP    =io\nCAPTION  =Порт ввода 1\nUNITS    =\nLIST     =\nADDRESS  =0x0806\nDESCRIP  =Значение порта ввода 1\nMINMAX   =0;1\nSERVICE  =0\nREADONLY =0\nDEVELOP  =0\nBITS     =16\nSTEP     =\nMACROS   =0\n---\nNAME     =io2\nGROUP    =io\nCAPTION  =Порт ввода 2\nUNITS    =\nLIST     =\nADDRESS  =0x0807\nDESCRIP  =Значение порта ввода 2\nMINMAX   =0;1\nSERVICE  =0\nREADONLY =0\nDEVELOP  =0\nBITS     =16\nSTEP     =\nMACROS   =0\n---\nNAME     =io3\nGROUP    =io\nCAPTION  =Порт ввода 3\nUNITS    =\nLIST     =\nADDRESS  =0x0808\nDESCRIP  =Значение порта ввода 3\nMINMAX   =0;1\nSERVICE  =0\nREADONLY =0\nDEVELOP  =0\nBITS     =16\nSTEP     =\nMACROS   =0\n---\nNAME     =io4\nGROUP    =io\nCAPTION  =Порт вывода 0\nUNITS    =\nLIST     =\nADDRESS  =0x0809\nDESCRIP  =Значение порта вывода 0\nMINMAX   =0;1\nSERVICE  =0\nREADONLY =0\nDEVELOP  =0\nBITS     =16\nSTEP     =\nMACROS   =0\n---\nNAME     =io5\nGROUP    =io\nCAPTION  =Порт вывода 1\nUNITS    =\nLIST     =\nADDRESS  =0x080A\nDESCRIP  =Значение порта вывода 1\nMINMAX   =0;1\nSERVICE  =0\nREADONLY =0\nDEVELOP  =0\nBITS     =16\nSTEP     =\nMACROS   =0\n---\nNAME     =io6\nGROUP    =io\nCAPTION  =PWM0\nUNITS    =\nLIST     =\nADDRESS  =0x080B\nDESCRIP  =Скваженность ШИМ сигнала, выводимого на порт вывода 0. Порт необходимо соответствующим образом настроить с помощью параметра: Режим работы порта вывода.\nMINMAX   =0;160\nSERVICE  =0\nREADONLY =0\nDEVELOP  =0\nBITS     =16\nSTEP     =1\nMACROS   =0\n---\nNAME     =io7\nGROUP    =io\nCAPTION  =PWM1\nUNITS    =\nLIST     =\nADDRESS  =0x080C\nDESCRIP  =Скваженность ШИМ сигнала, выводимого на порт вывода 1. Порт необходимо соответствующим образом настроить с помощью параметра: Режим работы порта вывода.\nMINMAX   =0;160\nSERVICE  =0\nREADONLY =0\nDEVELOP  =0\nBITS     =16\nSTEP     =1\nMACROS   =0\n---\nNAME     =io8\nGROUP    =io\nCAPTION  =Режим порта ввода 0\nUNITS    =\nLIST     =0:Порт ввода общего назначения;1:Порт ввода в режиме квадратурного счетчика;2:Порт ввода в режиме счетчика Step/dir;\nADDRESS  =0x080D\nDESCRIP  =Определяет режим работы порта ввода.\nMINMAX   =0;3\nSERVICE  =0\nREADONLY =0\nDEVELOP  =0\nBITS     =16\nSTEP     =1\nMACROS   =0\n---\nNAME     =io9\nGROUP    =io\nCAPTION  =Режим порта ввода 1\nUNITS    =\nLIST     =0:Порт ввода общего назначения;1:Порт ввода в режиме квадратурного счетчика;2:Порт ввода в режиме счетчика Step/dir;\nADDRESS  =0x080E\nDESCRIP  =Определяет режим работы порта ввода.\nMINMAX   =0;3\nSERVICE  =0\nREADONLY =0\nDEVELOP  =0\nBITS     =16\nSTEP     =1\nMACROS   =0\n---\nNAME     =io10\nGROUP    =io\nCAPTION  =Режим порта ввода 2\nUNITS    =\nLIST     =0:Порт ввода общего назначения;1:Порт ввода в режиме квадратурного счетчика;2:Порт ввода в режиме счетчика Step/dir;\nADDRESS  =0x080F\nDESCRIP  =Определяет режим работы порта ввода.\nMINMAX   =0;3\nSERVICE  =0\nREADONLY =0\nDEVELOP  =0\nBITS     =16\nSTEP     =1\nMACROS   =0\n---\nNAME     =io11\nGROUP    =io\nCAPTION  =Режим порта ввода 3\nUNITS    =\nLIST     =0:Порт ввода общего назначения;1:Порт ввода в режиме квадратурного счетчика;2:Порт ввода в режиме счетчика Step/dir;\nADDRESS  =0x0810\nDESCRIP  =Определяет режим работы порта ввода.\nMINMAX   =0;3\nSERVICE  =0\nREADONLY =0\nDEVELOP  =0\nBITS     =16\nSTEP     =1\nMACROS   =0\n---\nNAME     =io12\nGROUP    =io\nCAPTION  =Режим порта вывода 0\nUNITS    =\nLIST     =0:Порт вывода общего назначения;1:Порт вывода в режиме ШИМ;\nADDRESS  =0x0811\nDESCRIP  =Определяет режим работы порта вывода.\nMINMAX   =0;3\nSERVICE  =0\nREADONLY =0\nDEVELOP  =0\nBITS     =16\nSTEP     =1\nMACROS   =0\n---\nNAME     =io13\nGROUP    =io\nCAPTION  =Режим порта вывода 1\nUNITS    =\nLIST     =0:Порт вывода общего назначения;1:Порт вывода в режиме ШИМ;\nADDRESS  =0x0812\nDESCRIP  =Определяет режим работы порта вывода.\nMINMAX   =0;3\nSERVICE  =0\nREADONLY =0\nDEVELOP  =0\nBITS     =16\nSTEP     =1\nMACROS   =0\n---\nNAME     =io14\nGROUP    =io\nCAPTION  =Счетчик импульсов\nUNITS    =\nLIST     =\nADDRESS  =0x070F\nDESCRIP  =Аппаратный счетчик импульсов,  которые приходят на входы In0 и In1. При этом порты должны быть настроены на соответствующий интерфейс (см. параметры io8 и io9).\nMINMAX   =-2147483647;2147483647\nSERVICE  =0\nREADONLY =1\nDEVELOP  =0\nBITS     =32\nSTEP     =1\nMACROS   =0\n---\nNAME     =dd25\nGROUP    =dd\nCAPTION  =UVW треки\nUNITS    =\nLIST     =\nADDRESS  =0x0423\nDESCRIP  =Сигнал, считанный с UVW треков энкодера\nMINMAX   =0;16\nSERVICE  =0\nREADONLY =1\nDEVELOP  =0\nBITS     =16\nSTEP     =\nMACROS   =0\n---\nNAME     =st8\nGROUP    =st\nCAPTION  =Тип энкодера\nUNITS    =\nLIST     =0:Инкрементальный;1:Абсолютный;\nADDRESS  =0x0062\nDESCRIP  =\nMINMAX   =0;1\nSERVICE  =0\nREADONLY =0\nDEVELOP  =0\nBITS     =32\nSTEP     =1\nMACROS   =0\n---\nNAME     =vp17\nGROUP    =vp\nCAPTION  =Рывок\nUNITS    =\nLIST     =\nADDRESS  =0x0063\nDESCRIP  =Ограничивает вторую производную скорости. Параметр вступает в силу только при установки vp9 в значение 4\nMINMAX   =1;21470\nSERVICE  =1\nREADONLY =0\nDEVELOP  =0\nBITS     =32\nSTEP     =10\nMACROS   =0\n---\nNAME     =cp9\nGROUP    =cp\nCAPTION  =Допустимая перегрузка\nUNITS    =А2сек\nLIST     =\nADDRESS  =0x0814\nDESCRIP  =Ограничение выделяемой мощности обмотками двигателя. Предотвращает повреждения обмоток. Реализует защитную функцию I2t\nMINMAX   =0;350\nSERVICE  =1\nREADONLY =0\nDEVELOP  =0\nBITS     =32\nSTEP     =16\nMACROS   =0\n---\nNAME     =cp10\nGROUP    =cp\nCAPTION  =Номинальный ток\nUNITS    =А\nLIST     =\nADDRESS  =0x0815\nDESCRIP  =\nMINMAX   =0;850\nSERVICE  =1\nREADONLY =0\nDEVELOP  =0\nBITS     =32\nSTEP     =16\nMACROS   =1\n---\nNAME     =dd26\nGROUP    =dd\nCAPTION  =Текущая перегрузка\nUNITS    =А2сек\nLIST     =\nADDRESS  =0x0424\nDESCRIP  =Накомпленнае мощность, превышающая номинальные характеристики двигателя\nMINMAX   =0;100\nSERVICE  =1\nREADONLY =1\nDEVELOP  =0\nBITS     =32\nSTEP     =16\nMACROS   =0\n---\nNAME     =dd27\nGROUP    =dd\nCAPTION  =Ток в обмотке 3\nUNITS    =А\nLIST     =\nADDRESS  =0x0425\nDESCRIP  =Показывает ток, протекающий в обмотке двигателя. Параметр действителен только для СПС.\nMINMAX   =-5;5\nSERVICE  =0\nREADONLY =1\nDEVELOP  =0\nBITS     =16\nSTEP     =0.05\nMACROS   =1\n---\nNAME     =dd28\nGROUP    =dd\nCAPTION  =Заданный ток в обмотке 3\nUNITS    =А\nLIST     =\nADDRESS  =0x0426\nDESCRIP  =Заданный ток в обмотке 3. Действителен только для приводов серии СПС.\nMINMAX   =-2047;2047\nSERVICE  =0\nREADONLY =0\nDEVELOP  =0\nBITS     =16\nSTEP     =\nMACROS   =1\n---\nNAME     =dd29\nGROUP    =dd\nCAPTION  =Ток потребления двигателя\nUNITS    =А\nLIST     =\nADDRESS  =0x0427\nDESCRIP  =Параметр действителен только для СПС.\nMINMAX   =-5;5\nSERVICE  =0\nREADONLY =1\nDEVELOP  =0\nBITS     =16\nSTEP     =0.05\nMACROS   =1\n---\nNAME     =pd1\nGROUP    =pd\nCAPTION  =Зона нечувствительности\nUNITS    =\nLIST     =\nADDRESS  =0x0A01\nDESCRIP  =Параметр настройки ПИД-регулятора\nMINMAX   =0;10000\nSERVICE  =1\nREADONLY =0\nDEVELOP  =0\nBITS     =32\nSTEP     =12\nMACROS   =0\n---\nNAME     =pd2\nGROUP    =pd\nCAPTION  =Максимальная ошибка\nUNITS    =\nLIST     =\nADDRESS  =0x0A02\nDESCRIP  =Параметр настройки ПИД-регулятора\nMINMAX   =0;524287\nSERVICE  =1\nREADONLY =0\nDEVELOP  =0\nBITS     =32\nSTEP     =12\nMACROS   =0\n---\nNAME     =pd3\nGROUP    =pd\nCAPTION  =Пропорциональный коэффициент\nUNITS    =\nLIST     =\nADDRESS  =0x0A03\nDESCRIP  =Параметр настройки ПИД-регулятора\nMINMAX   =0;10000\nSERVICE  =1\nREADONLY =0\nDEVELOP  =0\nBITS     =32\nSTEP     =12\nMACROS   =0\n---\nNAME     =pd4\nGROUP    =pd\nCAPTION  =Интегральный коэффициент\nUNITS    =\nLIST     =\nADDRESS  =0x0A04\nDESCRIP  =Параметр настройки ПИД-регулятора\nMINMAX   =0;10000\nSERVICE  =1\nREADONLY =0\nDEVELOP  =0\nBITS     =32\nSTEP     =12\nMACROS   =0\n---\nNAME     =pd5\nGROUP    =pd\nCAPTION  =Дифференциальный коэффициент\nUNITS    =\nLIST     =\nADDRESS  =0x0A05\nDESCRIP  =Параметр настройки ПИД-регулятора\nMINMAX   =0;10000\nSERVICE  =1\nREADONLY =0\nDEVELOP  =0\nBITS     =32\nSTEP     =12\nMACROS   =0\n---\nNAME     =pd6\nGROUP    =pd\nCAPTION  =Ограничение интегральной составляющей\nUNITS    =\nLIST     =\nADDRESS  =0x0A06\nDESCRIP  =Параметр настройки ПИД-регулятора\nMINMAX   =0;100000\nSERVICE  =1\nREADONLY =0\nDEVELOP  =0\nBITS     =32\nSTEP     =12\nMACROS   =0\n---\nNAME     =pd7\nGROUP    =pd\nCAPTION  =Ограничение дифференциальной составляющей\nUNITS    =\nLIST     =\nADDRESS  =0x0A07\nDESCRIP  =Параметр настройки ПИД-регулятора\nMINMAX   =0;100000\nSERVICE  =1\nREADONLY =0\nDEVELOP  =0\nBITS     =32\nSTEP     =12\nMACROS   =0\n---\nNAME     =pd8\nGROUP    =pd\nCAPTION  =Ограничение форсирующей составляющей 1го порядка\nUNITS    =\nLIST     =\nADDRESS  =0x0A08\nDESCRIP  =Параметр настройки ПИД-регулятора\nMINMAX   =0;524287\nSERVICE  =1\nREADONLY =0\nDEVELOP  =0\nBITS     =32\nSTEP     =12\nMACROS   =0\n---\nNAME     =pd9\nGROUP    =pd\nCAPTION  =Ограничение форсирующей составляющей 2го порядка\nUNITS    =\nLIST     =\nADDRESS  =0x0A09\nDESCRIP  =Параметр настройки ПИД-регулятора\nMINMAX   =0;524287\nSERVICE  =1\nREADONLY =0\nDEVELOP  =0\nBITS     =32\nSTEP     =12\nMACROS   =0\n---\nNAME     =pd10\nGROUP    =pd\nCAPTION  =Коэффициент форсирующей составляющей 0го порядка\nUNITS    =\nLIST     =\nADDRESS  =0x0A0A\nDESCRIP  =Параметр настройки ПИД-регулятора\nMINMAX   =0;10000\nSERVICE  =1\nREADONLY =0\nDEVELOP  =0\nBITS     =32\nSTEP     =12\nMACROS   =0\n---\nNAME     =pd11\nGROUP    =pd\nCAPTION  =Коэффициент форсирующей составляющей 1го порядка\nUNITS    =\nLIST     =\nADDRESS  =0x0A0B\nDESCRIP  =Параметр настройки ПИД-регулятора\nMINMAX   =0;10000\nSERVICE  =1\nREADONLY =0\nDEVELOP  =0\nBITS     =32\nSTEP     =12\nMACROS   =0\n---\nNAME     =pd12\nGROUP    =pd\nCAPTION  =Коэффициент форсирующей составляющей 2го порядка\nUNITS    =\nLIST     =\nADDRESS  =0x0A0C\nDESCRIP  =Параметр настройки ПИД-регулятора\nMINMAX   =0;10000\nSERVICE  =1\nREADONLY =0\nDEVELOP  =0\nBITS     =32\nSTEP     =12\nMACROS   =0\n---\nNAME     =pd13\nGROUP    =pd\nCAPTION  =Смещение сигнала управления\nUNITS    =\nLIST     =\nADDRESS  =0x0A0D\nDESCRIP  =Параметр настройки ПИД-регулятора\nMINMAX   =-524286;524287\nSERVICE  =1\nREADONLY =0\nDEVELOP  =0\nBITS     =32\nSTEP     =12\nMACROS   =0\n---\nNAME     =pd14\nGROUP    =pd\nCAPTION  =Ограничение выходного сигнала\nUNITS    =\nLIST     =\nADDRESS  =0x0A0E\nDESCRIP  =Параметр настройки ПИД-регулятора\nMINMAX   =0;524287\nSERVICE  =1\nREADONLY =0\nDEVELOP  =0\nBITS     =32\nSTEP     =12\nMACROS   =0\n---\nNAME     =pd15\nGROUP    =pd\nCAPTION  =Задание регулятора\nUNITS    =\nLIST     =\nADDRESS  =0x0A0F\nDESCRIP  =Параметр настройки ПИД-регулятора\nMINMAX   =-524286;524287\nSERVICE  =1\nREADONLY =0\nDEVELOP  =0\nBITS     =32\nSTEP     =12\nMACROS   =0\n---\nNAME     =pd16\nGROUP    =pd\nCAPTION  =Обратная связь\nUNITS    =\nLIST     =\nADDRESS  =0x0A10\nDESCRIP  =Параметр настройки ПИД-регулятора\nMINMAX   =-524286;524287\nSERVICE  =1\nREADONLY =1\nDEVELOP  =0\nBITS     =32\nSTEP     =12\nMACROS   =0\n---\nNAME     =pd17\nGROUP    =pd\nCAPTION  =Ошибка\nUNITS    =\nLIST     =\nADDRESS  =0x0A11\nDESCRIP  =Параметр настройки ПИД-регулятора\nMINMAX   =-524286;524287\nSERVICE  =1\nREADONLY =1\nDEVELOP  =0\nBITS     =32\nSTEP     =12\nMACROS   =0\n---\nNAME     =pp7\nGROUP    =pp\nCAPTION  =Ограничение форсирующей составляющей 1го порядка\nUNITS    =\nLIST     =\nADDRESS  =0x0A12\nDESCRIP  =Параметр настройки ПИД-регулятора\nMINMAX   =0;524287\nSERVICE  =1\nREADONLY =0\nDEVELOP  =0\nBITS     =32\nSTEP     =10\nMACROS   =0\n---\nNAME     =pp8\nGROUP    =pp\nCAPTION  =Ограничение форсирующей составляющей 2го порядка\nUNITS    =\nLIST     =\nADDRESS  =0x0A13\nDESCRIP  =Параметр настройки ПИД-регулятора\nMINMAX   =0;524287\nSERVICE  =1\nREADONLY =0\nDEVELOP  =0\nBITS     =32\nSTEP     =10\nMACROS   =0\n---\nNAME     =pp9\nGROUP    =pp\nCAPTION  =Коэффициент форсирующей составляющей 1го порядка\nUNITS    =\nLIST     =\nADDRESS  =0x0A14\nDESCRIP  =Параметр настройки ПИД-регулятора\nMINMAX   =0;100000\nSERVICE  =1\nREADONLY =0\nDEVELOP  =0\nBITS     =32\nSTEP     =10\nMACROS   =0\n---\nNAME     =pp10\nGROUP    =pp\nCAPTION  =Коэффициент форсирующей составляющей 2го порядка\nUNITS    =\nLIST     =\nADDRESS  =0x0A15\nDESCRIP  =Параметр настройки ПИД-регулятора\nMINMAX   =0;100000\nSERVICE  =1\nREADONLY =0\nDEVELOP  =0\nBITS     =32\nSTEP     =10\nMACROS   =0\n---\nNAME     =vp18\nGROUP    =vp\nCAPTION  =Зона нечувствительности входного сигнала\nUNITS    =\nLIST     =\nADDRESS  =0x0A16\nDESCRIP  =Параметр настройки ПИ-регулятора контура скорости\nMINMAX   =0;60000\nSERVICE  =1\nREADONLY =0\nDEVELOP  =0\nBITS     =32\nSTEP     =12\nMACROS   =0\n---\nNAME     =vp19\nGROUP    =vp\nCAPTION  =Максимальная ошибка\nUNITS    =\nLIST     =\nADDRESS  =0x0A17\nDESCRIP  =Параметр настройки ПИ-регулятора контура скорости\nMINMAX   =0;60000\nSERVICE  =1\nREADONLY =0\nDEVELOP  =0\nBITS     =32\nSTEP     =12\nMACROS   =0\n---\nNAME     =vp20\nGROUP    =vp\nCAPTION  =Ограничение форсирующей связи 1го порядка\nUNITS    =\nLIST     =\nADDRESS  =0x0A18\nDESCRIP  =Параметр настройки ПИ-регулятора контура скорости\nMINMAX   =0;524287\nSERVICE  =1\nREADONLY =0\nDEVELOP  =0\nBITS     =32\nSTEP     =12\nMACROS   =0\n---\nNAME     =vp21\nGROUP    =vp\nCAPTION  =Ограничение форсирующей связи 2го порядка\nUNITS    =\nLIST     =\nADDRESS  =0x0A19\nDESCRIP  =Параметр настройки ПИ-регулятора контура скорости\nMINMAX   =0;524287\nSERVICE  =1\nREADONLY =0\nDEVELOP  =0\nBITS     =32\nSTEP     =12\nMACROS   =0\n---\nNAME     =vp22\nGROUP    =vp\nCAPTION  =Коэффициент форсирующей связи 0го порядка\nUNITS    =\nLIST     =\nADDRESS  =0x0A1A\nDESCRIP  =Параметр настройки ПИ-регулятора контура скорости\nMINMAX   =0;60000\nSERVICE  =1\nREADONLY =0\nDEVELOP  =0\nBITS     =32\nSTEP     =12\nMACROS   =0\n---\nNAME     =vp23\nGROUP    =vp\nCAPTION  =Коэффициент форсирующей связи 1го порядка\nUNITS    =\nLIST     =\nADDRESS  =0x0A1B\nDESCRIP  =Параметр настройки ПИ-регулятора контура скорости\nMINMAX   =0;60000\nSERVICE  =1\nREADONLY =0\nDEVELOP  =0\nBITS     =32\nSTEP     =12\nMACROS   =0\n---\nNAME     =vp24\nGROUP    =vp\nCAPTION  =Коэффициент форсирующей связи 2го порядка\nUNITS    =\nLIST     =\nADDRESS  =0x0A1C\nDESCRIP  =Параметр настройки ПИ-регулятора контура скорости\nMINMAX   =0;60000\nSERVICE  =1\nREADONLY =0\nDEVELOP  =0\nBITS     =32\nSTEP     =12\nMACROS   =0\n---\nNAME     =st9\nGROUP    =st\nCAPTION  =Линейный энкодер\nUNITS    =\nLIST     =0:Нет;1:Да;\nADDRESS  =0x0816\nDESCRIP  =Если параметр установлен в Да, то будет использоваться внешний по отношению к приводу линейный энкодер для замыкания контура позиции. При этом контуры тока и скорости будут работать, по прежнему, от внутреннего энкодера.\nMINMAX   =0;1\nSERVICE  =0\nREADONLY =0\nDEVELOP  =0\nBITS     =16\nSTEP     =\nMACROS   =0\n---\nNAME     =st10\nGROUP    =st\nCAPTION  =Разрешение линейного энкодера\nUNITS    =дискрет\nLIST     =\nADDRESS  =0x0817\nDESCRIP  =Разрешение линейного энкодера на оборот вала двигателя\nMINMAX   =-524286;524286\nSERVICE  =1\nREADONLY =0\nDEVELOP  =0\nBITS     =32\nSTEP     =12\nMACROS   =0\n---\nNAME     =dd30\nGROUP    =dd\nCAPTION  =Разница между внешним и внутренним энкодерами\nUNITS    =дискрет\nLIST     =\nADDRESS  =0x0428\nDESCRIP  =Разница между внешним и внутренним энкодерами с приведением к разрешению внутреннего\nMINMAX   =-524286;524286\nSERVICE  =1\nREADONLY =1\nDEVELOP  =0\nBITS     =32\nSTEP     =12\nMACROS   =0\n---\nNAME     =ss16\nGROUP    =ss\nCAPTION  =Счетчик потерь синхронизации\nUNITS    =\nLIST     =\nADDRESS  =0x0818\nDESCRIP  =Показывает сколько было потеряно команд SYNC=0x02 по шине CAN. Счетчик работает только, если выбран один из возможных режимов синхронизации.\nMINMAX   =0;65535\nSERVICE  =0\nREADONLY =0\nDEVELOP  =0\nBITS     =16\nSTEP     =\nMACROS   =0\n---\nNAME     =ss17\nGROUP    =ss\nCAPTION  =Счетчик потерь команд управления\nUNITS    =\nLIST     =\nADDRESS  =0x0819\nDESCRIP  =Показывает сколько было потеряно команд CAN_POS_COM=0x08 по шине CAN. Счетчик работает только, если выбран один из возможных режимов синхронизации.\nMINMAX   =0;65535\nSERVICE  =0\nREADONLY =0\nDEVELOP  =0\nBITS     =16\nSTEP     =\nMACROS   =0\n---\nNAME     =ss18\nGROUP    =ss\nCAPTION  =Счетчик получения неизвестных команд\nUNITS    =\nLIST     =\nADDRESS  =0x081A\nDESCRIP  =Показывает сколько было получено неизвестных команд по шине CAN, которые помешали прохождению команд управления. Счетчик работает только, если выбран один из возможных режимов синхронизации.\nMINMAX   =0;65535\nSERVICE  =0\nREADONLY =0\nDEVELOP  =0\nBITS     =16\nSTEP     =\nMACROS   =0\n---\nNAME     =pd18\nGROUP    =pd\nCAPTION  =Коэффициент ФНЧ входного сигнала\nUNITS    =\nLIST     =\nADDRESS  =0x0A1D\nDESCRIP  =Параметр настройки ПИД-регулятора\nMINMAX   =0;1\nSERVICE  =1\nREADONLY =0\nDEVELOP  =0\nBITS     =32\nSTEP     =12\nMACROS   =0\n---\nNAME     =pd19\nGROUP    =pd\nCAPTION  =Коэффициент ФНЧ сигнала обратной связи\nUNITS    =\nLIST     =\nADDRESS  =0x0A1E\nDESCRIP  =Параметр настройки ПИД-регулятора\nMINMAX   =0;1\nSERVICE  =1\nREADONLY =0\nDEVELOP  =0\nBITS     =32\nSTEP     =12\nMACROS   =0\n---\nNAME     =ep7\nGROUP    =ep\nCAPTION  =Функция контроля зазора\nUNITS    =\nLIST     =0:ВЫКЛ;90:ВКЛ;\nADDRESS  =0x081B\nDESCRIP  =Включение данной автоматически запускает внутреннюю программу контроля расстояния между инструментом и обрабатываемым листом.\nMINMAX   =0;90\nSERVICE  =0\nREADONLY =0\nDEVELOP  =0\nBITS     =16\nSTEP     =1\nMACROS   =0\n---\nNAME     =pp11\nGROUP    =pp\nCAPTION  =Коэффициент микроинтерполяции\nUNITS    =\nLIST     =1:1;2:2;3:3;4:4;5:5;\nADDRESS  =0x081C\nDESCRIP  =Коэффициент микроинтерполяции определяет кратность соотношения частот квантования СЧПУ и контура позиции привода. Коэффициент может принимать только значения 1, 2, 3, 4, 5. Если коэффициент равен 1, то частоты СЧПУ и привода равны.\nMINMAX   =1;5\nSERVICE  =1\nREADONLY =0\nDEVELOP  =0\nBITS     =32\nSTEP     =10\nMACROS   =0\n---\nNAME     =ip19\nGROUP    =ip\nCAPTION  =Данные CAN собщения 0\nUNITS    =\nLIST     =\nADDRESS  =0x081D\nDESCRIP  =4 младших байта последнего полученного CAN собщения\nMINMAX   =-2147483637;2147483646\nSERVICE  =0\nREADONLY =0\nDEVELOP  =0\nBITS     =32\nSTEP     =\nMACROS   =0\n---\nNAME     =ip20\nGROUP    =ip\nCAPTION  =Данные CAN собщения 1\nUNITS    =\nLIST     =\nADDRESS  =0x081E\nDESCRIP  =4 старших байта последнего полученного CAN собщения\nMINMAX   =-2147483637;2147483646\nSERVICE  =0\nREADONLY =0\nDEVELOP  =0\nBITS     =32\nSTEP     =\nMACROS   =0\n---\nNAME     =dd31\nGROUP    =dd\nCAPTION  =Смещение фазы ослабления поля\nUNITS    =\nLIST     =\nADDRESS  =0x0429\nDESCRIP  =\nMINMAX   =0;0\nSERVICE  =0\nREADONLY =1\nDEVELOP  =0\nBITS     =16\nSTEP     =\nMACROS   =0\n---\nNAME     =vp25\nGROUP    =vp\nCAPTION  =Коэффициент ФНЧ входного сигнала\nUNITS    =\nLIST     =\nADDRESS  =0x081F\nDESCRIP  =Коэффициент ФНЧ входного сигнала контура скорости\nMINMAX   =0;1\nSERVICE  =1\nREADONLY =0\nDEVELOP  =0\nBITS     =32\nSTEP     =12\nMACROS   =0\n---\nNAME     =vp26\nGROUP    =vp\nCAPTION  =Коэффициент ФНЧ сигнала обратной связи\nUNITS    =\nLIST     =\nADDRESS  =0x0820\nDESCRIP  =Коэффициент ФНЧ сигнала обратной связи контура скорости\nMINMAX   =0;1\nSERVICE  =1\nREADONLY =0\nDEVELOP  =0\nBITS     =32\nSTEP     =12\nMACROS   =0\n---\nNAME     =up17\nGROUP    =up\nCAPTION  =Переменная общего назначения 8\nUNITS    =\nLIST     =\nADDRESS  =0x0711\nDESCRIP  =Может использоваться для общих целей. ВНИМАНИЕ! Данная переменная не записывается в энергонезависимую память.\nMINMAX   =-2147483647;2147483647\nSERVICE  =0\nREADONLY =0\nDEVELOP  =0\nBITS     =32\nSTEP     =\nMACROS   =0\n---\nNAME     =up18\nGROUP    =up\nCAPTION  =Переменная общего назначения 9\nUNITS    =\nLIST     =\nADDRESS  =0x0712\nDESCRIP  =Может использоваться для общих целей. ВНИМАНИЕ! Данная переменная не записывается в энергонезависимую память.\nMINMAX   =-2147483647;2147483647\nSERVICE  =0\nREADONLY =0\nDEVELOP  =0\nBITS     =32\nSTEP     =\nMACROS   =0\n---\nNAME     =up19\nGROUP    =up\nCAPTION  =Переменная общего назначения 10\nUNITS    =\nLIST     =\nADDRESS  =0x0713\nDESCRIP  =\nMINMAX   =-2147483647;2147483647\nSERVICE  =0\nREADONLY =0\nDEVELOP  =0\nBITS     =32\nSTEP     =\nMACROS   =0\n---\nNAME     =up20\nGROUP    =up\nCAPTION  =Переменная общего назначения 11\nUNITS    =\nLIST     =\nADDRESS  =0x0714\nDESCRIP  =\nMINMAX   =-2147483647;2147483647\nSERVICE  =0\nREADONLY =0\nDEVELOP  =0\nBITS     =32\nSTEP     =\nMACROS   =0\n---\nNAME     =up21\nGROUP    =up\nCAPTION  =Переменная общего назначения 12\nUNITS    =\nLIST     =\nADDRESS  =0x0715\nDESCRIP  =Может использоваться для общих целей. ВНИМАНИЕ! Данная переменная не записывается в энергонезависимую память.\nMINMAX   =-2147483647;2147483647\nSERVICE  =0\nREADONLY =0\nDEVELOP  =0\nBITS     =32\nSTEP     =\nMACROS   =0\n---\nNAME     =up22\nGROUP    =up\nCAPTION  =Переменная общего назначения 13\nUNITS    =\nLIST     =\nADDRESS  =0x0716\nDESCRIP  =Может использоваться для общих целей. ВНИМАНИЕ! Данная переменная не записывается в энергонезависимую память.\nMINMAX   =-2147483647;2147483647\nSERVICE  =0\nREADONLY =0\nDEVELOP  =0\nBITS     =32\nSTEP     =\nMACROS   =0\n---\nNAME     =up23\nGROUP    =up\nCAPTION  =Переменная общего назначения  14\nUNITS    =\nLIST     =\nADDRESS  =0x0717\nDESCRIP  =Может использоваться для общих целей. ВНИМАНИЕ! Данная переменная не записывается в энергонезависимую память.\nMINMAX   =-2147483647;2147483647\nSERVICE  =0\nREADONLY =0\nDEVELOP  =0\nBITS     =32\nSTEP     =\nMACROS   =0\n---\nNAME     =up24\nGROUP    =up\nCAPTION  =Переменная общего назначения 15\nUNITS    =\nLIST     =\nADDRESS  =0x0718\nDESCRIP  =Может использоваться для общих целей. ВНИМАНИЕ! Данная переменная не записывается в энергонезависимую память.\nMINMAX   =-2147483647;2147483647\nSERVICE  =0\nREADONLY =0\nDEVELOP  =0\nBITS     =32\nSTEP     =\nMACROS   =0\n---\nNAME     =dd32\nGROUP    =dd\nCAPTION  =Задержка синхронизации\nUNITS    =nсек\nLIST     =\nADDRESS  =0x042A\nDESCRIP  =Время между приемом команды упарвления и команды синхронизации. Параметр действителен только для приоводов с интерфейсом упарвления EtherCAT и при активизации управления от СЧПУ.\nMINMAX   =0;0\nSERVICE  =0\nREADONLY =1\nDEVELOP  =0\nBITS     =32\nSTEP     =\nMACROS   =0\n---\nNAME     =cp11\nGROUP    =cp\nCAPTION  =Коэффициент ФНЧ входного сигнала\nUNITS    =\nLIST     =\nADDRESS  =0x0821\nDESCRIP  =Коэффициент ФНЧ входного сигнала контура тока.\nMINMAX   =0;1\nSERVICE  =1\nREADONLY =0\nDEVELOP  =0\nBITS     =32\nSTEP     =12\nMACROS   =0\n---\nNAME     =cp12\nGROUP    =cp\nCAPTION  =Коэффициент ФНЧ сигнала ОС\nUNITS    =\nLIST     =\nADDRESS  =0x0822\nDESCRIP  =Коэффициент ФНЧ сигнала обратной связи контура тока.\nMINMAX   =0;1\nSERVICE  =1\nREADONLY =0\nDEVELOP  =0\nBITS     =32\nSTEP     =12\nMACROS   =0\n---\nNAME     =st11\nGROUP    =st\nCAPTION  =Разрешение на полюс двигателя\nUNITS    =дискрет\nLIST     =\nADDRESS  =0x0823\nDESCRIP  =Формуля для расчета:\nMINMAX   =1000;2098176\nSERVICE  =0\nREADONLY =0\nDEVELOP  =0\nBITS     =32\nSTEP     =\nMACROS   =0\n---\nNAME     =st12\nGROUP    =st\nCAPTION  =Коэффициент деления энкодера\nUNITS    =\nLIST     =\nADDRESS  =0x0824\nDESCRIP  =Уменьшает разрешение датчика позиции (энкодера) в 2 или 4 раза. Если st12=1, то разрешение энкодера не уменьшается и соответствует физическому разрешению, выдаваемому самим датчиком.\nMINMAX   =1;4\nSERVICE  =0\nREADONLY =0\nDEVELOP  =0\nBITS     =16\nSTEP     =\nMACROS   =0\n---\nNAME     =st13\nGROUP    =st\nCAPTION  =Инвертированные сигналы UVW\nUNITS    =\nLIST     =0:Нет;21930:Да;\nADDRESS  =0x0825\nDESCRIP  =UVW треки должны следовать в следующем порядке: 2, 3, 1, 5, 4, 6. Для таких датчиков st13=Нет. В некоторых датчиках сигналы идут с инверсией, в этом случае последовательность: 2, 6, 4, 5, 1, 3. Для таких датчиков st13=Да.\nMINMAX   =-2147483647;2147483647\nSERVICE  =0\nREADONLY =0\nDEVELOP  =0\nBITS     =32\nSTEP     =\nMACROS   =0\n---\nNAME     =dd33\nGROUP    =dd\nCAPTION  =Кол-во импульсов на сектор UVW сигнала\nUNITS    =имп.\nLIST     =\nADDRESS  =0x042B\nDESCRIP  =Кол-во импульсов датчика позиции, приходящееся на текущий сектор UVW сигнала.\nMINMAX   =-2147483647;2147483647\nSERVICE  =0\nREADONLY =1\nDEVELOP  =0\nBITS     =32\nSTEP     =\nMACROS   =0\n---\nNAME     =dd34\nGROUP    =dd\nCAPTION  =Ток в роторной системе координат\nUNITS    =дискрет\nLIST     =\nADDRESS  =0x042C\nDESCRIP  =Ток, пересчитанный в роторную систему координат. Данный сигнал является обратной связью на задание ddd2\nMINMAX   =-2147483647;2147483647\nSERVICE  =1\nREADONLY =1\nDEVELOP  =0\nBITS     =32\nSTEP     =12\nMACROS   =0\n---\nNAME     =st14\nGROUP    =st\nCAPTION  =Автоматический поиск фазы\nUNITS    =\nLIST     =0:Фаза не найдена;170:Запрос поиска фазы;171:Ожидание завершения поиска фазы;172:Ожидаем вращения в +;173:Ожидаем вращения в -;174:Ошибка поиска;175:Поиск выполнен успешно;\nADDRESS  =0x0826\nDESCRIP  =Параметр используется для отображения текущего состояния поиска фазы в автоматическом режиме. Поиск фазы позволяет настроить сервоусилитель на конкретный экземпляр двигателя.\nMINMAX   =0;175\nSERVICE  =0\nREADONLY =1\nDEVELOP  =0\nBITS     =16\nSTEP     =0\nMACROS   =0\n\n//-------------------------------------------------------------\n//МАКРОСЫ\n//-------------------------------------------------------------\nFunctions\n\n\nmacros cp3\n  ON_READ\n  READ cp3\n  cp3=cp3*5/2047\n  RETURN cp3\n  ON_WRITE\n  cp3=val*2047/5\n  WRITE cp3\nend\n\n\nmacros cp4\n  ON_READ\n  READ cp4\n  cp4=cp4*5/2500\n  RETURN cp4\n  ON_WRITE\n  cp4=val*2500/5\n  WRITE cp4\nend\n\n\nmacros vp5 ОТКЛЮЧЕНО\n  ON_READ\n  READ vp5\n  vp5=vp5*2\n  RETURN vp5\n  ON_WRITE\n  vp5=val/2\n  WRITE vp5\nend\n\n\nmacros vp6\n  ON_READ\n  READ vp6\n  if vp4=0\n  READ vp4\n  fi\n  vp6=vp6/vp4\n  RETURN vp6\n  ON_WRITE\n  if vp4=0\n  READ vp4\n  fi\n  vp6=val*vp4\n  WRITE vp6\n  ON_ERROR\n  vp6=100000000000000\n  RETURN vp6\nend\n\n\nmacros vp8 ОТКЛЮЧЕНО\n  ON_READ\n  READ vp8\n  if st1=0\n  READ st1\n  fi\n  if vp4=0\n  READ vp4\n  fi\n  if vp3=0\n  READ vp3\n  fi\n  vp8=round(60*vp8*vp4/(st1*vp3))\n  RETURN vp8\n  ON_WRITE\n  if st1=0\n  READ st1\n  fi\n  if vp4=0\n  READ vp4\n  fi\n  if vp3=0\n  READ vp3\n  fi\n  vp8=val*st1*vp3/(60*vp4)\n  WRITE vp8\n  ON_ERROR\n  vp8=100000000000000\n  RETURN vp8\nend\n\n\nmacros ct1\n  ON_READ\n  READ ct1\n  ct1=ct1*5/2500\n  RETURN ct1\n  ON_WRITE\n  ct1=val*2500/5\n  WRITE ct1\nend\n\n\nmacros ct2 ОТКЛЮЧЕНО\n  ON_READ\n  READ ct2\n  if st1=0\n  READ st1\n  fi\n  if vp4=0\n  READ vp4\n  fi\n  if vp3=0\n  READ vp3\n  fi\n  ct2=round(60*ct2*vp4/(st1*vp3))\n  RETURN ct2\n  ON_WRITE\n  if st1=0\n  READ st1\n  fi\n  if vp4=0\n  READ vp4\n  fi\n  if vp3=0\n  READ vp3\n  fi\n  ct2=val*st1*vp3/(60*vp4)\n  WRITE ct2\nend\n\n\nmacros dd1\n  ON_READ\n  READ dd1\n  dd1=dd1*5/2047\n  RETURN dd1\n  ON_WRITE\n  dd1=val*2047/5\n  WRITE dd1\nend\n\n\nmacros dd6\n  ON_READ\n  READ dd6\n  dd6=dd6*5/2047\n  RETURN dd6\n  ON_WRITE\n  dd6=val*2047/5\n  WRITE dd6\nend\n\n\nmacros dd3\n  ON_READ\n  READ dd3\n  dd3=dd3*5/2047\n  RETURN dd3\n  ON_WRITE\n  dd3=val*2047/5\n  WRITE dd3\nend\n\n\nmacros dd9\n  ON_READ\n  READ dd9\n  dd9=dd9*5/2047\n  RETURN dd9\n  ON_WRITE\n  dd9=val*2047/5\n  WRITE dd9\nend\n\n\nmacros dd2\n  ON_READ\n  READ dd2\n  dd2=dd2*5/2047\n  RETURN dd2\n  ON_WRITE\n  dd2=val*2047/5\n  WRITE dd2\nend\n\n\nmacros dd4 ОТКЛЮЧЕНО\n  ON_READ\n  READ dd4\n  if st1=0\n  READ st1\n  fi\n  if vp4=0\n  READ vp4\n  fi\n  x=round(60*dd4*vp4/st1)\n  RETURN x\n  ON_WRITE\n  dd4=val\n  WRITE dd4\n  ON_STREAM_REQ\n  READ st1\n  READ vp4\n  ON_ERROR\n  dd4=100000000000000\n  RETURN dd4\nend\n\n\nmacros dd5 ОТКЛЮЧЕНО\n  ON_READ\n  READ dd5\n  if st1=0\n  READ st1\n  fi\n  if vp4=0\n  READ vp4\n  fi\n  if vp3=0\n  READ vp3\n  fi\n  dd5=round(60*dd5*vp4/(st1*vp3))\n  RETURN dd5\n  ON_WRITE\n  dd5=val\n  WRITE dd5\n  ON_STREAM_REQ\n  READ st1\n  READ vp4\n  ON_ERROR\n  dd5=100000000000\n  RETURN dd5\nend\n\n\nmacros dd20 ОТКЛЮЧЕНО\n  ON_READ\n  READ dd20\n  dd20=dd20/4096\n  RETURN dd20\n  ON_WRITE\n  dd20=val\n  WRITE dd20\nend\n\n\nmacros dd10\n  ON_READ\n  READ dd10\n  dd10=dd10/128\n  RETURN dd10\n  ON_WRITE\n  dd10=val\n  WRITE dd10\nend\n\n\nmacros dd19\n  ON_READ\n  READ dd19\n  dd19=dd19/178\n  RETURN dd19\n  ON_WRITE\n  dd19=val\n  WRITE dd19\nend\n\n\nmacros dd12\n  ON_READ\n  READ dd12\n  dd12=dd12/21\n  RETURN dd12\n  ON_WRITE\n  dd12=val\n  WRITE dd12\nend\n\n\nmacros tp2 ОТКЛЮЧЕНО\n  ON_READ\n  READ tp2\n  tp2=tp2*25\n  RETURN tp2\n  ON_WRITE\n  tp2=val/25\n  WRITE tp2\n  ON_ERROR\n  err=100000000000\n  RETURN err\nend\n\n\nmacros tp5\n  ON_READ\n  READ tp5\n  tp5=tp5*25\n  RETURN tp5\n  ON_WRITE\n  tp5=val/25\n  WRITE tp5\n  ON_ERROR\n  err=100000000000\n  RETURN err\nend\n\n\nmacros tp6 ОТКЛЮЧЕНО\n  ON_READ\n  READ tp6\n  if st1=0\n  READ st1\n  fi\n  if vp4=0\n  READ vp4\n  fi\n  if vp3=0\n  READ vp3\n  fi\n  tp6=round(60*tp6*vp4/(st1*vp3))\n  RETURN tp6\n  ON_WRITE\n  if st1=0\n  READ st1\n  fi\n  if vp4=0\n  READ vp4\n  fi\n  if vp3=0\n  READ vp3\n  fi\n  tp6=val*st1*vp3/(60*vp4)\n  WRITE tp6\n  ON_ERROR\n  tp6=100000000000000\n  RETURN tp6\nend\n\n\nmacros vp10\n  ON_READ\n  READ vp10\n  if st1=0\n  READ st1\n  fi\n  if vp4=0\n  READ vp4\n  fi\n  if vp3=0\n  READ vp3\n  fi\n  vp10=round(60*vp10*vp4/(st1*vp3))\n  RETURN vp10\n  ON_WRITE\n  if st1=0\n  READ st1\n  fi\n  if vp4=0\n  READ vp4\n  fi\n  if vp3=0\n  READ vp3\n  fi\n  vp10=val*st1*vp3/(60*vp4)\n  WRITE vp10\n  ON_ERROR\n  vp10=100000000000000\n  RETURN vp10\nend\n\n\nmacros vp11\n  ON_READ\n  READ vp11\n  if st1=0\n  READ st1\n  fi\n  if vp4=0\n  READ vp4\n  fi\n  if vp3=0\n  READ vp3\n  fi\n  vp11=round(60*vp11*vp4/(st1*vp3))\n  RETURN vp11\n  ON_WRITE\n  if st1=0\n  READ st1\n  fi\n  if vp4=0\n  READ vp4\n  fi\n  if vp3=0\n  READ vp3\n  fi\n  vp11=val*st1*vp3/(60*vp4)\n  WRITE vp11\n  ON_ERROR\n  vp11=100000000000000\n  RETURN vp11\nend\n\n\nmacros vp12\n  ON_READ\n  READ vp12\n  if st1=0\n  READ st1\n  fi\n  if vp4=0\n  READ vp4\n  fi\n  if vp3=0\n  READ vp3\n  fi\n  vp12=round(60*vp12*vp4/(st1*vp3))\n  RETURN vp12\n  ON_WRITE\n  if st1=0\n  READ st1\n  fi\n  if vp4=0\n  READ vp4\n  fi\n  if vp3=0\n  READ vp3\n  fi\n  vp12=val*st1*vp3/(60*vp4)\n  WRITE vp12\n  ON_ERROR\n  vp12=100000000000000\n  RETURN vp12\nend\n\n\nmacros vp13\n  ON_READ\n  READ vp13\n  if st1=0\n  READ st1\n  fi\n  if vp4=0\n  READ vp4\n  fi\n  if vp3=0\n  READ vp3\n  fi\n  vp13=round(60*vp13*vp4/(st1*vp3))\n  RETURN vp13\n  ON_WRITE\n  if st1=0\n  READ st1\n  fi\n  if vp4=0\n  READ vp4\n  fi\n  if vp3=0\n  READ vp3\n  fi\n  vp13=val*st1*vp3/(60*vp4)\n  WRITE vp13\n  ON_ERROR\n  vp13=100000000000000\n  RETURN vp13\nend\n\n\nmacros vp14\n  ON_READ\n  READ vp14\n  if st1=0\n  READ st1\n  fi\n  if vp4=0\n  READ vp4\n  fi\n  x=round(60*vp14*1000/4000)\n  RETURN x\n  ON_WRITE\n  if st1=0\n  READ st1\n  fi\n  if vp4=0\n  READ vp4\n  fi\n  vp14=val*4000/(60*1000)\n  WRITE vp14\n  ON_STREAM_REQ\n  READ st1\n  READ vp4\n  ON_ERROR\n  dd4=100000000000000\n  RETURN vp14\nend\n\n\nmacros ep2\n  ON_READ\n  READ ep2\n  ep2=ep2/21\n  RETURN ep2\n  ON_WRITE\n  ep2=val*21\n  WRITE ep2\nend\n\n\nmacros dd15\n  ON_READ\n  READ dd15\n  dd15=dd15*25/1000\n  RETURN dd15\n  ON_WRITE\n  dd15=val\n  WRITE dd15\nend\n\n\nmacros dd16\n  ON_READ\n  READ dd16\n  dd16=dd16*25/1000\n  RETURN dd16\n  ON_WRITE\n  dd16=val\n  WRITE dd16\nend\n\n\nmacros cp9 ОТКЛЮЧЕНО\n  ON_READ\n  READ cp3\n  cp3=cp3*5/2047\n  RETURN cp3\n  ON_WRITE\n  cp3=val*66\n  WRITE cp3\nend\n\n\nmacros cp10\n  ON_READ\n  READ cp3\n  cp3=cp3*5/2047\n  RETURN cp3\n  ON_WRITE\n  cp3=val*66\n  WRITE cp3\nend\n\n\nmacros dd27\n  ON_READ\n  READ dd1\n  dd1=dd1*5/2047\n  RETURN dd1\n  ON_WRITE\n  dd1=val*2047/5\n  WRITE dd1\nend\n\n\nmacros dd28\n  ON_READ\n  READ dd6\n  dd6=dd6/74\n  RETURN dd6\n  ON_WRITE\n  dd6=val*74\n  WRITE dd6\nend\n\n\nmacros dd29\n  ON_READ\n  READ dd1\n  dd1=dd1/74\n  RETURN dd1\n  ON_WRITE\n  dd1=val*74\n  WRITE dd1\nend\n\n\nmacros dd30 ОТКЛЮЧЕНО\n  ON_READ\n  READ dd1\n  dd1=dd1/74\n  RETURN dd1\n  ON_WRITE\n  dd1=val*74\n  WRITE dd1\nend\n\n\nmacros dd31 ОТКЛЮЧЕНО\n  ON_READ\n  READ vp14\n  if st1=0\n  READ st1\n  fi\n  if vp4=0\n  READ vp4\n  fi\n  x=round(60*vp14*vp4/4000)\n  RETURN x\n  ON_WRITE\n  if st1=0\n  READ st1\n  fi\n  if vp4=0\n  READ vp4\n  fi\n  vp14=val*4000/(60*vp4)\n  WRITE vp14\n  ON_STREAM_REQ\n  READ st1\n  READ vp4\n  ON_ERROR\n  dd4=100000000000000\n  RETURN vp14\nend\n\n"
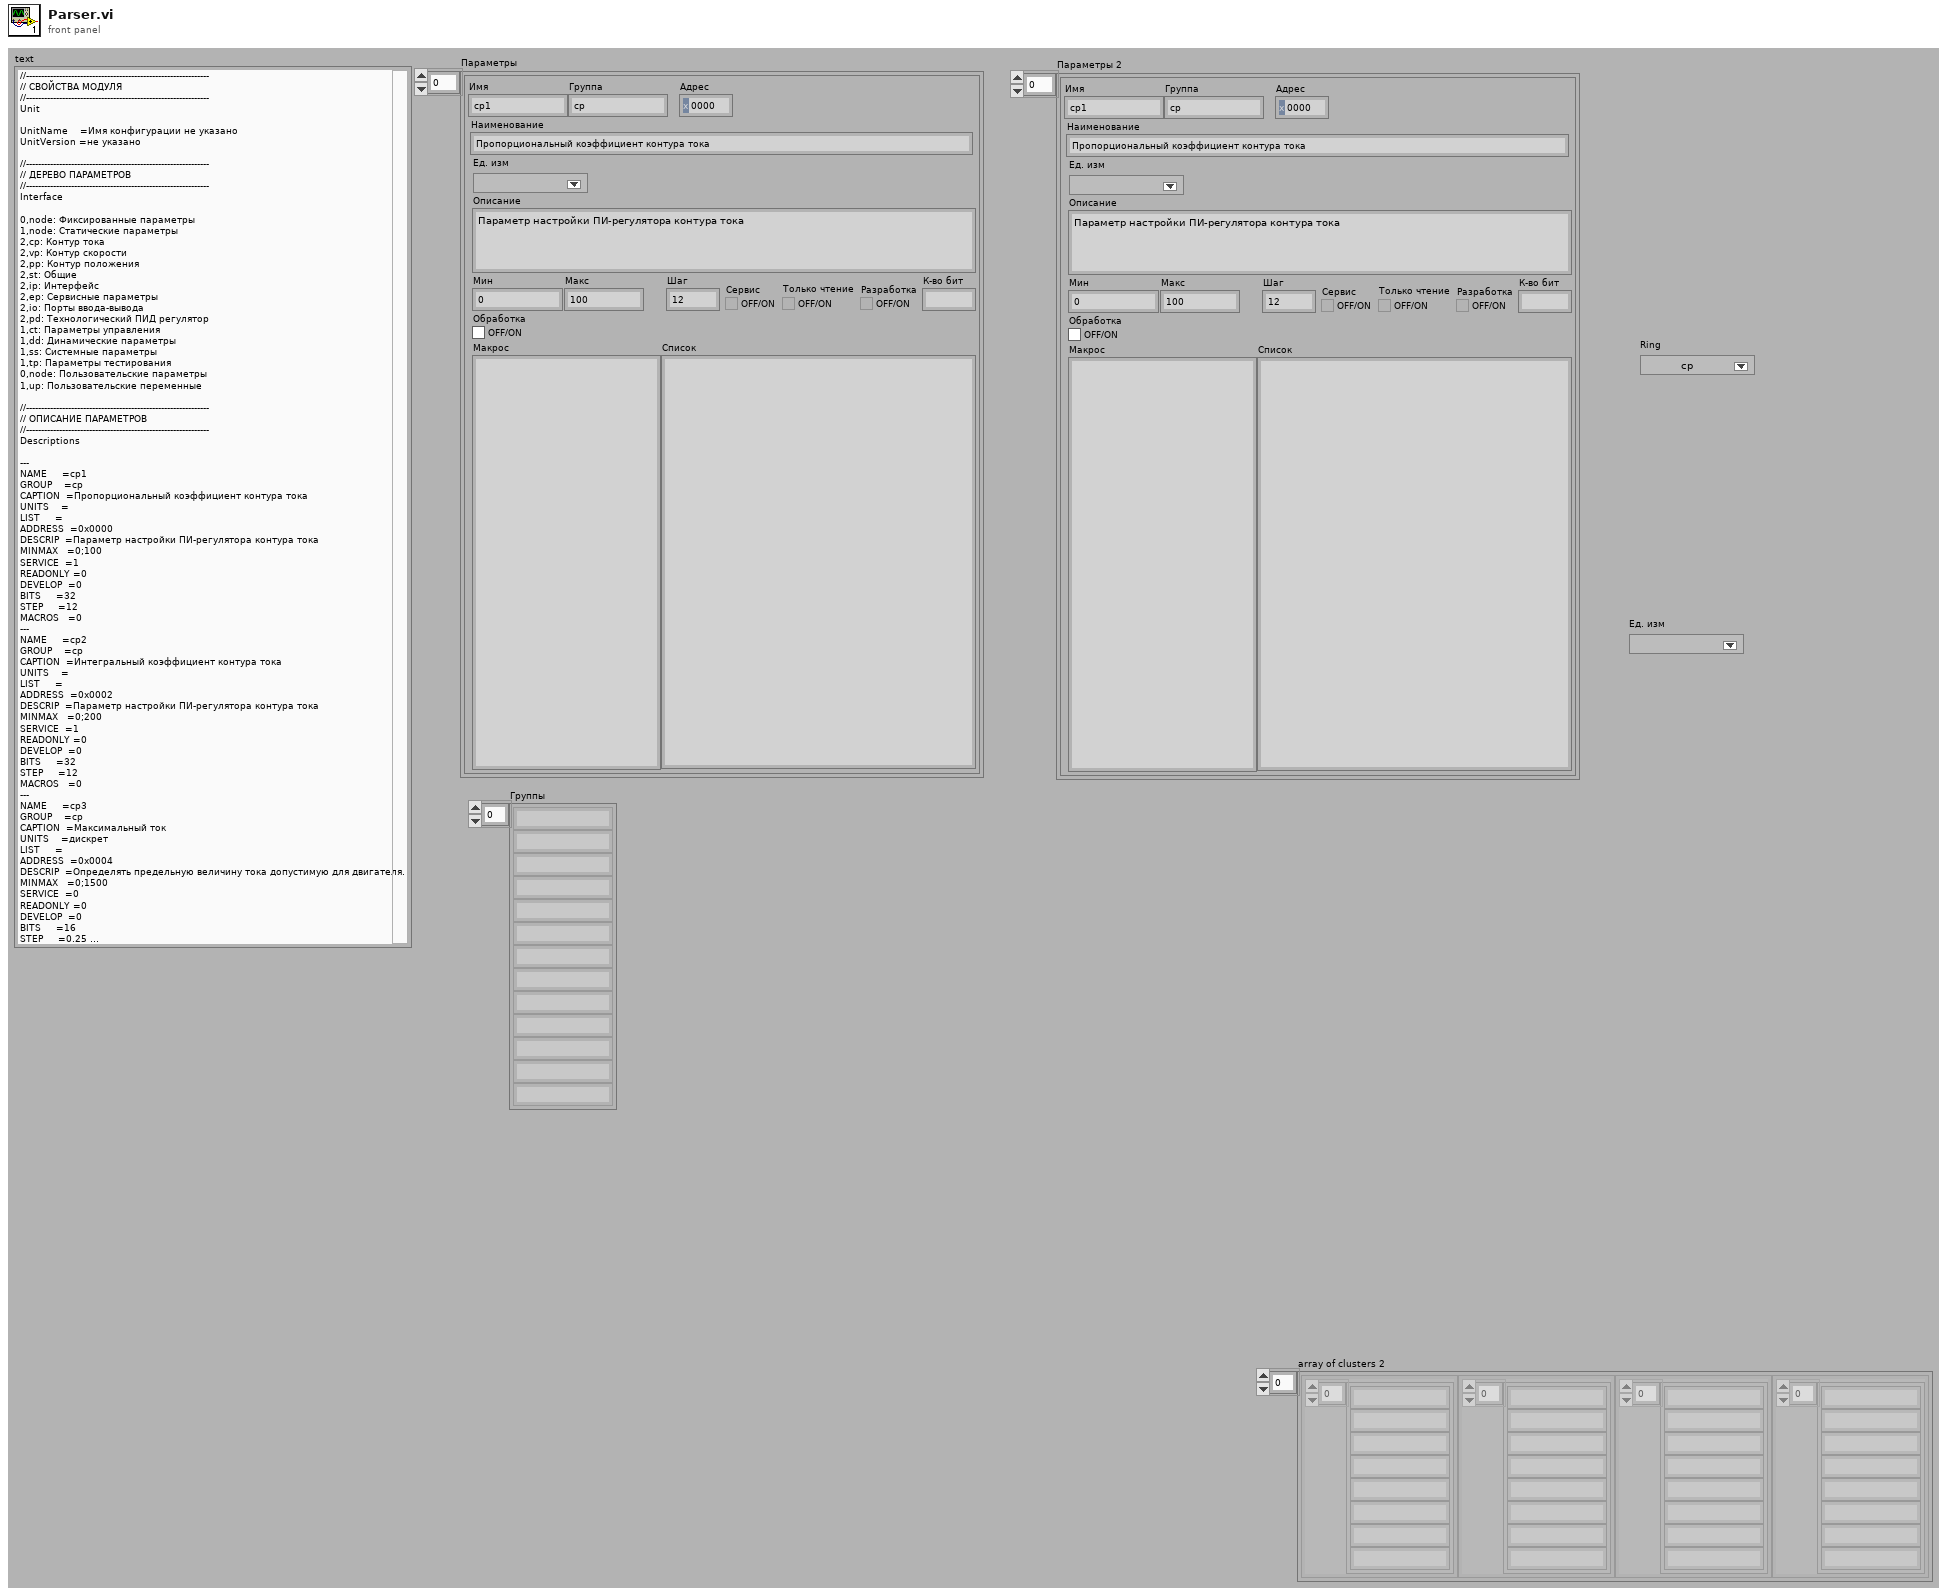
[diagram p1: front panel]
types:
  T1 = cluster{"Имя":string, "Группа":string, "Наименование":string, "Ед. изм":u16, "Список":string, "Адрес":u16, "Описание":string, "Мин":i32, "Макс":i32, "Сервис":bool, "Только чтение":bool, "Разработка":bool, "К-во бит":u16, "Шаг":u32, "Обработка":bool, "Макрос":string}[]
  T2 = cluster{"Имя":string, "Группа":string, "Наименование":string, "Ед. изм":u16, "Список":string, "Адрес":u16, "Описание":string, "Мин":i32, "Макс":i32, "Сервис":bool, "Только чтение":bool, "Разработка":bool, "К-во бит":u16, "Шаг":u32, "Обработка":bool, "Макрос":string}
  T3 = cluster{"[0]":string, "[1]":string, "[2]":string, "[3]":string, "[4]":string, "[5]":string, "[6]":string, "[7]":string, "[8]":string, "[9]":string, "[10]":string, "[11]":string, "[12]":string, "[13]":string}
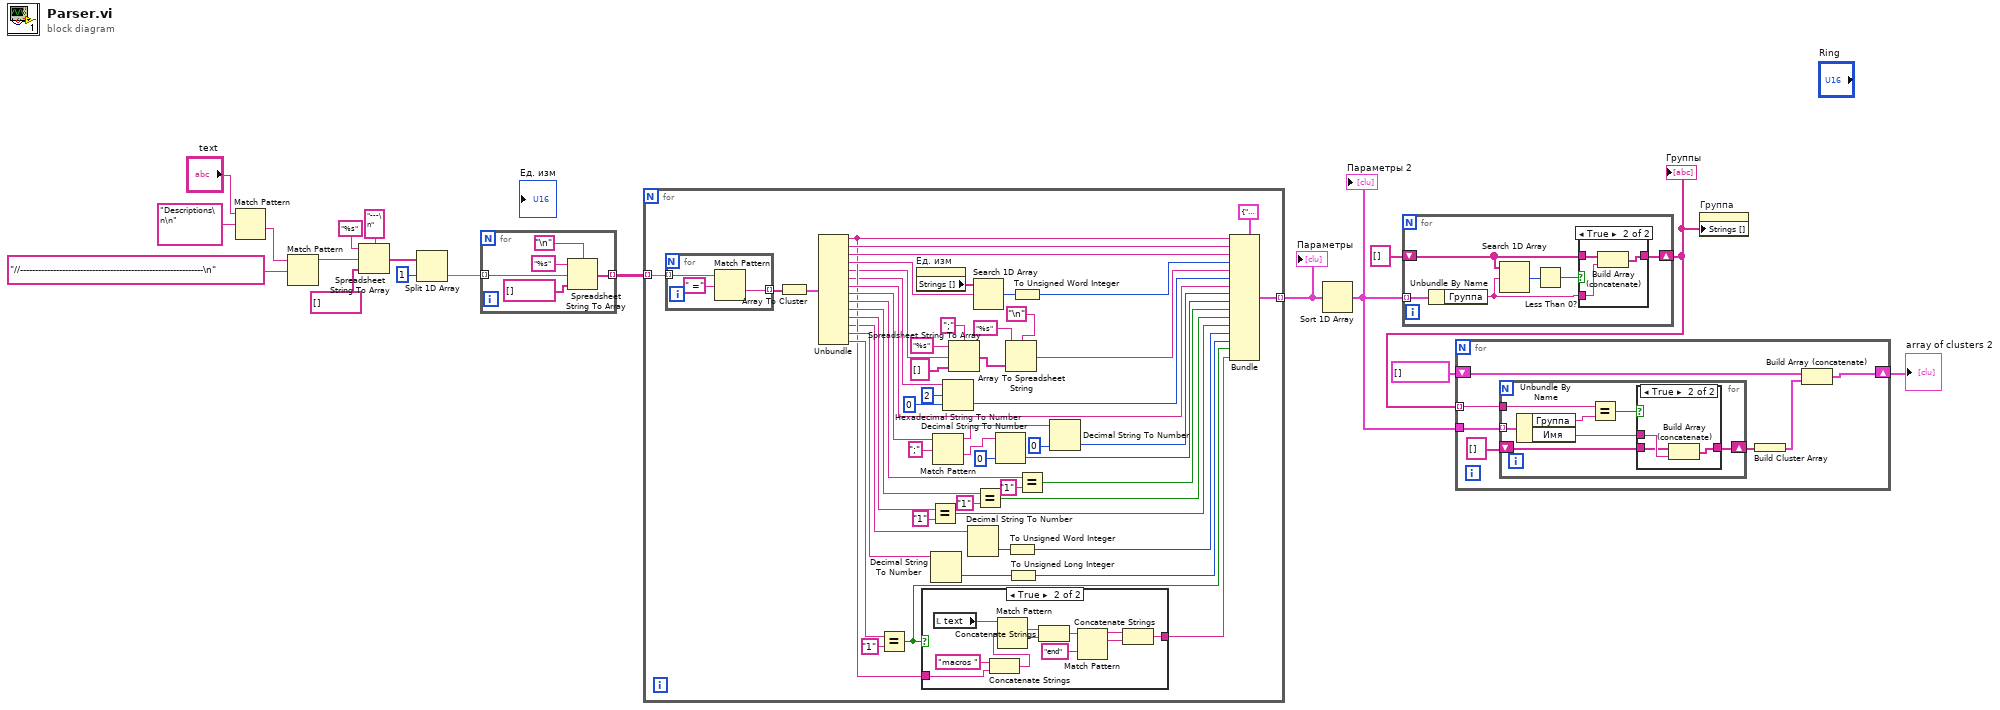
[diagram p0: block diagram]
diagram:
  n1 = Match Pattern(string="text", regular expression="Descriptions\n\n") -> (after substring=w11:string)  [unwired: 1 in, 3 out]
  n2 = Match Pattern(string=w11, regular expression="//-------------------------------------------------------------\n") -> (before substring=w14:string)  [unwired: 1 in, 3 out]
  n3 = Spreadsheet String To Array(delimiter (Tab)="---\n", format string="%s", spreadsheet string=w14, array type (2D Dbl)=string[] []) -> (array=w10:string[])
  n4 = Split 1D Array(array=w10, index=1) -> (second subarray=w8:string[])  [unwired: 1 out]
  n5 = for {
    tunnel: w8 -> [w22] mode=indexing
    tunnel: [w20] -> w7 mode=indexing
    n6 = Spreadsheet String To Array(delimiter (Tab)="\n", format string="%s", spreadsheet string=w22, array type (2D Dbl)=string[] []) -> (array=w20:string[])
  }
  n7 = for {
    tunnel: w7 -> [w75] mode=indexing
    tunnel: [w49] -> w6 mode=indexing
    n8 = for {
      tunnel: w75 -> [w87] mode=indexing
      tunnel: [w88] -> w74 mode=indexing
      n9 = Match Pattern(string=w87, regular expression=" =") -> (after substring=w88:string)  [unwired: 1 in, 3 out]
    }
    n10 = Array To Cluster(array=w74) -> (cluster=w73:T3)
    n11 = Unbundle(w73) -> ("[0]"=w47:string, "[1]"=w68:string, "[2]"=w67:string, "[3]"=w71:string, "[4]"=w36:string, "[5]"=w44:string, "[6]"=w52:string, "[7]"=w50:string, "[8]"=w62:string, "[9]"=w60:string, "[10]"=w58:string, "[11]"=w40:string, "[12]"=w54:string, "[13]"=w66:string)
    n12 = Equal?(x=w66, y="1") -> (x = y?=w48:bool)
    n13 = property on="Ед. изм" class="Ring (strict)"() -> ("Strings []"=w72:string[])  [unwired: 2 in, 2 out]
    n14 = case shown="True" w48 {
      tunnel: w47 -> [_ w85]
      tunnel: [_ w76] -> w46
      frame False {
      }
      frame True {
        n15 = local read "text"() -> (w84:string)
        n16 = Concatenate Strings("macros " ("string"), w85) -> (w83:string)
        n17 = Match Pattern(string=w84, regular expression=w83) -> (match substring=w82:string, after substring=w81:string)  [unwired: 1 in, 2 out]
        n18 = Concatenate Strings(w82, w81) -> (w80:string)
        n19 = Match Pattern(string=w80, regular expression="end") -> (before substring=w78:string, match substring=w77:string)  [unwired: 1 in, 2 out]
        n20 = Concatenate Strings(w78, w77) -> (w76:string)
      }
    }
    n21 = Equal?(x=w58, y="1") -> (x = y?=w57:bool)
    n22 = Decimal String To Number(string=w54) -> (number=w38:i32)  [unwired: 2 in, 1 out]
    n23 = Match Pattern(string=w50, regular expression=";") -> (before substring=w26:string, after substring=w24:string)  [unwired: 1 in, 2 out]
    n24 = Hexadecimal String To Number(string=w44, offset=2, default (0uL)=u16 0 ("default (0 U32)")) -> (number=w43:u16)  [unwired: 1 out]
    n25 = Spreadsheet String To Array(delimiter (Tab)=";" ("format string"), format string="%s", spreadsheet string=w36, array type (2D Dbl)=string[] []) -> (array=w33:string[])
    n26 = Decimal String To Number(string=w40) -> (number=w39:i32)  [unwired: 2 in, 1 out]
    n27 = Search 1D Array(1D array=w72, element=w71) -> (index of element=w70:i32)  [unwired: 1 in]
    n28 = Equal?(x=w60, y="1") -> (x = y?=w59:bool)
    n29 = Decimal String To Number(string=w24, default (0L)=0 ("default (0 U32)")) -> (number=w25:i32)  [unwired: 1 in, 1 out]
    n30 = Array To Spreadsheet String(delimiter (Tab)="\n", array=w33, 3:"%s" ("format string")) -> (spreadsheet string=w30:string)
    n31 = To Unsigned Word Integer(number=w39) -> (unsigned 16bit integer=w55:u16)
    n32 = To Unsigned Long Integer(number=w38) -> (unsigned 32bit integer=w53:u32)
    n33 = To Unsigned Word Integer(number=w70) -> (unsigned 16bit integer=w69:u16)
    n34 = Equal?(x=w62, y="1") -> (x = y?=w61:bool)
    n35 = Decimal String To Number(string=w26, default (0L)=0 ("default (0 U32)")) -> (number=w28:i32)  [unwired: 1 in, 1 out]
    n36 = Bundle(cluster=T2 {"Имя"="", "Группа"="", "Наименование"="", "Ед. изм"=0, "Список"="", "Адрес"=0, "Описание"="", "Мин"=0, "Макс"=0, "Сервис"=FALSE, "Только чтение"=FALSE, "Разработка"=FALSE, "К-во бит"=0, "Шаг"=0, "Обработка"=FALSE, "Макрос"=""}, "Имя"=w47, "Группа"=w68, "Наименование"=w67, "Ед. изм"=w69, "Список"=w30, "Адрес"=w43, "Описание"=w52, "Мин"=w28, "Макс"=w25, "Сервис"=w61, "Только чтение"=w59, "Разработка"=w57, "К-во бит"=w55, "Шаг"=w53, "Обработка"=w48, "Макрос"=w46) -> (w49:T2)
  }
  "Параметры" <- w6
  n37 = Sort 1D Array(array=w6) -> (sorted array=w4:T1)
  "Параметры 2" <- w4
  n38 = for {
    tunnel: w4 -> [w95] mode=indexing
    shift-right: [w91] -> w3
    shift-left: string[] [] -> [w92]
    n39 = Unbundle By Name(w95) -> ("Группа"=w90:string)
    n40 = Search 1D Array(1D array=w92, element=w90) -> (index of element=w94:i32)  [unwired: 1 in]
    n41 = Less Than 0?(x=w94) -> (x < 0?=w93:bool)
    n42 = case shown="True" w93 {
      tunnel: w92 -> [w96 w99]
      tunnel: [w96 w98] -> w91
      tunnel: w90 -> [_ w97]
      frame False {
      }
      frame True {
        n43 = Build Array (concatenate)(w99, w97) -> (w98:string[])
      }
    }
  }
  "Группы" <- w3
  n44 = for {
    tunnel: w3 -> [w105] mode=indexing
    tunnel: w4 -> [w106]
    shift-right: [w100] -> w1
    shift-left: cluster{string[]}[] [] ("array of clusters") -> [w101]
    n45 = for {
      tunnel: w106 -> [w113] mode=indexing
      tunnel: w105 -> [w111]
      shift-right: [w107] -> w103
      shift-left: string[] [] -> [w108]
      n46 = Unbundle By Name(w113) -> ("Группа"=w112:string, "Имя"=w109:string)
      n47 = Equal?(x=w111, y=w112) -> (x = y?=w110:bool)
      n48 = case shown="True" w110 {
        tunnel: w109 -> [_ w117]
        tunnel: w108 -> [w114 w116]
        tunnel: [w114 w115] -> w107
        frame False {
        }
        frame True {
          n49 = Build Array (concatenate)(w116, w117) -> (w115:string[])
        }
      }
    }
    n50 = Build Cluster Array(w103) -> (w102:cluster{string[]}[])
    n51 = Build Array (concatenate)(w101, w102) -> (w100:cluster{string[]}[])
  }
  "array of clusters 2" <- w1
  n52 = property on="Группа" class="Ring (strict)"("Strings []"=w3) -> ()  [unwired: 2 in, 2 out]
